vi "myRIO_BRig_RT_v0,83__PortC.vi"() -> ()   [LabVIEW 2014]
uses:
  myRIO_BRig_RT__Case_Exp_stateList.ctl
  myRIO_BRig_RT__Case_NonExp_stateList.ctl
  <vilib>/Platform/TimedLoop/XDataNode/timing_clust.ctl
  <vilib>/Platform/TimedLoop/XDataNode/nitl_modes.ctl
  <vilib>/Platform/TimedLoop/XDataNode/wakeup.ctl
  <vilib>/WebDAVClient/Advanced/SessionHandle.ctl
  <vilib>/myRIO/Common/Instrument Driver Framework/myRIO v1.0/UART/vis/myRIO v1.0 Close UART.vi
  <vilib>/FPGAPlugInAG/myRIO-1900/niLvFpga_Open_myRIO-1900.vi
  <vilib>/rvi/interface/common/dynamic/niFpgaDynamicAddResources.vi
  <vilib>/Utility/error.llb/Error Cluster From Error Code.vi
  <vilib>/rvi/errors/niLvFpgaAdjustHostInterfaceError.vi
  <vilib>/FPGAPlugInAG/Dynamic/niLvFpga_Close_Dynamic.vi
  <vilib>/myRIO/Common/Instrument Driver Framework/Utilities/vis/FPGA Ref Manager.vi
  <vilib>/myRIO/Common/Instrument Driver Framework/myRIO v1.0/myRIO v1.0 Reset FPGA.vi
  <vilib>/myRIO/Common/Instrument Driver Framework/myRIO v1.0/IRQ/vis/myRIO v1.0 IRQ Info FGV.vi
  <vilib>/myRIO/Common/Instrument Driver Framework/myRIO v1.0/IRQ/vis/myRIO v1.0 Timer IRQ Info FGV.vi
  <vilib>/myRIO/Common/Instrument Driver Framework/myRIO v1.0/IRQ/vis/myRIO v1.0 ISR Agent.vi
  <vilib>/rvi/interface/nirviOpenFPGA/nirviOpenFPGA.xnode
  myRIO_BRig_FPGA_v3,80__PortC__build.lvbitx
  myRIO_BRig_FPGA_v3,80__PortC.vi
  <vilib>/rvi/interface/nirviReadWriteControl/nirviReadWriteControl.xnode
  <vilib>/Platform/TimedLoop/XDataNode/XDataNode.xnode
  <vilib>/rvi/interface/nirviCloseFPGA/nirviCloseFPGA.xnode
  <vilib>/Platform/TimedLoop/XDataNode/XDNodeRunTimeDep.lvlib
  <vilib>/rvi/interface/Simulation/niFpgaSimulationCallBeginRW.vi
  <vilib>/myRIO/Instrument Drivers/Utilities/Utilities.lvlib
  <vilib>/WebDAVClient/NI_WebDAV.lvlib
  NiFpgaLv.dll
panel:
  out "allReward_R":bool
  out "allReward_L":bool
  in  "I_allReward":bool caption="NonSpecific Lick Direction"
  in  "Tcycle_Reward_max_R":u16=1000 caption="Max" min=5 max=5000 step=5
  in  "Tcycle_Reward_min_R":u16=1000 caption="Min" min=5 max=5000 step=5
  in  "Tcycle_Reward_step_R":u16=1000 caption="Penalty" min=1 max=10000 step=1
  in  "Tcycle_Reward_max_L":u16=1000 caption="Max" min=5 max=5000 step=5
  in  "Tcycle_Reward_min_L":u16=1000 caption="Min" min=5 max=5000 step=5
  in  "Tcycle_Reward_step_L":u16=1000 caption="Penalty" min=1 max=10000 step=1
  in  "MTrig_CueLed":bool
  out "Threshold":bool
  out "tLoop":dbl
  in  "Tcycle_Cue_LED_max":u16=1000 caption="Max" min=5 max=5000 step=5
  in  "Tcycle_Cue_LED_min":u16=1000 caption="Min" min=5 max=5000 step=5
  in  "Tcycle_CuePenalty_LED":u16=1000 caption="Penalty" min=1 max=10000 step=1
  out "power_l2":dbl
  in  "MTrig_Laser_Switch":bool
  in  "Cue1Param_AudioLed_Count_NS":u16
  in  "Cue1Param_AudioLed_Count_Switch":u16
  in  "Cue1Param_AudioLed_Probability_NS":u16
  in  "Cue1Param_CueType_NS":u16(slide) max=2 step=1 scale=0.0..2.0
  in  "Cue1Param_AudioLed_Probability_Switch":u16
  in  "Cue1Param_CueType_Switch":u16(slide) max=2 step=1 scale=0.0..2.0
  in  "CueLed_Freq":dbl=10.0
  in  "CueLed_Tpeak":dbl=2.0
  in  "Laser_power_step_l2":dbl
  in  "Laser_power_max_l2":dbl
  in  "Laser_power_min_l2":dbl
  in  "Laser_Tshutter_l2":dbl=2.0
  in  "Laser_Freq_l2":dbl=10.0
  in  "Laser_Tpeak_l2":dbl=2.0
  in  "Laser_duration_l2":u16
  in  "LC_Sel_Count_NS_l2":u16
  in  "LC_Sel_Count_Switch_l2":u16
  in  "LC_Sel_Probability_NS_l2":u16
  in  "LC_Sel_Block_NS_l2":u16(slide) max=2 step=1 scale=0.0..2.0
  in  "LC_Sel_OnOff_NS_l2":bool
  in  "LC_Sel_Probability_Switch_l2":u16
  in  "LC_Sel_Block_Switch_l2":u16(slide) max=2 step=1 scale=0.0..2.0
  in  "LC_Sel_OnOff_Switch_l2":bool
  in  "LC_Sel_Tdelay_NS_l2":u16
  in  "LC_Sel_Tdelay_Switch_l2":u16
  in  "LC_Cue1_Count_NS_l2":u16
  in  "LC_Cue1_Count_Switch_l2":u16
  in  "LC_Cue1_delayOpt_NS_l2":bool
  in  "LC_ENL1_delayOpt_NS_l2":bool
  in  "LC_ENL1_Count_NS_l2":u16
  in  "LC_ENL1_Count_Switch_l2":u16
  in  "LC_Cue1_delayOpt_Switch_l2":bool
  in  "LC_ENL1_delayOpt_Switch_l2":bool
  in  "LC_Cue1_Probability_NS_l2":u16
  in  "LC_Cue1_Block_NS_l2":u16(slide) max=2 step=1 scale=0.0..2.0
  in  "LC_Cue1_OnOff_NS_l2":bool
  in  "LC_Cue1_Probability_Switch_l2":u16
  in  "LC_Cue1_Block_Switch_l2":u16(slide) max=2 step=1 scale=0.0..2.0
  in  "LC_Cue1_OnOff_Switch_l2":bool
  in  "LC_ENL1_Probability_NS_l2":u16 max=100 step=1
  in  "LC_ENL1_Block_NS_l2":u16(slide) max=2 step=1 scale=0.0..2.0
  in  "LC_ENL1_OnOff_NS_l2":bool
  in  "LC_ENL1_Probability_Switch_l2":u16 max=100 step=1
  in  "LC_ENL1_Block_Switch_l2":u16(slide) max=2 step=1 scale=0.0..2.0
  in  "LC_Cue1_Tdelay_NS_l2":u16
  in  "LC_ENL1_Tdelay_NS_l2":u16
  in  "LC_Cue1_Tdelay_Switch_l2":u16
  in  "LC_ENL1_Tdelay_Switch_l2":u16
  in  "LC_ENL1_OnOff_Switch_l2":bool
  in  "LC_Wrong_Probability_l2":u16
  in  "LC_Wrong_Trial_l2":u16(slide) max=2 step=1 scale=0.0..2.0
  in  "LC_Wrong_Block_l2":u16(slide) max=2 step=1 scale=0.0..2.0
  in  "LC_Wrong_OnOff_l2":bool
  in  "LC_Reward_Probability_l2":u16
  in  "LC_Reward_Trial_l2":u16(slide) max=2 step=1 scale=0.0..2.0
  in  "LC_Reward_Block_l2":u16(slide) max=2 step=1 scale=0.0..2.0
  in  "LC_Reward_OnOff_l2":bool
  in  "LC_Wrong_Tdelay_l2":u16
  in  "LC_Reward_Tdelay_l2":u16
  in  "LC_Sel_Count_NS_l1":u16
  in  "LC_Sel_Count_Switch_l1":u16
  in  "LC_Sel_Probability_NS_l1":u16
  in  "LC_Sel_Block_NS_l1":u16(slide) max=2 step=1 scale=0.0..2.0
  in  "LC_Sel_OnOff_NS_l1":bool
  in  "LC_Sel_Probability_Switch_l1":u16
  in  "LC_Sel_Block_Switch_l1":u16(slide) max=2 step=1 scale=0.0..2.0
  in  "LC_Sel_OnOff_Switch_l1":bool
  in  "LC_Sel_Tdelay_NS_l1":u16
  in  "LC_Sel_Tdelay_Switch_l1":u16
  out "I_connect_TCP":bool
  in  "get_countPerMS":bool
  in  "count_warmup_R_reset":bool
  in  "count_warmup_L_reset":bool
  out "count_warmup_R":u16
  out "count_warmup_L":u16
  out "SolenoidReward":bool
  in  "SolenoidProbability_L":u16=100 caption="Reward Time [ms]" min=1 max=1000 step=1
  in  "SolenoidProbability_R":u16=100 caption="Reward Time [ms]" min=1 max=1000 step=1
  out "power_l1":dbl caption="LaserPower"
  in  "Laser_power_step_l1":dbl
  in  "Laser_power_max_l1":dbl
  in  "Recording":bool
  in  "Laser_power_min_l1":dbl
  in  "FPGA_count2ms":dbl=159.0
  in  "Laser_Tshutter_l1":dbl=2.0
  in  "Laser_Freq_l1":dbl=10.0
  in  "Laser_Tpeak_l1":dbl=2.0
  in  "Laser_duration_l1":u16
  out "error out":errorcluster
  in  "LC_Cue1_Count_NS_l1":u16
  in  "LC_Cue1_Count_Switch_l1":u16
  in  "LC_Cue1_delayOpt_NS_l1":bool
  in  "LC_ENL1_delayOpt_NS_l1":bool
  in  "LC_ENL1_Count_NS_l1":u16
  in  "LC_ENL1_Count_Switch_l1":u16
  in  "LC_Cue1_delayOpt_Switch_l1":bool
  in  "LC_ENL1_delayOpt_Switch_l1":bool
  in  "Tcycle_Cue_Audio_max":u16=1000 caption="Max" min=5 max=5000 step=5
  in  "Tcycle_Cue_Audio_min":u16=1000 caption="Min" min=5 max=5000 step=5
  in  "SendData":bool
  out "cSpout":enum16{"Left", "Right"}(ring) caption="Left or Right Spout"
  out "A4":u32 caption="LickCounter_Right"
  out "A2":u32 caption="LickCounter_Left"
  in  "LR_wrong_Event":bool
  out "SelectWrong":bool
  out "SelectReward":bool
  in  "Left(F)_or_Right(T)":bool
  in  "ignoreWrong":bool
  in  "SelectionState":bool
  in  "LR_wrong_Laser":bool
  in  "LR_reward_Laser":bool
  in  "LR_reward_Event":bool
  out "nRewards_Right":u16 caption="# Rewards Total (Right)"
  out "nRewards_Left":u16 caption="# Rewards Total (Left)"
  out "nRewards_cur":u16 caption="# Rewards in Current Block"
  out "TpB_target":u16 caption="Target Trials Per Block"
  out "cState_NonExp":T1 caption="WarmUp State"
  out "iBlock":u16 caption="Current Block"
  out "cState":T2 caption="Experimental State"
  out "iTrial":u16 caption="Current Trial"
  in  "warmupType":u8(slide) max=2 step=1 scale=0.0..2.0
  in  "TestConnection":bool
  in  "warmup":bool caption="WarmUp"
  in  "Data Set Prefix":string="Exp1_TM2"
  out "Connected To Host?":bool
  in  "Host Password":string="sabalab"
  in  "Host UserName":string="Test2"
  in  "sp_RightSpout":u16(slide)=2 max=2 step=1 scale=0.0..2.0
  in  "sp_LeftSpout":u16(slide)=2 max=2 step=1 scale=0.0..2.0
  in  "BUR_max":u16 caption="Count Reward Structure  (0 = off)"
  in  "LC_Wrong_Probability_l1":u16
  in  "LC_Wrong_Trial_l1":u16(slide) max=2 step=1 scale=0.0..2.0
  in  "LC_Wrong_Block_l1":u16(slide) max=2 step=1 scale=0.0..2.0
  in  "LC_Wrong_OnOff_l1":bool
  in  "LC_Reward_Probability_l1":u16
  in  "LC_Reward_Trial_l1":u16(slide) max=2 step=1 scale=0.0..2.0
  in  "LC_Reward_Block_l1":u16(slide) max=2 step=1 scale=0.0..2.0
  in  "LC_Reward_OnOff_l1":bool
  in  "LC_Cue1_Probability_NS_l1":u16
  in  "LC_Cue1_Block_NS_l1":u16(slide) max=2 step=1 scale=0.0..2.0
  in  "LC_Cue1_OnOff_NS_l1":bool
  in  "LC_Cue1_Probability_Switch_l1":u16
  in  "LC_Cue1_Block_Switch_l1":u16(slide) max=2 step=1 scale=0.0..2.0
  in  "LC_Cue1_OnOff_Switch_l1":bool
  in  "LC_ENL1_Probability_NS_l1":u16 max=100 step=1
  in  "LC_ENL1_Block_NS_l1":u16(slide) max=2 step=1 scale=0.0..2.0
  in  "LC_ENL1_OnOff_NS_l1":bool
  in  "LC_ENL1_Probability_Switch_l1":u16 max=100 step=1
  in  "LC_ENL1_Block_Switch_l1":u16(slide) max=2 step=1 scale=0.0..2.0
  in  "Tcycle_Timeout":u16=1000 caption="Timeout Time [ms]" min=10 max=10000 step=1
  in  "Tcycle_Wrong":u16=1000 caption="Wrong Time [ms]" min=10 max=10000 step=1
  in  "Tcycle_Selection":u16=1000 caption="Answer Time [ms]" min=1 max=10000 step=1
  in  "Tcycle_RewardPost":u16=1000 caption="Consumption Time [ms]" min=250 max=10000 step=250
  in  "TpB_Max_R":u16=4 caption="Max TrialsPerBlock" min=1 max=12 step=1
  in  "TpB_Min_R":u16=4 caption="Min TrialsPerBlock" min=1 max=12 step=1
  in  "TpB_Max_L":u16=4 caption="Max TrialsPerBlock" min=1 max=12 step=1
  in  "TpB_Min_L":u16=4 caption="Min TrialsPerBlock" min=1 max=12 step=1
  in  "BUR_min":u16 caption="Count Reward Structure\n(0 = off)"
  in  "TrialUntilReward":bool caption="Ignore Wrong Selection"
  in  "CueCycles":u16=1 caption="Cue Structure" min=1 max=1 step=1
  in  "MTrig_Laser_Tcycle":u16=10 caption="Time [ms]"
  in  "MTrig_Laser_trig":bool
  in  "MTrig_Audio_trig__R":bool caption="Trigger Audio"
  in  "MTrig_Audio_trig__L":bool caption="Trigger Audio"
  in  "RewCalib_Trig_R":bool caption="Calibrate_R"
  in  "RewCalib_Trig_L":bool caption="Calibrate_L"
  in  "MTrig_Solenoid_Tcycle__R":u16=300 caption="Time [ms]"
  in  "MTrig_Solenoid_Tcycle__L":u16=300 caption="Time [ms]"
  in  "MTrig_Solenoid_trig__R":bool caption="Solenoid"
  in  "MTrig_Solenoid_trig__L":bool caption="Solenoid"
  in  "STOP_abort":bool caption="Stop LabView\n(Stops myRio and FPGA)"
  in  "STOP_endBlock":bool caption="Stop Experiment\n@ End of Block"
  in  "STOP_endTrial":bool caption="Stop Experiment\n@ End of Trial"
  in  "START":bool caption="Start Experiment"
  in  "Tcycle_CuePenalty_Audio":u16=1000 caption="Penalty" min=1 max=10000 step=1
  in  "Audio_Amp__R":u16=100 caption="Amp"
  in  "Audio_Freq__R":u8=5 caption="Freq [kHz]" max=14 step=1
  in  "Audio_Amp__L":u16=100 caption="Amp"
  in  "Audio_Freq__L":u8=5 caption="Freq [kHz]" max=14 step=1
  in  "LC_Wrong_Tdelay_l1":u16
  in  "LC_Cue1_Tdelay_NS_l1":u16
  in  "LC_ENL1_Tdelay_NS_l1":u16
  in  "LC_Reward_Tdelay_l1":u16
  in  "LC_Cue1_Tdelay_Switch_l1":u16
  in  "LC_ENL1_Tdelay_Switch_l1":u16
  in  "LC_ENL1_OnOff_Switch_l1":bool
  in  "Tcycle_ENLPenalty":u16=100 caption="Penalty" min=10 max=10000 step=10
  in  "Tcycle_ENL_max":u16=1000 caption="Max" min=250 max=10000 step=250
  in  "Tcycle_ENL_min":u16=1000 caption="Min" min=250 max=10000 step=250
  # "Communication (Host PC)"
  # "Recording Rig"
  # "Experimental Run"
  # "Experiment Task Structure"
  # "STOP experiment at"
  # "Min            Max            Penalty"
  # "(1) = Switching\n(2) = Two Choice"
  # "Enforced\nNonLick"
  # "FPGA Count per [ms]"
  # "Cue Audio"
  # "Current State"
  # "Cue LED"
  # "Global Parameters                                                         Trial Parameters"
  # "Selection"
  # "WarmUp"
  # "Reward - Dispense Water"
  # "Left/Right        Give Reward?        Laser Power [V]"
  # "Laser1      Laser2"
  # "Left"
  # "Cue then reward (no lick)\n \nLeft                    Right"
  # "Right"
  # "Min"
  # "Max"
  # "Dispense Water Probability"
  # "Block                   Trial            Target Trials       # Rewards \n                                                            Per Block             Current"
  # "Left"
  # "WarmUp State"
  # "Trial Per Block Structure \n               Left                        Right"
  # "Lick Counter"
  # "Right"
  # "Left           Right"
  # "Reward - Consumption"
  # "Manual Control"
  # "Min"
  # "# Rewards Total\n                                                                  Left                    Right"
  # "Experimental State"
  # "Penalty - Wrong Choice"
  # "Solenoid\n \nLeft              Right"
  # "Speaker\n \nLeft                    Right"
  # "Laser 1  |  Laser 2"
  # "Max"
  # "Penalty - Choice Timeout"
  # "Time\n[ms]"
  # "Time\n[ms]"
  # "Time = Cue Min"
  # "Cue LED"
  # "Power = Min"
  # "Cue1 Control\n                                  Cue Type           LED Probability [%]      Count"
  # "Laser1 Control\n                               On/Off      Block        Probability [%]   Delay [ms]                              Count"
  # "Laser2 Control\n                               On/Off      Block        Probability [%]   Delay [ms]                              Count"
  # "Audio or LED"
  # "Cue 1"
  # "Enforced\nNonLick\n      1"
  # "Enforced\nNonLick\n      1"
  # "from end"
  # "from end"
  # "Switch\nTrial"
  # "Switch\nTrial"
  # "Switch\nTrial"
  # "from start"
  # "from start"
  # "from end"
  # "from end"
  # "NonSwitch\nTrials"
  # "NonSwitch\nTrials"
  # "NonSwitch\nTrials"
  # "from start"
  # "from start"
  # "Cue 1"
  # "Cue 1"
  # "from end"
  # "from end"
  # "Switch\nTrial"
  # "Switch\nTrial"
  # "Cue Audio Parameters"
  # "Cue LED Parameters"
  # "from start"
  # "from start"
  # "Left                  Right"
  # "Frequency\n[Hz]"
  # "Frequency\n[kHz]"
  # "from end"
  # "from end"
  # "NonSwitch\nTrials"
  # "NonSwitch\nTrials"
  # "Timing [ms]\n                    Peak Width"
  # "from start"
  # "from start"
  # "Amp\n(0 - 32,000)"
  # "Selection"
  # "Selection"
  # "from start"
  # "from start"
  # "Switch\nTrial"
  # "Switch\nTrial"
  # "Speaker\nPattern\nDuring Cue"
  # "from start"
  # "from start"
  # "NonSwitch\nTrials"
  # "NonSwitch\nTrials"
  # "Laser1 Parameters"
  # "Laser2 Parameters"
  # "Laser1 Response\n                               On/Off      Block       Trial       Probability [%]   Delay [ms]"
  # "Laser2 Response\n                               On/Off      Block       Trial       Probability [%]   Delay [ms]"
  # "Frequency\n[Hz]"
  # "Frequency\n[Hz]"
  # "Timing [ms]\n Duration     Peak Width   Shutter"
  # "Timing [ms]\n Duration     Peak Width   Shutter"
  # "Selection Reward"
  # "Selection Reward"
  # "Laser Power [V]\nMin          Max              Step"
  # "Laser Power [V]\nMin          Max              Step"
  # "Selection Wrong"
  # "Selection Wrong"
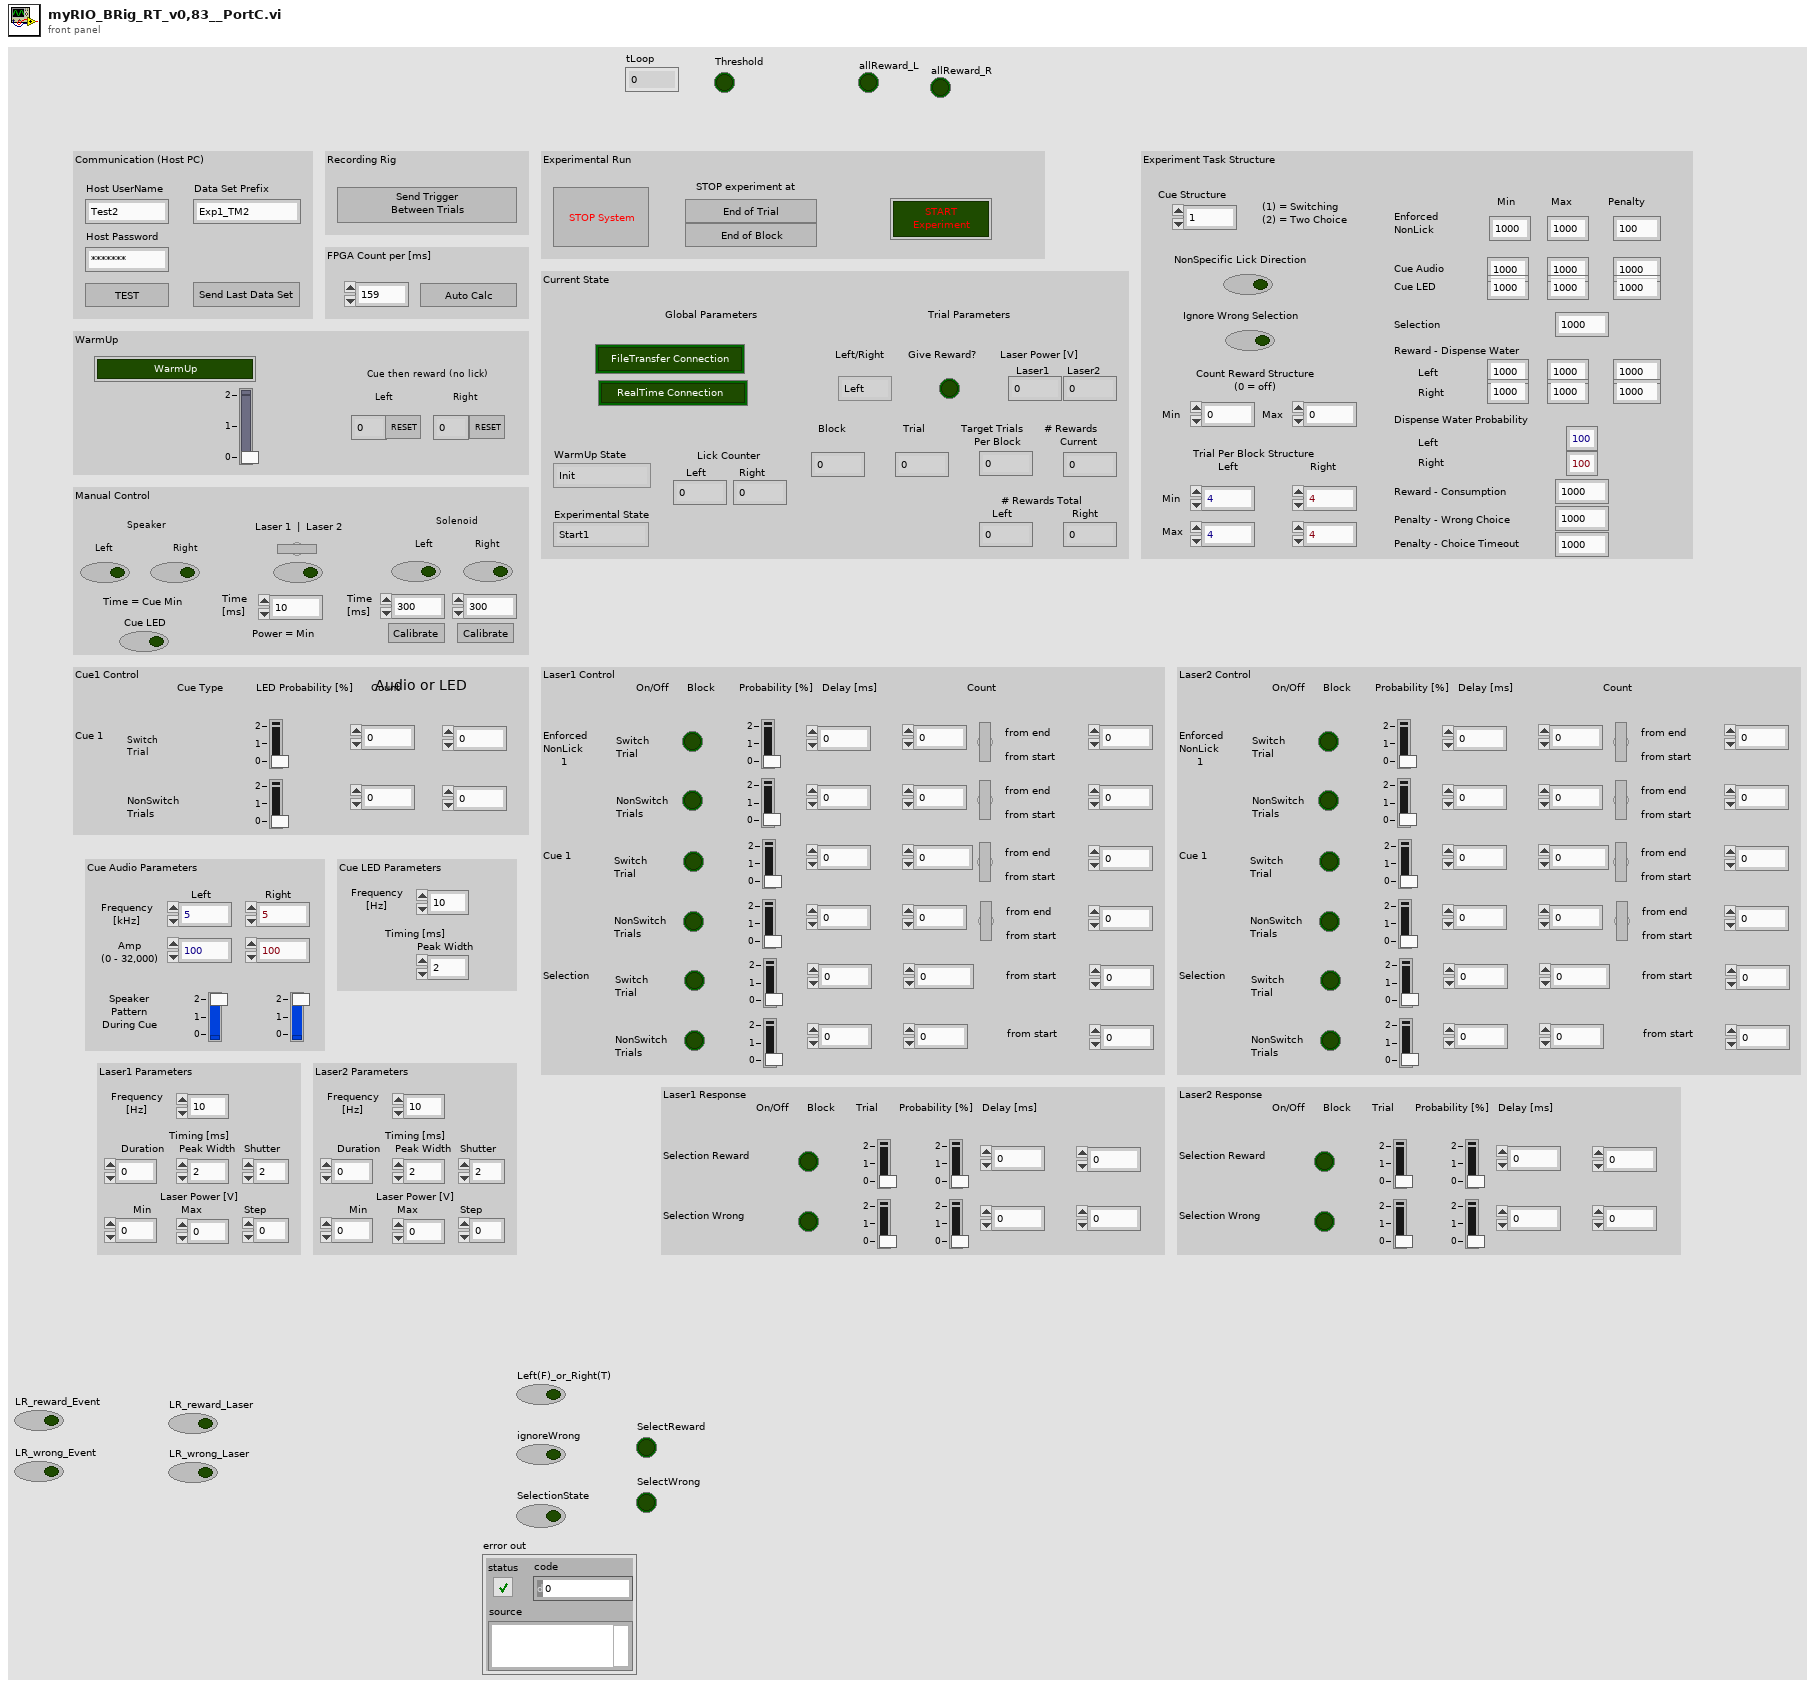
[diagram p1: front panel]
types:
  T1 = typedef "myRIO_BRig_RT__Case_NonExp_stateList.ctl" = enum16{"Init", "UploadSettings_pre", "UploadSettings_Read_dataExp", "UploadSettings_dataExp_1", "UploadSettings_dataExp_2", "UploadSettings_Read_dataLC", "UploadSettings_dataLC_1", "UploadSettings_dataLC_2", "UploadSettings_dataLC_3", "UploadSettings_dataLC_4", "UploadSettings_Read_dataMTrig", "UploadSettings_dataMTrig_1", "UploadSettings_post", "Idle_pre", "IdleEmpty", "IdleEmpty2", "IdleEmpty3", "IdleEmpty4", "Idle", "Idle_2", "Idle_3", "Idle_4", "Idle_5", "Idle_6", "Idle_post", "Cue_pre__pre", "Cue_pre", "Cue", "Cue_LED", "Cue_post", "RewardCalibration_pre", "DispenseWater_pre__pre", "DispenseWater_pre", "DispenseWater", "DispenseWater_post", "TestConnection", "SendData", "Get_FPGA_count_per_ms", "End"}
  T2 = typedef "myRIO_BRig_RT__Case_Exp_stateList.ctl" = enum16{"Start1", "Start2", "Start3", "saveSettings1", "saveSettings2", "saveSettings3", "saveSettings4", "saveSettings_LC_ENL_l1", "saveSettings_LC_ENL_l2", "saveSettings_LC_Cue_l1", "saveSettings_LC_Cue_l2", "saveSettings6_LC_l1_Other", "SaveSettings6_LC_l2_Other", "setSettings_Audio", "setSettings_Laser", "initBlock_pre", "initBlock", "initBlock2", "initBlock_post", "initTrial_pre", "initTrial", "initTrial2", "initTrial3", "initTrial4", "initTrial_LC_ENL1", "initTrial_LC_Cue1", "initTrial_LC_Cue1_2", "initTrial_LC_Sel", "initTrial_post", "ENL1_pre", "ENL1", "ENL1_post", "ENL1Penalty_pre", "ENL1Penalty", "ENL2_pre", "ENL2", "ENL2Penalty_pre", "ENL2Penalty", "Cue1_pre", "Cue1", "Cue1_post", "Cue1Penalty_pre", "Cue1Penalty", "Cue2_pre", "Cue2", "Cue2Penalty_pre", "Cue2Penalty", "Selection_pre", "Selection", "Select_post", "SelectReward_pre", "SelectReward", "SelectRewardPost_pre", "SelectRewardPost", "SelectWrong_pre", "SelectWrong", "SelectWrong_post", "SelectTimeout_pre", "SelectTimeout", "SelectTimeout_post", "endTrial_pre", "endTrial1", "endTrial2", "endTrial3", "endTrial_post", "endBlock_pre", "endBlock", "endBlock_post", "endExp", "commConnect", "commUpload_pre", "commUpload_dataBlock", "commUpload_dataCurrent", "commUpload_dataExp", "commUpload_dataLC", "commUpload_dataTrial", "commUpload_post", "saveData_pre", "saveData_dataBlock", "saveData_dataCurrent", "saveData_dataExp", "saveData_dataLC", "saveData_dataTrial", "saveData_post", "empty_endBlock1", "empty_endBlock2", "empty_endTrial1", "empty_endTrial2", "empty_endTrial3", "empty_endTrial4", "empty_endTrial5", "dummyState", "dummyState_endBlock"}
  T3 = typedef "XDNodeRunTimeDep.lvlib/timing_clust.ctl" = cluster{"Expected End [f-1]":u64, "Actual End [f-1]":u64, "Finished Late? [f-1]":bool, "Expected End [i-1]":u64, "Actual End [i-1]":u64, "Finished Late? [i-1]":bool, "Expected Start [i]":u64, "Actual Start [i]":u64, "Expected Start [f]":u64, "Actual Start [f]":u64, "Source Name":string, "Structure Name":string, "Period":i64, "Deadline":i64, "Offset":i64, "Start":i64, "Priority":i32, "Timeout":i32, "Mode":T4, "Wakeup Reason":T5, "Error":errorcluster, "Source Type":string, "Secondary Source Type":string, "Global End Time":u64, "Global Start Time":u64, "Frame Duration":u64, "Iteration Duration":u64, "Assigned CPU":i32, "I/O Scan Engine Mode":u32}
  T4 = typedef "XDNodeRunTimeDep.lvlib/nitl_modes.ctl" = enum32{"No Change", "Process missed periods, maintain original phase", "Discard missed periods, maintain original phase", "Process missed periods, ignore original phase", "Discard missed periods, ignore original phase"}
  T5 = typedef "XDNodeRunTimeDep.lvlib/wakeup.ctl" = enum32{"Normal", "Aborted", "Asynchronous wakeup", "Timing source error", "Timed loop error", "Timeout"}
  T6 = typedef "NI_WebDAV.lvlib/SessionHandle.ctl" = refnum<k1>
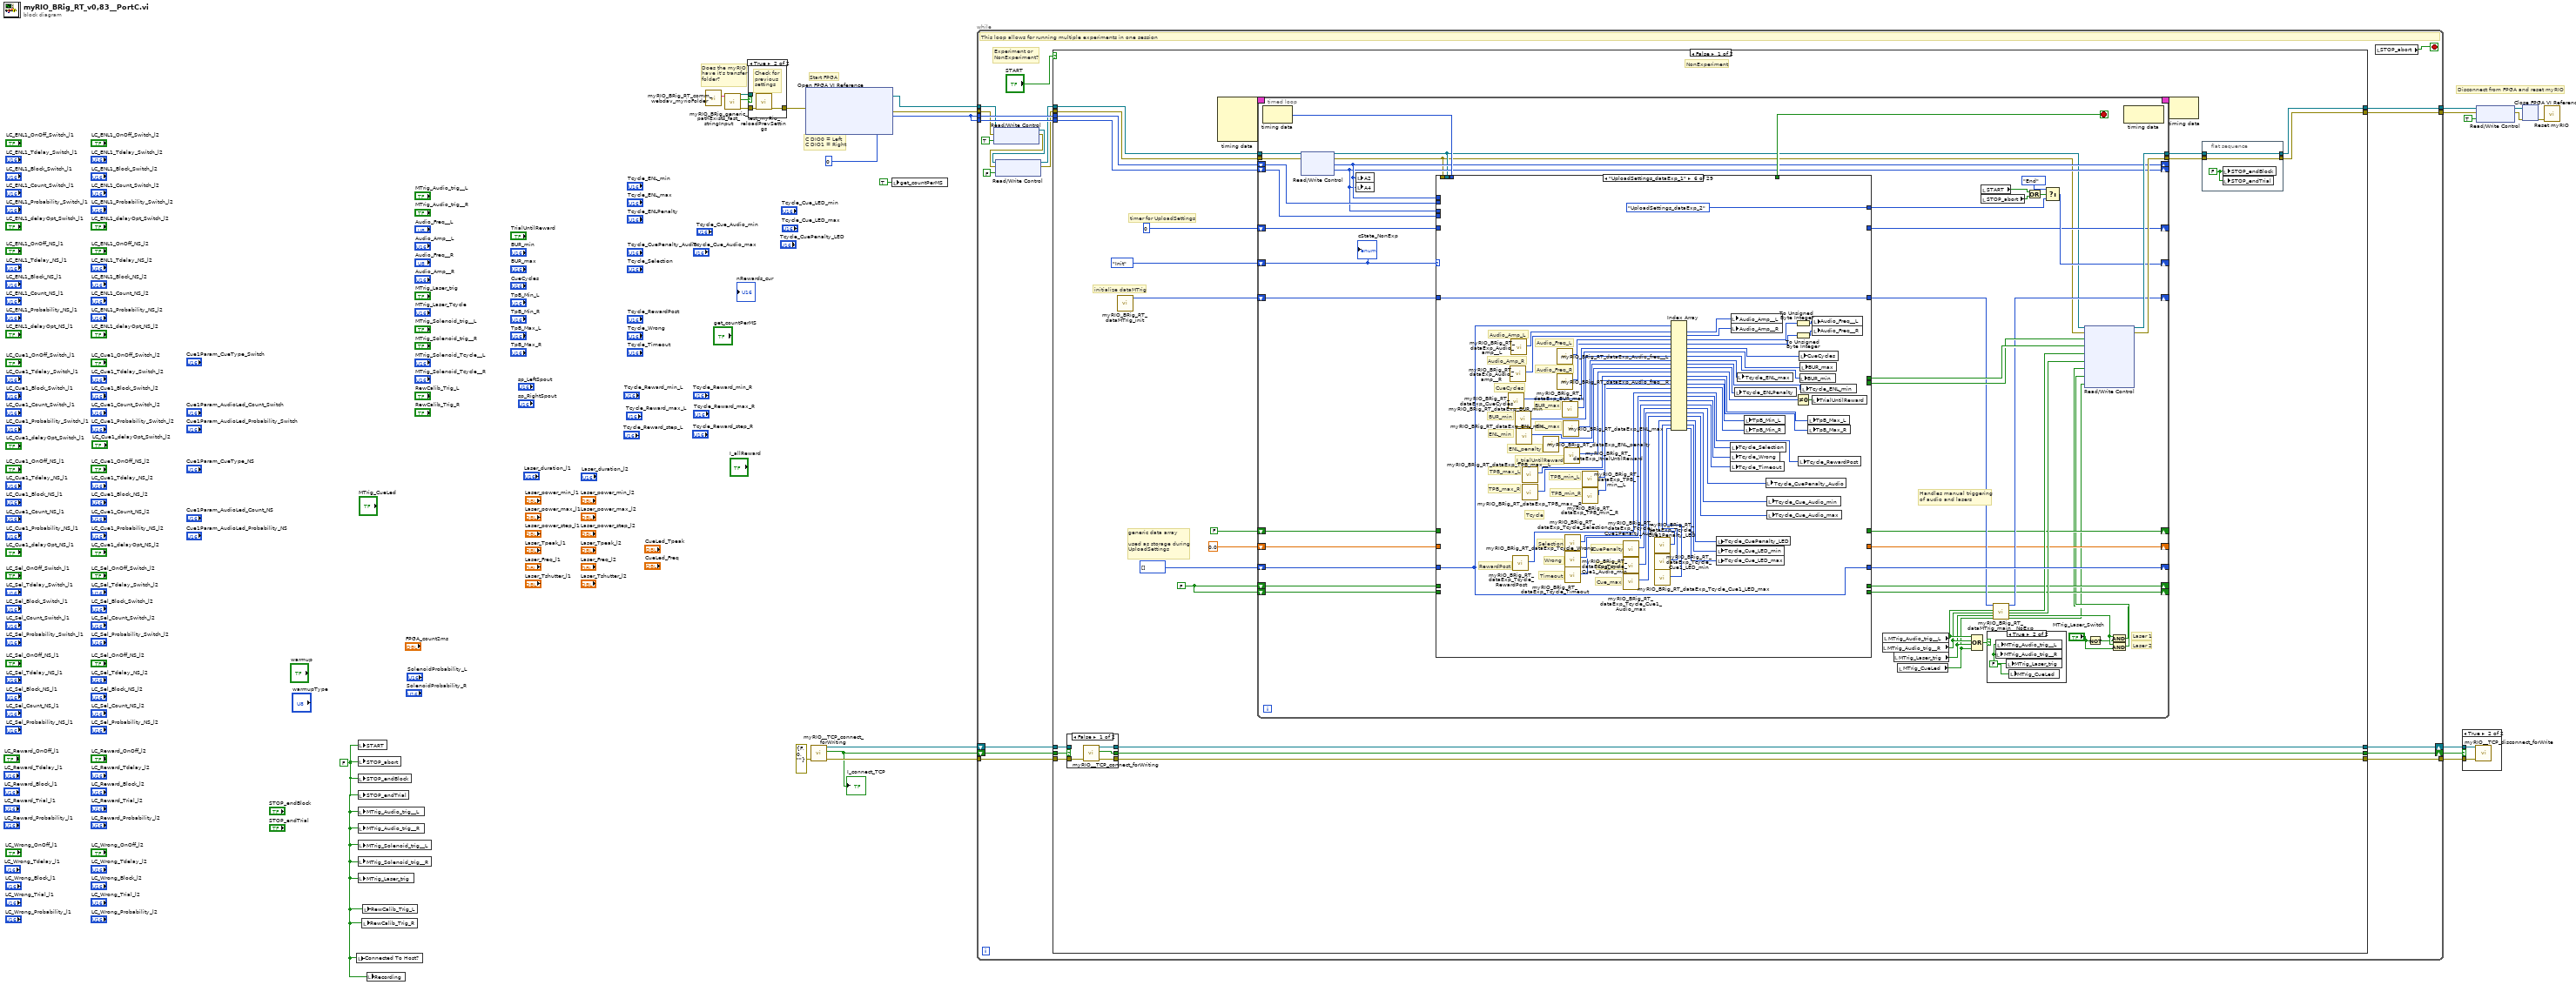
[diagram p0: block diagram]
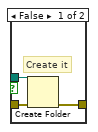
[diagram p3: hidden frame]
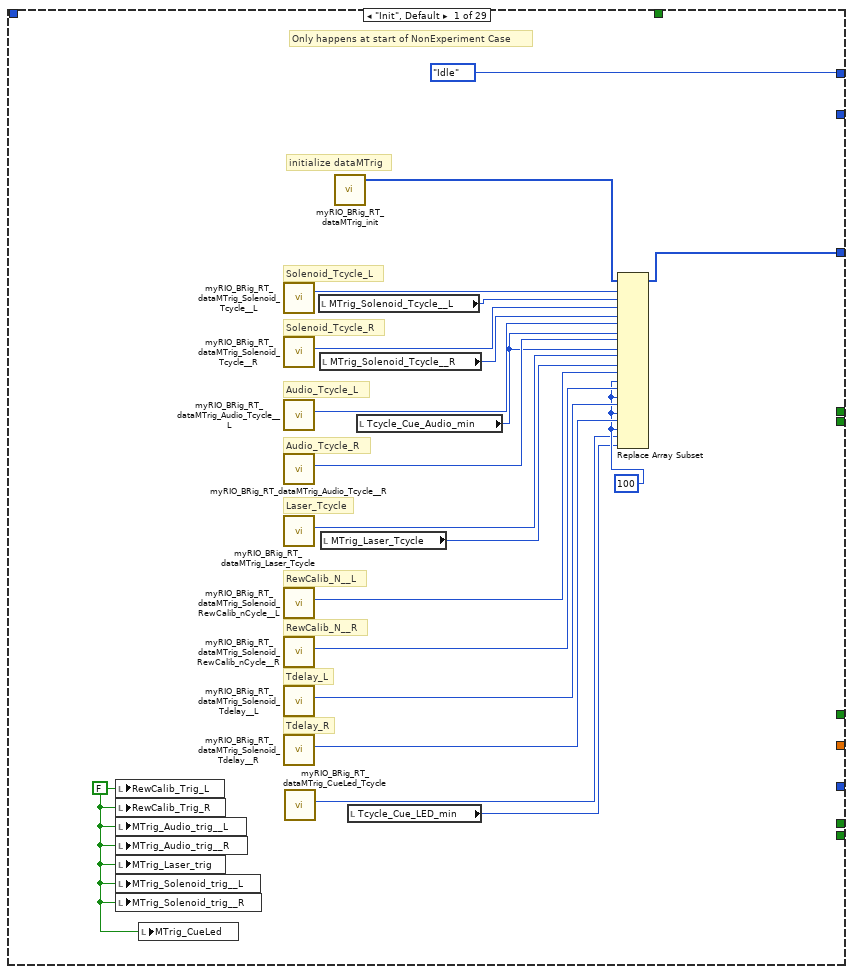
[diagram p6: hidden frame]
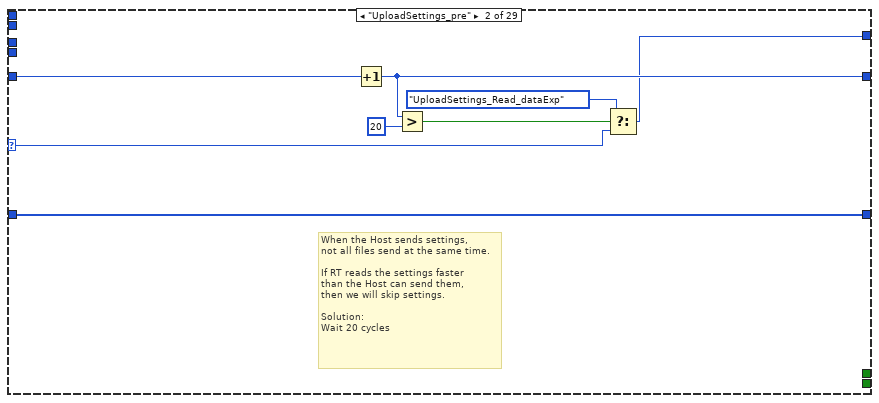
[diagram p7: hidden frame]
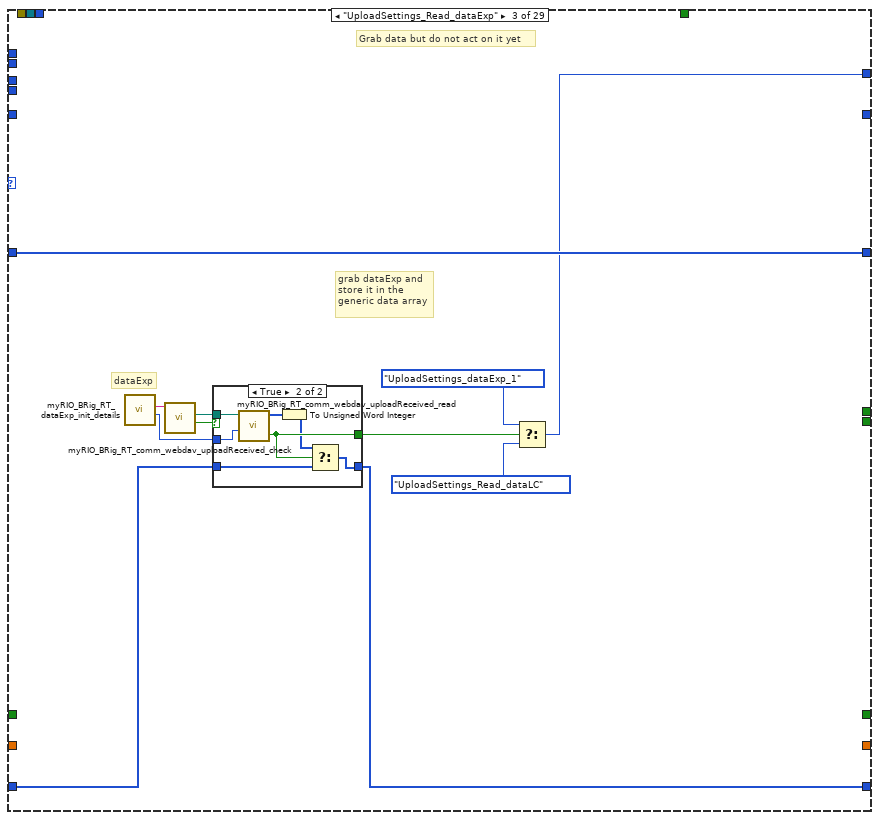
[diagram p8: hidden frame]
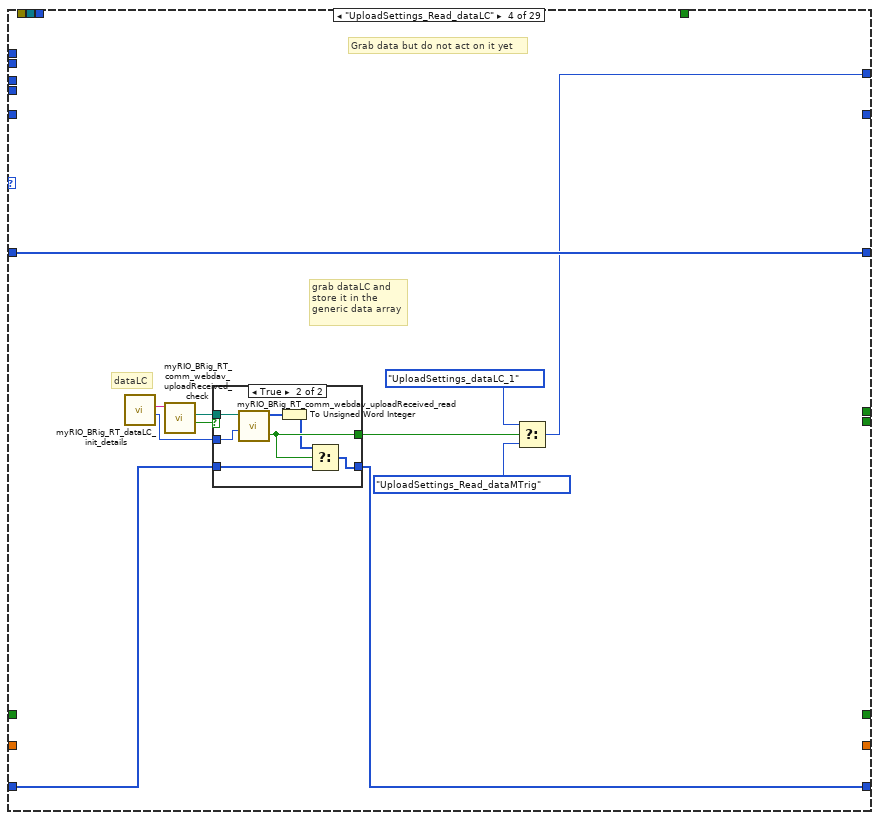
[diagram p10: hidden frame]
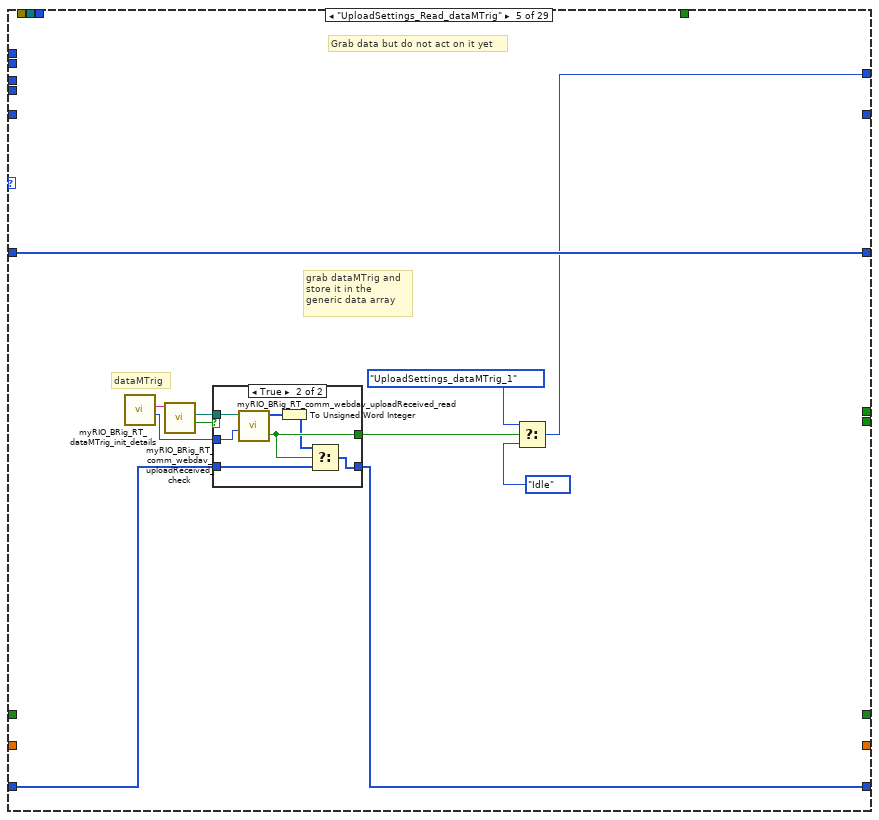
[diagram p12: hidden frame]
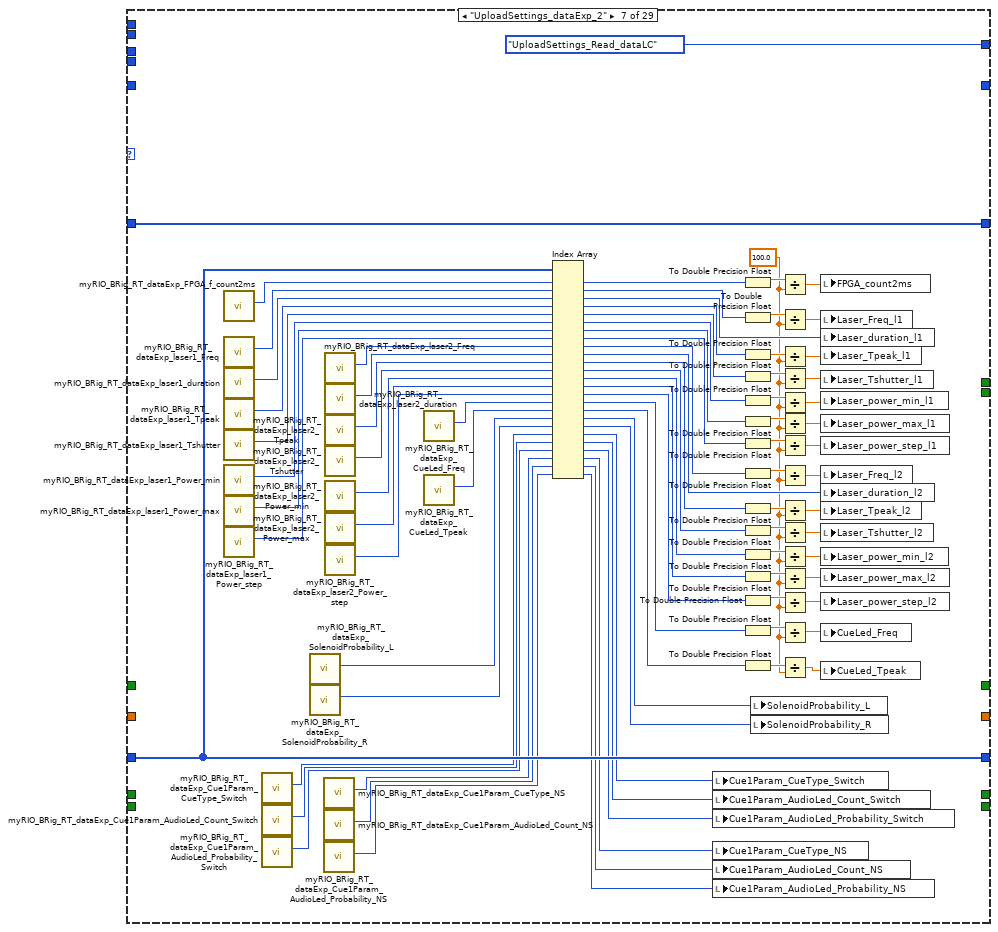
[diagram p14: hidden frame]
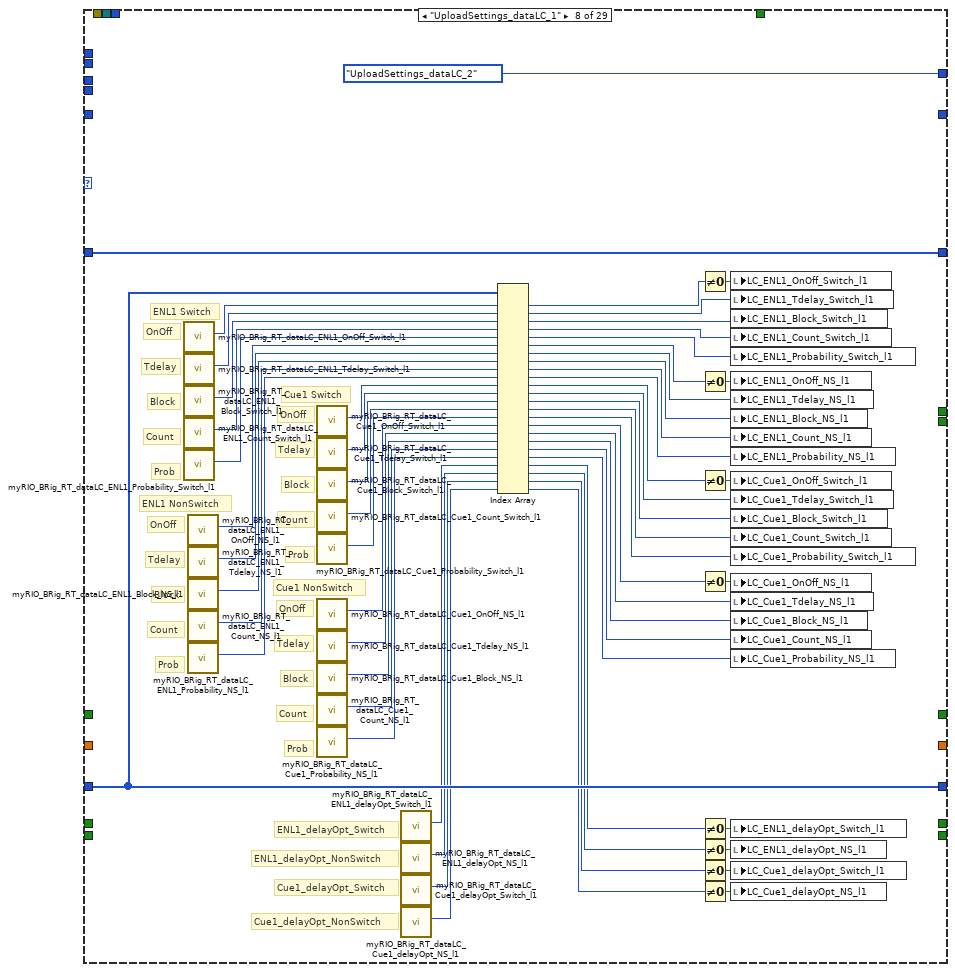
[diagram p15: hidden frame]
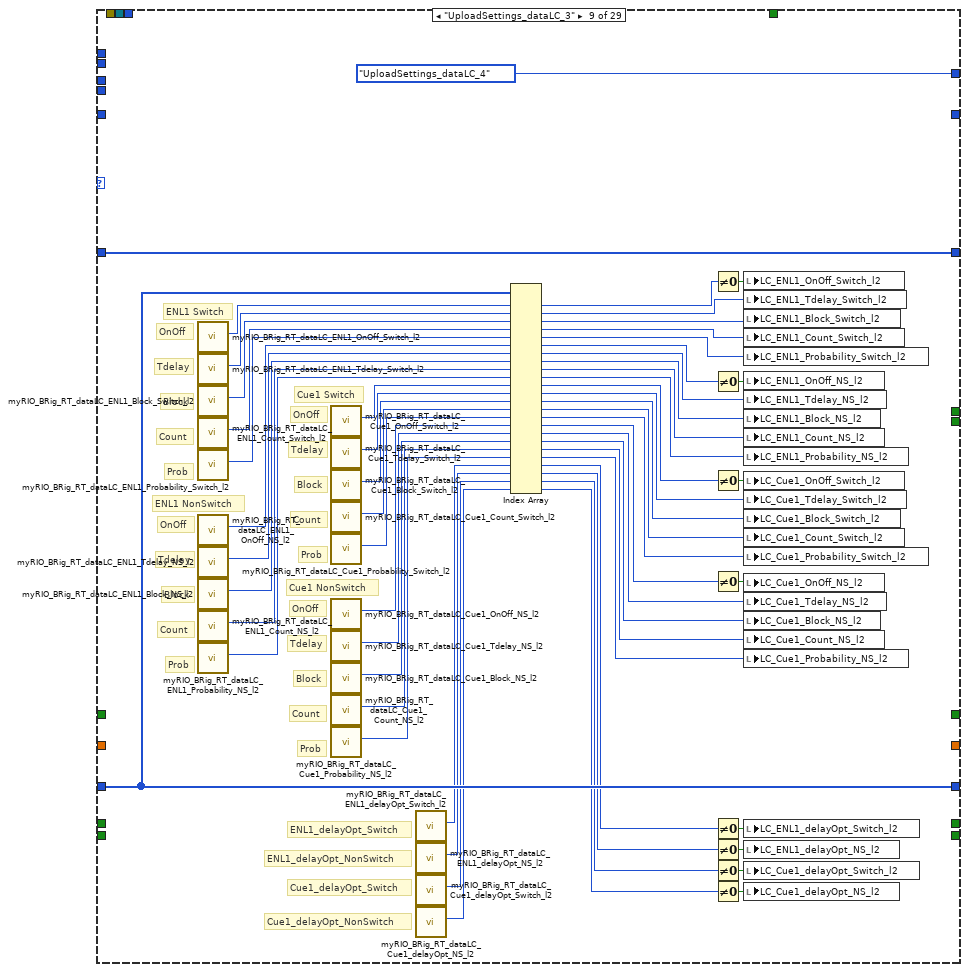
[diagram p16: hidden frame]
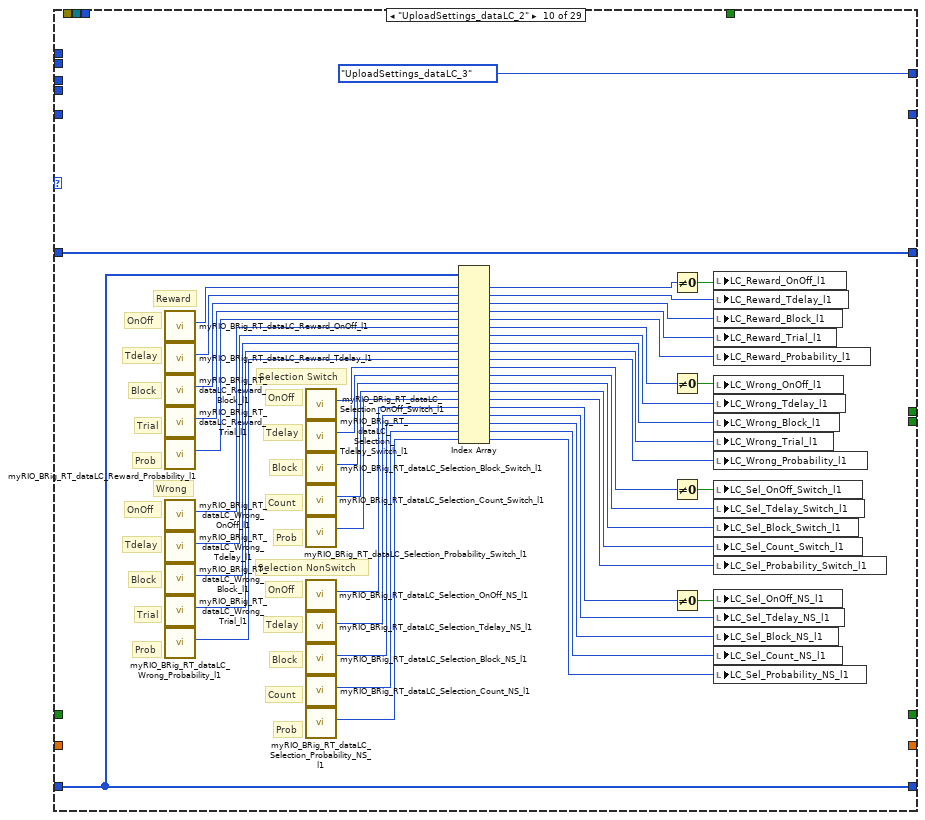
[diagram p17: hidden frame]
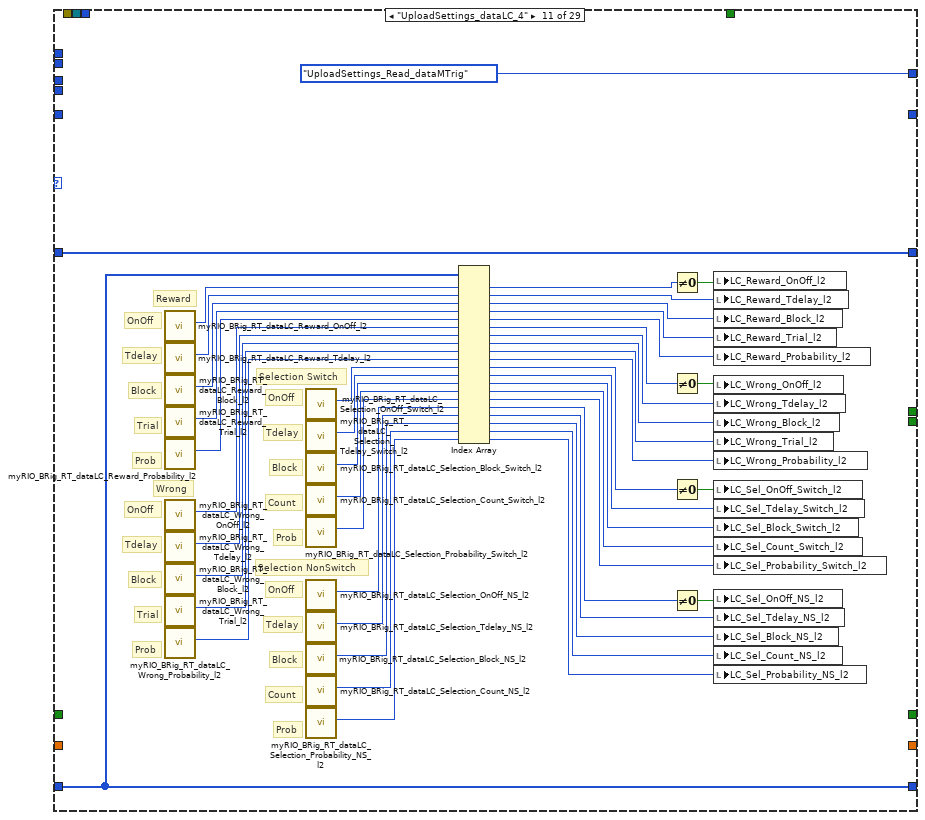
[diagram p18: hidden frame]
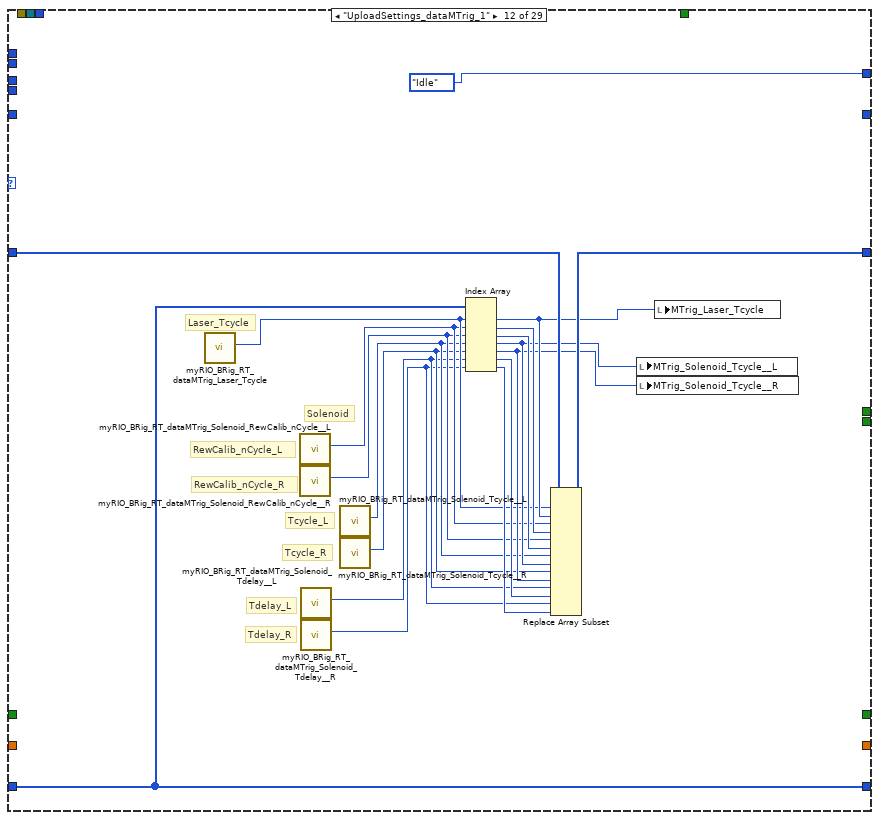
[diagram p19: hidden frame]
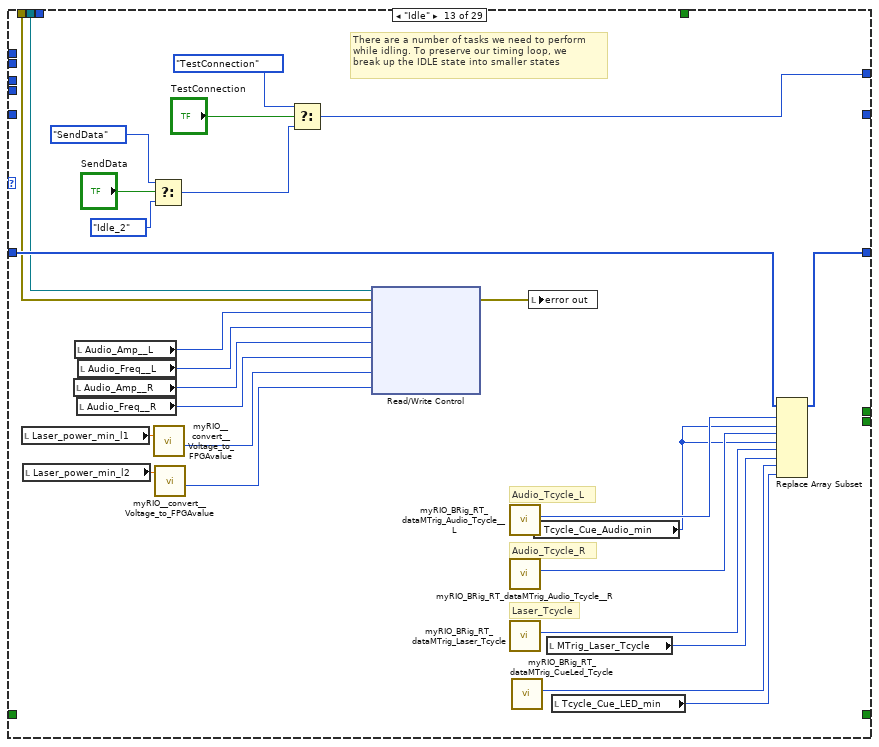
[diagram p20: hidden frame]
diagram:
  w17 = u32 0
  w1 = FALSE
  # "Does the myRIO\nhave it's transfer\nfolder?"
  # "C DIO0 = Left\nC DIO1 = Right"
  # "Start FPGA"
  # "Disconnect from FPGA and reset myRIO"
  n1 = local write "Connected To Host?"(w1) -> ()
  n2 = local write "START"(w1) -> ()
  n3 = local write "STOP_abort"(w1) -> ()
  n4 = local write "STOP_endBlock"(w1) -> ()
  n5 = local write "STOP_endTrial"(w1) -> ()
  n6 = local write "MTrig_Audio_trig__L"(w1) -> ()
  n7 = local write "MTrig_Audio_trig__R"(w1) -> ()
  n8 = local write "MTrig_Solenoid_trig__L"(w1) -> ()
  n9 = local write "MTrig_Solenoid_trig__R"(w1) -> ()
  n10 = local write "MTrig_Laser_trig"(w1) -> ()
  n11 = local write "RewCalib_Trig_R"(w1) -> ()
  n12 = local write "RewCalib_Trig_L"(w1) -> ()
  n13 = local write "Recording"(w1) -> ()
  n14 = call "myRIO_BRig_RT_comm_webdav_myrioFolder.vi"() -> ("output_myrioFolder"=w14:string)  [unwired: 11 in]
  n15 = call "myRIO_BRig_generic_pathExists_fast_stringInput.vi"("input_filePath"=w14) -> ("output_error"=w13:errorcluster, "output_Iexist"=w12:bool, "output_filePath"=w11:path)  [unwired: 8 in]
  n16 = case shown="True" w12 {
    tunnel: w11 -> [w26 _]
    tunnel: w13 -> [w25 w28]
    tunnel: [w24 w27] -> w9
    frame False {
      # "Create it"
      n17 = Create Folder(path (use dialog)=w26, error in=w25) -> (error out=w24:errorcluster)  [unwired: 1 in, 2 out]
    }
    frame True {
      # "Check for\nprevious\nsettings"
      n18 = call "test_myRio_reloadPrevSettings.vi"("input_error"=w28) -> ("output_error"=w27:errorcluster)  [unwired: 10 in]
    }
  }
  n19 = xnode "Open FPGA VI Reference"("error in"=w9) -> ("FPGA VI Reference Out"=w19:refnum<k20>, "error out"=w18:errorcluster)  [unwired: 1 in]
  n20 = call "myRIO__TCP_connect_forWriting.vi"("input_error"=errorcluster {"status"=FALSE, "code"=0, "source"=""}) -> ("output_error"=w7:errorcluster, "output_connected"=w6:bool, "output_hTCP"=w10:refnum<k5>)  [unwired: 8 in]
  "I_connect_TCP" <- w6
  n21 = local write "get_countPerMS"(TRUE ("get_countPerMS")) -> ()
  n22 = while {
    tunnel: w19 -> [w38]
    tunnel: w18 -> [w43]
    tunnel: w17 -> [w46]
    tunnel: w17 -> [w45]
    tunnel: [w36] -> w16
    tunnel: [w35] -> w15
    shift-right: [w32] -> w5
    shift-left: w6 -> [w33]
    tunnel: w7 -> [w31]
    shift-right: [w30] -> w4
    shift-left: w10 -> [w34]
    tunnel: [w29] -> w3
    stop <- w44 stop-if-true
    # "Experiment or\nNonExperiment?"
    # "This loop allows for running multiple experiments in one session"
    n23 = xnode "Read/Write Control"("FPGA VI Reference In"=w38, "error in"=w43, "Counts_Reset"=TRUE) -> ("FPGA VI Reference Out"=w40:refnum<k20>, "error out"=w41:errorcluster)
    n24 = xnode "Read/Write Control"("FPGA VI Reference In"=w40, "error in"=w41, "Counts_Reset"=FALSE) -> ("FPGA VI Reference Out"=w37:refnum<k20>, "error out"=w39:errorcluster)
    n25 = case shown="False" "START" {
      tunnel: w46 -> [w67 w1510]
      tunnel: w45 -> [w66 w1509]
      tunnel: w39 -> [w64 w1444]
      tunnel: w37 -> [w65 w1445]
      tunnel: [w62 w1506] -> w36
      tunnel: [w60 w1501] -> w35
      tunnel: w34 -> [w53 w1455]
      tunnel: [w51 w1459] -> w30
      tunnel: w33 -> [w52 w1457]
      tunnel: [w50 w1458] -> w32
      tunnel: w31 -> [w54 w1456]
      tunnel: [w49 w1454] -> w29
      frame False {
        w57 = FALSE
        # "generic data array\n\nused as storage during\nUploadSettings"
        # "timer for UploadSettings"
        # "initialize dataMTrig"
        # "NonExperiment"
        n26 = case shown="False" w52 {
          selector: w52 -> [_ w76]
          tunnel: w54 -> [w73 w78]
          tunnel: [w74 w78] -> w49
          tunnel: w53 -> [_ w77]
          tunnel: [w75 w77] -> w51
          tunnel: [w72 w76] -> w50
          frame False {
            n27 = call "myRIO__TCP_connect_forWriting.vi"("input_error"=w73) -> ("output_error"=w74:errorcluster, "output_connected"=w72:bool, "output_hTCP"=w75:refnum<k5>)  [unwired: 8 in]
          }
          frame True {
          }
        }
        n28 = call "myRIO_BRig_RT_dataMTrig_init.vi"() -> ("output_dataMTrig"=w68:u16[])  [unwired: 5 in]
        n29 = node-c288() -> (w71:T3)  [unwired: 4 in]
        n30 = timed-loop {
          timing: w71 -> [_]
          timing-out: [_] -> w70
          shift-right: [w117] -> _
          shift-left: w68 -> [w129]
          shift-right: [w111] -> _
          shift-left: myRIO_BRig_RT__Case_NonExp_stateList."Init" ("Enum") -> [w123]
          shift-right: [w105] -> _
          shift-left: w67 -> [w106]
          shift-right: [w103] -> _
          shift-left: w66 -> [w104]
          tunnel: [w125] -> w63
          tunnel: [w124] -> w61
          tunnel: w64 -> [w127]
          tunnel: w65 -> [w126]
          shift-right: [w122] -> _
          shift-left: u16[] [] ("output_data") -> [w121]
          shift-right: [w107] -> _
          shift-left: u16 0 ("Audio_Amp__L") -> [w108]
          shift-right: [w100] -> _
          shift-left: w57 -> [w102]
          shift-right: [w99] -> _
          shift-left: w57 -> [w101]
          shift-right: [w95] -> _
          shift-left: FALSE -> [w96]
          shift-right: [w93] -> _
          shift-left: 0.0 -> [w94]
          stop <- w130 stop-if-true
          # "Laser 2"
          # "Laser 1"
          # "Handles manual triggering\nof audio and lasers"
          n31 = node-c288() -> (w128:i64)  [unwired: 1 in]
          n32 = xnode "Read/Write Control"("FPGA VI Reference In"=w126, "error in"=w127) -> ("FPGA VI Reference Out"=w98:refnum<k20>, "error out"=w97:errorcluster, "A2_LickL"=w105:u32, "A4_LickR"=w103:u32)
          n33 = local write "A2"(w105) -> ()
          n34 = local write "A4"(w103) -> ()
          n35 = case shown="\"UploadSettings_dataExp_1\"" w123 {
            selector: w123 -> [_ w155 _ _ _ _ _ _ _ _ _ _ _ _ _ _ _ _ _ w1059 w1118 _ _ w1323 _ _ _ w1396 w1437]
            tunnel: [myRIO_BRig_RT__Case_NonExp_stateList."Idle" ("Enum") w153 w160 w179 w198 myRIO_BRig_RT__Case_NonExp_stateList."UploadSettings_dataExp_2" ("Enum") myRIO_BRig_RT__Case_NonExp_stateList."UploadSettings_Read_dataLC" ("Enum") myRIO_BRig_RT__Case_NonExp_stateList."UploadSettings_dataLC_2" ("Enum") myRIO_BRig_RT__Case_NonExp_stateList."UploadSettings_dataLC_4" ("Enum") myRIO_BRig_RT__Case_NonExp_stateList."UploadSettings_dataLC_3" ("f") myRIO_BRig_RT__Case_NonExp_stateList."UploadSettings_Read_dataMTrig" ("f") myRIO_BRig_RT__Case_NonExp_stateList."Idle" ("Enum") w606 w642 myRIO_BRig_RT__Case_NonExp_stateList."Idle_5" ("Enum") w715 w833 w995 w1026 w1054 w1113 myRIO_BRig_RT__Case_NonExp_stateList."DispenseWater_pre" ("Enum") w1269 w1321 w1343 myRIO_BRig_RT__Case_NonExp_stateList."Idle" ("Enum") myRIO_BRig_RT__Case_NonExp_stateList."Idle" ("Enum") w1395 w1437] -> w112
            tunnel: [w143 w152 w170 w189 w208 w272 w356 w409 w468 w521 w568 w584 w610 w657 w701 w720 w838 w993 w1033 w1060 w1119 w1180 w1306 w1328 w1354 w1388 w1393 w1405 w1435] -> w118
            tunnel: [_ _ _ _ _ _ _ _ _ _ _ _ _ _ _ _ _ _ _ _ _ _ _ _ _ _ _ _ TRUE] -> w130
            tunnel: w129 -> [_ w152 w170 w189 w208 w272 w356 w409 w468 w521 w568 w585 w609 w657 w701 w721 w839 w993 w1034 w1061 w1120 w1166 w1302 w1329 w1355 w1388 w1393 w1405 w1435]
            tunnel: w128 -> [_ _ _ _ _ _ _ _ _ _ _ _ _ _ _ _ _ _ _ _ _ _ _ w1333 _ _ _ _ _]
            tunnel: [_ _ w161 w180 w199 w237 w354 w410 w469 w517 w564 w569 _ _ _ _ _ _ w1022 _ w1107 _ _ _ _ _ _ _ _] -> w122
            tunnel: w121 -> [_ _ w162 w181 w200 w237 w354 w410 w469 w517 w564 w569 _ _ _ _ _ _ _ _ w1108 _ _ _ _ _ _ _ _]
            tunnel: [_ _ _ _ _ _ _ _ _ _ _ _ _ _ _ _ _ _ _ _ _ _ _ w1330 _ _ _ _ _] -> w120
            tunnel: [_ _ _ _ _ _ _ _ _ _ _ _ _ _ _ _ _ _ _ _ _ _ _ w1312 _ _ _ _ _] -> w119
            tunnel: w108 -> [_ w159 _ _ _ _ _ _ _ _ _ _ _ _ _ _ _ _ _ _ _ _ _ _ _ _ _ _ _]
            tunnel: [_ w158 _ _ _ _ _ _ _ _ _ _ _ _ _ _ _ _ _ _ _ _ _ _ _ _ _ _ _] -> w107
            tunnel: w106 -> [_ _ _ _ _ _ _ _ _ _ _ _ _ _ _ _ _ _ _ w1065 w1124 _ _ _ _ _ _ _ _]
            tunnel: w105 -> [_ _ _ _ _ _ _ _ _ _ _ _ _ _ _ _ _ _ _ w1066 w1125 _ _ _ _ _ _ _ _]
            tunnel: w104 -> [_ _ _ _ _ _ _ _ _ _ _ _ _ _ _ _ _ _ _ w1063 w1122 _ _ _ _ _ _ _ _]
            tunnel: w103 -> [_ _ _ _ _ _ _ _ _ _ _ _ _ _ _ _ _ _ _ w1064 w1123 _ _ _ _ _ _ _ _]
            tunnel: w102 -> [_ _ _ _ _ _ _ _ _ _ _ _ _ _ _ _ _ _ _ w1051 w1110 _ _ _ _ _ _ _ _]
            tunnel: w101 -> [_ _ _ _ _ _ _ _ _ _ _ _ _ _ _ _ _ _ _ w1050 w1109 _ _ _ _ _ _ _ _]
            tunnel: [_ _ _ _ _ _ _ _ _ _ _ _ _ _ _ _ _ _ w1024 w1051 w1110 _ _ _ _ _ _ _ _] -> w100
            tunnel: [_ _ _ _ _ _ _ _ _ _ _ _ _ _ _ _ _ _ w1023 w1050 w1109 _ _ _ _ _ _ _ _] -> w99
            tunnel: w98 -> [_ _ _ _ _ _ _ _ _ _ _ _ w599 w615 w703 _ _ _ _ _ w1106 _ _ _ _ _ _ w1400 _]
            tunnel: w97 -> [_ _ _ _ _ _ _ _ _ _ _ _ w598 w616 w702 _ _ _ _ _ w1105 _ _ _ _ _ _ w1399 _]
            tunnel: w96 -> [_ _ _ _ _ _ _ _ _ _ _ _ _ _ _ _ _ _ _ _ _ _ _ _ _ _ _ w1404 _]
            tunnel: [_ _ _ _ _ _ _ _ _ _ _ _ _ _ _ _ _ _ _ _ _ _ _ _ _ _ _ TRUE _] -> w95
            tunnel: w94 -> [_ _ _ _ _ _ _ _ _ _ _ _ _ _ _ _ _ _ _ _ _ _ _ _ _ _ _ w1402 _]
            tunnel: [_ _ _ _ _ _ _ _ _ _ _ _ _ _ _ _ _ _ _ _ _ _ _ _ _ _ _ w1401 _] -> w93
            frame "Init", Default {
              w134 = FALSE ("RewCalib_Trig_L")
              w135 = u16 100 ("new element/subarray")
              # "Only happens at start of NonExperiment Case"
              # "Tdelay_R"
              # "Tdelay_L"
              # "RewCalib_N__R"
              # "RewCalib_N__L"
              # "Solenoid_Tcycle_R"
              # "Solenoid_Tcycle_L"
              # "Laser_Tcycle"
              # "Audio_Tcycle_R"
              # "Audio_Tcycle_L"
              # "initialize dataMTrig"
              n36 = local write "RewCalib_Trig_L"(w134) -> ()
              n37 = local write "RewCalib_Trig_R"(w134) -> ()
              n38 = local write "MTrig_Audio_trig__L"(w134) -> ()
              n39 = local write "MTrig_Audio_trig__R"(w134) -> ()
              n40 = local write "MTrig_Laser_trig"(w134) -> ()
              n41 = local write "MTrig_Solenoid_trig__L"(w134) -> ()
              n42 = local write "MTrig_Solenoid_trig__R"(w134) -> ()
              n43 = local write "MTrig_CueLed"(w134) -> ()
              n44 = call "myRIO_BRig_RT_dataMTrig_Solenoid_Tcycle__L.vi"() -> ("output_Solenoid_Tcycle__L"=w145:i32)  [unwired: 11 in]
              n45 = call "myRIO_BRig_RT_dataMTrig_Solenoid_Tcycle__R.vi"() -> ("output_Solenoid_Tcycle__R"=w146:i32)  [unwired: 11 in]
              n46 = call "myRIO_BRig_RT_dataMTrig_Audio_Tcycle__L.vi"() -> ("output_Audio_Tcycle__L"=w147:i32)  [unwired: 11 in]
              n47 = call "myRIO_BRig_RT_dataMTrig_Audio_Tcycle__R.vi"() -> ("output_Audio_Tcycle__R"=w148:i32)  [unwired: 11 in]
              n48 = call "myRIO_BRig_RT_dataMTrig_Laser_Tcycle.vi"() -> ("output_Laser_Tcycle"=w149:i32)  [unwired: 11 in]
              n49 = call "myRIO_BRig_RT_dataMTrig_Solenoid_RewCalib_nCycle__L.vi"() -> ("output_Solenoid_RewCalib_nCycle__L"=w141:i32)  [unwired: 11 in]
              n50 = call "myRIO_BRig_RT_dataMTrig_Solenoid_RewCalib_nCycle__R.vi"() -> ("output_Solenoid_RewCalib_nCycle__R"=w140:i32)  [unwired: 11 in]
              n51 = call "myRIO_BRig_RT_dataMTrig_Solenoid_Tdelay__L.vi"() -> ("output_Solenoid_Tdelay__L"=w139:i32)  [unwired: 11 in]
              n52 = call "myRIO_BRig_RT_dataMTrig_Solenoid_Tdelay__R.vi"() -> ("output_Solenoid_Tdelay__R"=w138:i32)  [unwired: 11 in]
              n53 = call "myRIO_BRig_RT_dataMTrig_CueLed_Tcycle.vi"() -> ("output_CueLed_Tcycle"=w133:i32)  [unwired: 11 in]
              n54 = local read "MTrig_Solenoid_Tcycle__L"() -> (w150:u16)
              n55 = local read "MTrig_Solenoid_Tcycle__R"() -> (w151:u16)
              n56 = local read "MTrig_Laser_Tcycle"() -> (w136:u16)
              n57 = call "myRIO_BRig_RT_dataMTrig_init.vi"() -> ("output_dataMTrig"=w144:u16[])  [unwired: 5 in]
              n58 = local read "Tcycle_Cue_LED_min"() -> (w132:u16)
              n59 = local read "Tcycle_Cue_Audio_min"() -> (w137:u16)
              n60 = Replace Array Subset(array=w144, new element #1=w150, index #1=w145, new element #2=w151, index #2=w146, new element #3=w137, index #3=w147, new element #4=w137, index #4=w148, new element #5=w136, index #5=w149, new element #6=w135, index #6=w141, new element #7=w135, index #7=w140, new element #8=w135, index #8=w139, new element #9=w135, index #9=w138, new element #10=w132, index #10=w133) -> (w143:u16[])
            }
            frame "UploadSettings_pre" {
              # "When the Host sends settings,\nnot all files send at the same time.\n\nIf RT reads the settings faster\nthan the Host can send them,\nthen we will skip settings.\n\nSolution:\nWait 20 cycles"
              n61 = Increment(x=w159) -> (x+1=w158:u16)
              n62 = Greater?(x=w158, y=u16 20) -> (0:w156:bool)
              n63 = Select(t=myRIO_BRig_RT__Case_NonExp_stateList."UploadSettings_Read_dataExp", s=w156, f=w155) -> (s? t:f=w153:T1)
            }
            frame "UploadSettings_Read_dataExp" {
              # "Grab data but do not act on it yet"
              # "grab dataExp and\nstore it in the\ngeneric data array"
              # "dataExp"
              n64 = call "myRIO_BRig_RT_dataExp_init_details.vi"() -> ("output_dataSize"=w166:i32, "output_dataName"=w169:string)  [unwired: 10 in]
              n65 = call "myRIO_BRig_RT_comm_webdav_uploadReceived_check.vi"("input_dataName"=w169) -> ("output_Iexist"=w168:bool, "output_dataPath"=w167:path)  [unwired: 9 in]
              n66 = case shown="True" w168 {
                tunnel: w167 -> [_ w178]
                tunnel: w166 -> [_ w177]
                tunnel: [_ w176] -> w165
                tunnel: w162 -> [w171 w175]
                tunnel: [w171 w172] -> w161
                frame False {
                }
                frame True {
                  n67 = call "myRIO_BRig_RT_comm_webdav_uploadReceived_read.vi"("input_dataSize"=w177, "input_filePath"=w178) -> ("output_Ivalid"=w176:bool, "output_data"=w174:i64[])  [unwired: 8 in]
                  n68 = To Unsigned Word Integer(number=w174) -> (unsigned 16bit integer=w173:u16[])
                  n69 = Select(t=w173, s=w176, f=w175) -> (s? t:f=w172:u16[])
                }
              }
              n70 = Select(t=myRIO_BRig_RT__Case_NonExp_stateList."UploadSettings_dataExp_1", s=w165, f=myRIO_BRig_RT__Case_NonExp_stateList."UploadSettings_Read_dataLC" ("t")) -> (s? t:f=w160:T1)
            }
            frame "UploadSettings_Read_dataLC" {
              # "Grab data but do not act on it yet"
              # "grab dataLC and\nstore it in the\ngeneric data array"
              # "dataLC"
              n71 = call "myRIO_BRig_RT_dataLC_init_details.vi"() -> ("output_dataSize"=w185:i32, "output_dataName"=w188:string)  [unwired: 10 in]
              n72 = call "myRIO_BRig_RT_comm_webdav_uploadReceived_check.vi"("input_dataName"=w188) -> ("output_Iexist"=w187:bool, "output_dataPath"=w186:path)  [unwired: 9 in]
              n73 = case shown="True" w187 {
                tunnel: w186 -> [_ w197]
                tunnel: w185 -> [_ w196]
                tunnel: [_ w195] -> w184
                tunnel: w181 -> [w190 w194]
                tunnel: [w190 w191] -> w180
                frame False {
                }
                frame True {
                  n74 = call "myRIO_BRig_RT_comm_webdav_uploadReceived_read.vi"("input_dataSize"=w196, "input_filePath"=w197) -> ("output_Ivalid"=w195:bool, "output_data"=w193:i64[])  [unwired: 8 in]
                  n75 = To Unsigned Word Integer(number=w193) -> (unsigned 16bit integer=w192:u16[])
                  n76 = Select(t=w192, s=w195, f=w194) -> (s? t:f=w191:u16[])
                }
              }
              n77 = Select(t=myRIO_BRig_RT__Case_NonExp_stateList."UploadSettings_dataLC_1", s=w184, f=myRIO_BRig_RT__Case_NonExp_stateList."UploadSettings_Read_dataMTrig" ("t")) -> (s? t:f=w179:T1)
            }
            frame "UploadSettings_Read_dataMTrig" {
              # "Grab data but do not act on it yet"
              # "grab dataMTrig and\nstore it in the\ngeneric data array"
              # "dataMTrig"
              n78 = call "myRIO_BRig_RT_dataMTrig_init_details.vi"() -> ("output_dataSize"=w204:i32, "output_dataName"=w207:string)  [unwired: 10 in]
              n79 = call "myRIO_BRig_RT_comm_webdav_uploadReceived_check.vi"("input_dataName"=w207) -> ("output_Iexist"=w206:bool, "output_dataPath"=w205:path)  [unwired: 9 in]
              n80 = case shown="True" w206 {
                tunnel: w205 -> [_ w216]
                tunnel: w204 -> [_ w215]
                tunnel: [_ w214] -> w203
                tunnel: w200 -> [w209 w213]
                tunnel: [w209 w210] -> w199
                frame False {
                }
                frame True {
                  n81 = call "myRIO_BRig_RT_comm_webdav_uploadReceived_read.vi"("input_dataSize"=w215, "input_filePath"=w216) -> ("output_Ivalid"=w214:bool, "output_data"=w212:i64[])  [unwired: 8 in]
                  n82 = To Unsigned Word Integer(number=w212) -> (unsigned 16bit integer=w211:u16[])
                  n83 = Select(t=w211, s=w214, f=w213) -> (s? t:f=w210:u16[])
                }
              }
              n84 = Select(t=myRIO_BRig_RT__Case_NonExp_stateList."UploadSettings_dataMTrig_1", s=w203, f=myRIO_BRig_RT__Case_NonExp_stateList."Idle" ("t")) -> (s? t:f=w198:T1)
            }
            frame "UploadSettings_dataExp_1" {
              # "Cue_max"
              # "Cue_min"
              # "CuePenalty"
              # "Timeout"
              # "Wrong"
              # "Selection"
              # "RewardPost"
              # "Tcycle"
              # "TPB_min_R"
              # "TPB_min_L"
              # "TPB_max_R"
              # "TPB_max_L"
              # "I_trialUntilReward"
              # "ENL_penalty"
              # "ENL_min"
              # "ENL_max"
              # "BUR_max"
              # "BUR_min"
              # "CueCycles"
              # "Audio_Freq_R"
              # "Audio_Freq_L"
              # "Audio_Amp_R"
              # "Audio_Amp_L"
              n85 = call "myRIO_BRig_RT_dataExp_CueCycles.vi"() -> ("output_CueCycles"=w264:i32)  [unwired: 11 in]
              n86 = call "myRIO_BRig_RT_dataExp_Audio_amp__R.vi"() -> ("output_Audio_amp__R"=w268:i32)  [unwired: 11 in]
              n87 = call "myRIO_BRig_RT_dataExp_Audio_amp__L.vi"() -> ("output_Audio_amp__L"=w270:i32)  [unwired: 11 in]
              n88 = call "myRIO_BRig_RT_dataExp_Tcycle_RewardPost.vi"() -> ("output_Tcycle_RewardPost"=w236:i32)  [unwired: 11 in]
              n89 = call "myRIO_BRig_RT_dataExp_BUR_min.vi"() -> ("output_BUR_min"=w261:i32)  [unwired: 11 in]
              n90 = call "myRIO_BRig_RT_dataExp_ENL_min.vi"() -> ("output_ENL_min"=w257:i32)  [unwired: 11 in]
              n91 = call "myRIO_BRig_RT_dataExp_TPB_max__L.vi"() -> ("output_TPB_max__L"=w249:i32)  [unwired: 11 in]
              n92 = call "myRIO_BRig_RT_dataExp_TPB_max__R.vi"() -> ("output_TPB_max__R"=w248:i32)  [unwired: 11 in]
              n93 = call "myRIO_BRig_RT_dataExp_ENL_penalty.vi"() -> ("output_ENL_penalty"=w256:i32)  [unwired: 11 in]
              n94 = call "myRIO_BRig_RT_dataExp_Audio_freq__L.vi"() -> ("output_Audio_freq__L"=w266:i32)  [unwired: 11 in]
              n95 = call "myRIO_BRig_RT_dataExp_Audio_freq__R.vi"() -> ("output_Audio_freq__R"=w265:i32)  [unwired: 11 in]
              n96 = call "myRIO_BRig_RT_dataExp_BUR_max.vi"() -> ("output_BUR_max"=w262:i32)  [unwired: 11 in]
              n97 = call "myRIO_BRig_RT_dataExp_ENL_max.vi"() -> ("output_ENL_max"=w258:i32)  [unwired: 11 in]
              n98 = call "myRIO_BRig_RT_dataExp_ItrialUntilReward.vi"() -> ("output_I_trialUntilReward"=w252:i32)  [unwired: 11 in]
              n99 = call "myRIO_BRig_RT_dataExp_Tcycle_Selection.vi"() -> ("output_Tcycle_Selection"=w235:i32)  [unwired: 11 in]
              n100 = call "myRIO_BRig_RT_dataExp_Tcycle_Wrong.vi"() -> ("output_Tcycle_Wrong"=w234:i32)  [unwired: 11 in]
              n101 = call "myRIO_BRig_RT_dataExp_Tcycle_Timeout.vi"() -> ("output_Tcycle_Timeout"=w230:i32)  [unwired: 11 in]
              n102 = call "myRIO_BRig_RT_dataExp_TPB_min__L.vi"() -> ("output_TPB_min__L"=w247:i32)  [unwired: 11 in]
              n103 = call "myRIO_BRig_RT_dataExp_TPB_min__R.vi"() -> ("output_TPB_min__R"=w246:i32)  [unwired: 11 in]
              n104 = call "myRIO_BRig_RT_dataExp_Tcycle_Cue1Penalty_Audio.vi"() -> ("output_Tcycle_Cue1Penalty_Audio"=w228:i32)  [unwired: 11 in]
              n105 = call "myRIO_BRig_RT_dataExp_Tcycle_Cue1_Audio_min.vi"() -> ("output_Tcycle_Cue1_Audio_min"=w226:i32)  [unwired: 11 in]
              n106 = call "myRIO_BRig_RT_dataExp_Tcycle_Cue1_Audio_max.vi"() -> ("output_Tcycle_Cue1_Audio_max"=w224:i32)  [unwired: 11 in]
              n107 = call "myRIO_BRig_RT_dataExp_Tcycle_Cue1Penalty_LED.vi"() -> ("output_Tcycle_Cue1Penalty_LED"=w222:i32)  [unwired: 11 in]
              n108 = call "myRIO_BRig_RT_dataExp_Tcycle_Cue1_LED_min.vi"() -> ("output_Tcycle_Cue1_LED_min"=w221:i32)  [unwired: 11 in]
              n109 = call "myRIO_BRig_RT_dataExp_Tcycle_Cue1_LED_max.vi"() -> ("output_Tcycle_Cue1_LED_max"=w220:i32)  [unwired: 11 in]
              n110 = Index Array(array=w237, index #1=w270, index #2=w268, index #3=w266, index #4=w265, index #5=w264, index #6=w262, index #7=w261, index #8=w258, index #9=w257, index #10=w256, index #11=w252, index #12=w249, index #13=w248, index #14=w247, index #15=w246, index #16=w236, index #17=w235, index #18=w234, index #19=w230, index #20=w228, index #21=w226, index #22=w224, index #23=w222, index #24=w221, index #25=w220) -> (element #1=w269:u16, element #2=w267:u16, element #3=w240:u16, element #4=w239:u16, element #5=w263:u16, element #6=w260:u16, element #7=w259:u16, element #8=w255:u16, element #9=w254:u16, element #10=w253:u16, element #11=w250:u16, element #12=w245:u16, element #13=w244:u16, element #14=w243:u16, element #15=w242:u16, element #16=w233:u16, element #17=w232:u16, element #18=w231:u16, element #19=w229:u16, element #20=w227:u16, element #21=w225:u16, element #22=w223:u16, element #23=w219:u16, element #24=w218:u16, element #25=w217:u16)
              n111 = local write "Tcycle_CuePenalty_LED"(w219) -> ()
              n112 = local write "Tcycle_Cue_LED_min"(w218) -> ()
              n113 = local write "Tcycle_Cue_LED_max"(w217) -> ()
              n114 = local write "Tcycle_Selection"(w232) -> ()
              n115 = local write "Tcycle_Wrong"(w231) -> ()
              n116 = local write "Tcycle_Timeout"(w229) -> ()
              n117 = local write "Audio_Amp__L"(w269) -> ()
              n118 = local write "Audio_Amp__R"(w267) -> ()
              n119 = local write "Tcycle_ENLPenalty"(w253) -> ()
              n120 = local write "Tcycle_ENL_max"(w255) -> ()
              n121 = local write "TpB_Min_L"(w243) -> ()
              n122 = local write "TpB_Min_R"(w242) -> ()
              n123 = local write "Tcycle_CuePenalty_Audio"(w227) -> ()
              n124 = local write "Tcycle_Cue_Audio_min"(w225) -> ()
              n125 = local write "Tcycle_Cue_Audio_max"(w223) -> ()
              n126 = To Unsigned Byte Integer(number=w240) -> (unsigned 8bit integer=w241:u8)
              n127 = To Unsigned Byte Integer(number=w239) -> (unsigned 8bit integer=w238:u8)
              n128 = Not Equal To 0?(x=w250) -> (x != 0?=w251:bool)
              n129 = local write "Tcycle_RewardPost"(w233) -> ()
              n130 = local write "CueCycles"(w263) -> ()
              n131 = local write "BUR_min"(w259) -> ()
              n132 = local write "BUR_max"(w260) -> ()
              n133 = local write "Tcycle_ENL_min"(w254) -> ()
              n134 = local write "TpB_Max_L"(w245) -> ()
              n135 = local write "TpB_Max_R"(w244) -> ()
              n136 = local write "TrialUntilReward"(w251) -> ()
              n137 = local write "Audio_Freq__L"(w241) -> ()
              n138 = local write "Audio_Freq__R"(w238) -> ()
            }
            frame "UploadSettings_dataExp_2" {
              w292 = 100.0 ("y")
              n139 = call "myRIO_BRig_RT_dataExp_FPGA_f_count2ms.vi"() -> ("output_FPGA_f_count2ms"=w353:i32)  [unwired: 11 in]
              n140 = call "myRIO_BRig_RT_dataExp_laser1_Freq.vi"() -> ("output_laser1_Freq"=w341:i32)  [unwired: 11 in]
              n141 = call "myRIO_BRig_RT_dataExp_laser1_duration.vi"() -> ("output_laser1_duration"=w340:i32)  [unwired: 11 in]
              n142 = call "myRIO_BRig_RT_dataExp_laser1_Tpeak.vi"() -> ("output_laser1_Tpeak"=w339:i32)  [unwired: 11 in]
              n143 = call "myRIO_BRig_RT_dataExp_laser1_Tshutter.vi"() -> ("output_laser1_Tshutter"=w338:i32)  [unwired: 11 in]
              n144 = call "myRIO_BRig_RT_dataExp_laser1_Power_min.vi"() -> ("output_laser1_Power_min"=w337:i32)  [unwired: 11 in]
              n145 = call "myRIO_BRig_RT_dataExp_laser1_Power_max.vi"() -> ("output_laser1_Power_max"=w336:i32)  [unwired: 11 in]
              n146 = call "myRIO_BRig_RT_dataExp_laser1_Power_step.vi"() -> ("output_laser1_Power_step"=w335:i32)  [unwired: 11 in]
              n147 = call "myRIO_BRig_RT_dataExp_Cue1Param_CueType_Switch.vi"() -> ("output_Cue1Param_CueType_Switch"=w286:i32)  [unwired: 11 in]
              n148 = call "myRIO_BRig_RT_dataExp_Cue1Param_AudioLed_Count_Switch.vi"() -> ("output_Cue1Param_AudioLed_Count_Switch"=w285:i32)  [unwired: 11 in]
              n149 = call "myRIO_BRig_RT_dataExp_Cue1Param_AudioLed_Probability_Switch.vi"() -> ("output_Cue1Param_AudioLed_Probability_Switch"=w284:i32)  [unwired: 11 in]
              n150 = call "myRIO_BRig_RT_dataExp_SolenoidProbability_L.vi"() -> ("output_SolenoidProbability_L"=w288:i32)  [unwired: 11 in]
              n151 = call "myRIO_BRig_RT_dataExp_SolenoidProbability_R.vi"() -> ("output_SolenoidProbability_R"=w287:i32)  [unwired: 11 in]
              n152 = call "myRIO_BRig_RT_dataExp_Cue1Param_CueType_NS.vi"() -> ("output_Cue1Param_CueType_NS"=w283:i32)  [unwired: 11 in]
              n153 = call "myRIO_BRig_RT_dataExp_Cue1Param_AudioLed_Count_NS.vi"() -> ("output_Cue1Param_AudioLed_Count_NS"=w282:i32)  [unwired: 11 in]
              n154 = call "myRIO_BRig_RT_dataExp_Cue1Param_AudioLed_Probability_NS.vi"() -> ("output_Cue1Param_AudioLed_Probability_NS"=w281:i32)  [unwired: 11 in]
              n155 = call "myRIO_BRig_RT_dataExp_laser2_Freq.vi"() -> ("output_laser2_Freq"=w334:i32)  [unwired: 11 in]
              n156 = call "myRIO_BRig_RT_dataExp_laser2_duration.vi"() -> ("output_laser2_duration"=w333:i32)  [unwired: 11 in]
              n157 = call "myRIO_BRig_RT_dataExp_laser2_Tpeak.vi"() -> ("output_laser2_Tpeak"=w332:i32)  [unwired: 11 in]
              n158 = call "myRIO_BRig_RT_dataExp_laser2_Tshutter.vi"() -> ("output_laser2_Tshutter"=w331:i32)  [unwired: 11 in]
              n159 = call "myRIO_BRig_RT_dataExp_laser2_Power_min.vi"() -> ("output_laser2_Power_min"=w330:i32)  [unwired: 11 in]
              n160 = call "myRIO_BRig_RT_dataExp_laser2_Power_max.vi"() -> ("output_laser2_Power_max"=w329:i32)  [unwired: 11 in]
              n161 = call "myRIO_BRig_RT_dataExp_laser2_Power_step.vi"() -> ("output_laser2_Power_step"=w328:i32)  [unwired: 11 in]
              n162 = call "myRIO_BRig_RT_dataExp_CueLed_Freq.vi"() -> ("output_CueLed_Freq"=w297:i32)  [unwired: 11 in]
              n163 = call "myRIO_BRig_RT_dataExp_CueLed_Tpeak.vi"() -> ("output_CueLed_Tpeak"=w290:i32)  [unwired: 11 in]
              n164 = Index Array(array=w354, index #1=w353, index #2=w341, index #3=w340, index #4=w339, index #5=w338, index #6=w337, index #7=w336, index #8=w335, index #9=w334, index #10=w333, index #11=w332, index #12=w331, index #13=w330, index #14=w329, index #15=w328, index #16=w297, index #17=w290, index #18=w288, index #19=w287, index #20=w286, index #21=w285, index #22=w284, index #23=w283, index #24=w282, index #25=w281) -> (element #1=w352:u16, element #2=w327:u16, element #3=w326:u16, element #4=w325:u16, element #5=w324:u16, element #6=w323:u16, element #7=w313:u16, element #8=w312:u16, element #9=w308:u16, element #10=w307:u16, element #11=w306:u16, element #12=w305:u16, element #13=w304:u16, element #14=w299:u16, element #15=w298:u16, element #16=w291:u16, element #17=w289:u16, element #18=w280:u16, element #19=w279:u16, element #20=w278:u16, element #21=w277:u16, element #22=w276:u16, element #23=w275:u16, element #24=w274:u16, element #25=w273:u16)
              n165 = local write "Cue1Param_CueType_Switch"(w278) -> ()
              n166 = local write "Cue1Param_AudioLed_Count_Switch"(w277) -> ()
              n167 = local write "Cue1Param_AudioLed_Probability_Switch"(w276) -> ()
              n168 = local write "Cue1Param_CueType_NS"(w275) -> ()
              n169 = local write "Cue1Param_AudioLed_Count_NS"(w274) -> ()
              n170 = local write "Cue1Param_AudioLed_Probability_NS"(w273) -> ()
              n171 = To Double Precision Float(number=w352) -> (double precision float=w351:dbl)
              n172 = To Double Precision Float(number=w327) -> (double precision float=w349:dbl)
              n173 = To Double Precision Float(number=w325) -> (double precision float=w346:dbl)
              n174 = To Double Precision Float(number=w324) -> (double precision float=w345:dbl)
              n175 = To Double Precision Float(number=w323) -> (double precision float=w347:dbl)
              n176 = To Double Precision Float(number=w313) -> (double precision float=w318:dbl)
              n177 = To Double Precision Float(number=w312) -> (double precision float=w314:dbl)
              n178 = To Double Precision Float(number=w308) -> (double precision float=w319:dbl)
              n179 = To Double Precision Float(number=w306) -> (double precision float=w321:dbl)
              n180 = To Double Precision Float(number=w305) -> (double precision float=w322:dbl)
              n181 = To Double Precision Float(number=w304) -> (double precision float=w320:dbl)
              n182 = To Double Precision Float(number=w299) -> (double precision float=w302:dbl)
              n183 = To Double Precision Float(number=w298) -> (double precision float=w303:dbl)
              n184 = To Double Precision Float(number=w291) -> (double precision float=w296:dbl)
              n185 = To Double Precision Float(number=w289) -> (double precision float=w295:dbl)
              n186 = local write "SolenoidProbability_L"(w280) -> ()
              n187 = local write "SolenoidProbability_R"(w279) -> ()
              n188 = Divide(x=w351, y=w292) -> (x/y=w350:dbl)
              n189 = Divide(x=w349, y=w292) -> (x/y=w348:dbl)
              n190 = Divide(x=w346, y=w292) -> (x/y=w343:dbl)
              n191 = Divide(x=w345, y=w292) -> (x/y=w342:dbl)
              n192 = Divide(x=w347, y=w292) -> (x/y=w344:dbl)
              n193 = Divide(x=w318, y=w292) -> (x/y=w316:dbl)
              n194 = Divide(x=w314, y=w292) -> (x/y=w315:dbl)
              n195 = Divide(x=w319, y=w292) -> (x/y=w317:dbl)
              n196 = Divide(x=w321, y=w292) -> (x/y=w311:dbl)
              n197 = Divide(x=w322, y=w292) -> (x/y=w310:dbl)
              n198 = Divide(x=w320, y=w292) -> (x/y=w309:dbl)
              n199 = Divide(x=w302, y=w292) -> (x/y=w301:dbl)
              n200 = Divide(x=w303, y=w292) -> (x/y=w300:dbl)
              n201 = Divide(x=w296, y=w292) -> (x/y=w294:dbl)
              n202 = Divide(x=w295, y=w292) -> (x/y=w293:dbl)
              n203 = local write "FPGA_count2ms"(w350) -> ()
              n204 = local write "Laser_Freq_l1"(w348) -> ()
              n205 = local write "Laser_duration_l1"(w326) -> ()
              n206 = local write "Laser_Tpeak_l1"(w343) -> ()
              n207 = local write "Laser_Tshutter_l1"(w342) -> ()
              n208 = local write "Laser_power_min_l1"(w344) -> ()
              n209 = local write "Laser_power_max_l1"(w316) -> ()
              n210 = local write "Laser_power_step_l1"(w315) -> ()
              n211 = local write "Laser_Freq_l2"(w317) -> ()
              n212 = local write "Laser_duration_l2"(w307) -> ()
              n213 = local write "Laser_Tpeak_l2"(w311) -> ()
              n214 = local write "Laser_Tshutter_l2"(w310) -> ()
              n215 = local write "Laser_power_min_l2"(w309) -> ()
              n216 = local write "Laser_power_max_l2"(w301) -> ()
              n217 = local write "Laser_power_step_l2"(w300) -> ()
              n218 = local write "CueLed_Freq"(w294) -> ()
              n219 = local write "CueLed_Tpeak"(w293) -> ()
            }
            frame "UploadSettings_dataLC_1" {
              # "Cue1_delayOpt_NonSwitch"
              # "ENL1_delayOpt_NonSwitch"
              # "Cue1_delayOpt_Switch"
              # "ENL1_delayOpt_Switch"
              # "Count"
              # "Tdelay"
              # "Prob"
              # "OnOff"
              # "Block"
              # "Count"
              # "Tdelay"
              # "Prob"
              # "OnOff"
              # "Block"
              # "Count"
              # "Tdelay"
              # "Prob"
              # "OnOff"
              # "Block"
              # "ENL1 Switch"
              # "Cue1 NonSwitch"
              # "Cue1 Switch"
              # "ENL1 NonSwitch"
              # "Count"
              # "Tdelay"
              # "Prob"
              # "OnOff"
              # "Block"
              n220 = call "myRIO_BRig_RT_dataLC_ENL1_OnOff_Switch_l1.vi"() -> ("output_ENL1_OnOff_Switch_l1"=w408:i32)  [unwired: 11 in]
              n221 = call "myRIO_BRig_RT_dataLC_ENL1_Tdelay_Switch_l1.vi"() -> ("output_ENL1_Tdelay_Switch_l1"=w407:i32)  [unwired: 11 in]
              n222 = call "myRIO_BRig_RT_dataLC_ENL1_Block_Switch_l1.vi"() -> ("output_ENL1_Block_Switch_l1"=w406:i32)  [unwired: 11 in]
              n223 = call "myRIO_BRig_RT_dataLC_ENL1_Count_Switch_l1.vi"() -> ("output_ENL1_Count_Switch_l1"=w405:i32)  [unwired: 11 in]
              n224 = call "myRIO_BRig_RT_dataLC_ENL1_Probability_Switch_l1.vi"() -> ("output_ENL1_Probability_Switch_l1"=w404:i32)  [unwired: 11 in]
              n225 = call "myRIO_BRig_RT_dataLC_ENL1_OnOff_NS_l1.vi"() -> ("output_ENL1_OnOff_NS_l1"=w403:i32)  [unwired: 11 in]
              n226 = call "myRIO_BRig_RT_dataLC_ENL1_Tdelay_NS_l1.vi"() -> ("output_ENL1_Tdelay_NS_l1"=w402:i32)  [unwired: 11 in]
              n227 = call "myRIO_BRig_RT_dataLC_ENL1_Block_NS_l1.vi"() -> ("output_ENL1_All_Block"=w401:i32)  [unwired: 11 in]
              n228 = call "myRIO_BRig_RT_dataLC_ENL1_Count_NS_l1.vi"() -> ("output_ENL1_Count_NS_l1"=w400:i32)  [unwired: 11 in]
              n229 = call "myRIO_BRig_RT_dataLC_ENL1_Probability_NS_l1.vi"() -> ("output_ENL1_Probability_NS_l1"=w399:i32)  [unwired: 11 in]
              n230 = call "myRIO_BRig_RT_dataLC_Cue1_OnOff_Switch_l1.vi"() -> ("output_Cue1_OnOff_Switch_l1"=w398:i32)  [unwired: 11 in]
              n231 = call "myRIO_BRig_RT_dataLC_Cue1_Tdelay_Switch_l1.vi"() -> ("output_Cue1_Tdelay_Switch_l1"=w397:i32)  [unwired: 11 in]
              n232 = call "myRIO_BRig_RT_dataLC_Cue1_Block_Switch_l1.vi"() -> ("output_Cue1_Block_Switch_l1"=w396:i32)  [unwired: 11 in]
              n233 = call "myRIO_BRig_RT_dataLC_Cue1_Count_Switch_l1.vi"() -> ("output_Cue1_Count_Switch_l1"=w395:i32)  [unwired: 11 in]
              n234 = call "myRIO_BRig_RT_dataLC_Cue1_Probability_Switch_l1.vi"() -> ("output_Cue1_Probability_Switch_l1"=w394:i32)  [unwired: 11 in]
              n235 = call "myRIO_BRig_RT_dataLC_Cue1_OnOff_NS_l1.vi"() -> ("output_Cue1_OnOff_NS_l1"=w393:i32)  [unwired: 11 in]
              n236 = call "myRIO_BRig_RT_dataLC_Cue1_Tdelay_NS_l1.vi"() -> ("output_Cue1_Tdelay_NS_l1"=w392:i32)  [unwired: 11 in]
              n237 = call "myRIO_BRig_RT_dataLC_Cue1_Block_NS_l1.vi"() -> ("output_Cue1_Block_NS_l1"=w391:i32)  [unwired: 11 in]
              n238 = call "myRIO_BRig_RT_dataLC_Cue1_Count_NS_l1.vi"() -> ("output_Cue1_Count_NS_l1"=w390:i32)  [unwired: 11 in]
              n239 = call "myRIO_BRig_RT_dataLC_Cue1_Probability_NS_l1.vi"() -> ("output_Cue1_l1_All_Probability"=w389:i32)  [unwired: 11 in]
              n240 = call "myRIO_BRig_RT_dataLC_ENL1_delayOpt_Switch_l1.vi"() -> ("output_ENL1_delayOpt_Switch_l1"=w368:i32)  [unwired: 11 in]
              n241 = call "myRIO_BRig_RT_dataLC_ENL1_delayOpt_NS_l1.vi"() -> ("output_ENL1_delayOpt_NS_l1"=w367:i32)  [unwired: 11 in]
              n242 = call "myRIO_BRig_RT_dataLC_Cue1_delayOpt_Switch_l1.vi"() -> ("output_Cue1_delayOpt_Switch_l1"=w366:i32)  [unwired: 11 in]
              n243 = call "myRIO_BRig_RT_dataLC_Cue1_delayOpt_NS_l1.vi"() -> ("output_Cue1_delayOpt_NS_l1"=w365:i32)  [unwired: 11 in]
              n244 = Index Array(array=w410, index #1=w408, index #2=w407, index #3=w406, index #4=w405, index #5=w404, index #6=w403, index #7=w402, index #8=w401, index #9=w400, index #10=w399, index #11=w398, index #12=w397, index #13=w396, index #14=w395, index #15=w394, index #16=w393, index #17=w392, index #18=w391, index #19=w390, index #20=w389, index #21=w368, index #22=w367, index #23=w366, index #24=w365) -> (element #1=w388:u16, element #2=w387:u16, element #3=w386:u16, element #4=w385:u16, element #5=w384:u16, element #6=w383:u16, element #7=w382:u16, element #8=w381:u16, element #9=w380:u16, element #10=w379:u16, element #11=w378:u16, element #12=w377:u16, element #13=w376:u16, element #14=w375:u16, element #15=w374:u16, element #16=w373:u16, element #17=w372:u16, element #18=w371:u16, element #19=w370:u16, element #20=w369:u16, element #21=w360:u16, element #22=w359:u16, element #23=w358:u16, element #24=w357:u16)
              n245 = Not Equal To 0?(x=w388) -> (x != 0?=w412:bool)
              n246 = Not Equal To 0?(x=w383) -> (x != 0?=w411:bool)
              n247 = Not Equal To 0?(x=w378) -> (x != 0?=w414:bool)
              n248 = Not Equal To 0?(x=w373) -> (x != 0?=w413:bool)
              n249 = Not Equal To 0?(x=w360) -> (x != 0?=w362:bool)
              n250 = Not Equal To 0?(x=w359) -> (x != 0?=w363:bool)
              n251 = Not Equal To 0?(x=w358) -> (x != 0?=w364:bool)
              n252 = Not Equal To 0?(x=w357) -> (x != 0?=w361:bool)
              n253 = local write "LC_ENL1_OnOff_Switch_l1"(w412) -> ()
              n254 = local write "LC_ENL1_Tdelay_Switch_l1"(w387) -> ()
              n255 = local write "LC_ENL1_Block_Switch_l1"(w386) -> ()
              n256 = local write "LC_ENL1_Count_Switch_l1"(w385) -> ()
              n257 = local write "LC_ENL1_Probability_Switch_l1"(w384) -> ()
              n258 = local write "LC_ENL1_OnOff_NS_l1"(w411) -> ()
              n259 = local write "LC_ENL1_Tdelay_NS_l1"(w382) -> ()
              n260 = local write "LC_ENL1_Block_NS_l1"(w381) -> ()
              n261 = local write "LC_ENL1_Count_NS_l1"(w380) -> ()
              n262 = local write "LC_ENL1_Probability_NS_l1"(w379) -> ()
              n263 = local write "LC_Cue1_OnOff_Switch_l1"(w414) -> ()
              n264 = local write "LC_Cue1_Tdelay_Switch_l1"(w377) -> ()
              n265 = local write "LC_Cue1_Block_Switch_l1"(w376) -> ()
              n266 = local write "LC_Cue1_Count_Switch_l1"(w375) -> ()
              n267 = local write "LC_Cue1_Probability_Switch_l1"(w374) -> ()
              n268 = local write "LC_Cue1_OnOff_NS_l1"(w413) -> ()
              n269 = local write "LC_Cue1_Tdelay_NS_l1"(w372) -> ()
              n270 = local write "LC_Cue1_Block_NS_l1"(w371) -> ()
              n271 = local write "LC_Cue1_Count_NS_l1"(w370) -> ()
              n272 = local write "LC_Cue1_Probability_NS_l1"(w369) -> ()
              n273 = local write "LC_ENL1_delayOpt_Switch_l1"(w362) -> ()
              n274 = local write "LC_ENL1_delayOpt_NS_l1"(w363) -> ()
              n275 = local write "LC_Cue1_delayOpt_Switch_l1"(w364) -> ()
              n276 = local write "LC_Cue1_delayOpt_NS_l1"(w361) -> ()
            }
            frame "UploadSettings_dataLC_3" {
              # "Cue1_delayOpt_NonSwitch"
              # "ENL1_delayOpt_NonSwitch"
              # "Cue1_delayOpt_Switch"
              # "ENL1_delayOpt_Switch"
              # "Count"
              # "Tdelay"
              # "Prob"
              # "OnOff"
              # "Block"
              # "Count"
              # "Tdelay"
              # "Prob"
              # "OnOff"
              # "Block"
              # "Count"
              # "Tdelay"
              # "Prob"
              # "OnOff"
              # "Block"
              # "ENL1 Switch"
              # "Cue1 NonSwitch"
              # "Cue1 Switch"
              # "ENL1 NonSwitch"
              # "Count"
              # "Tdelay"
              # "Prob"
              # "OnOff"
              # "Block"
              n277 = call "myRIO_BRig_RT_dataLC_ENL1_OnOff_Switch_l2.vi"() -> ("output_ENL1_OnOff_Switch_l2"=w435:i32)  [unwired: 11 in]
              n278 = call "myRIO_BRig_RT_dataLC_ENL1_Tdelay_Switch_l2.vi"() -> ("output_ENL1_Tdelay_Switch_l2"=w436:i32)  [unwired: 11 in]
              n279 = call "myRIO_BRig_RT_dataLC_ENL1_Block_Switch_l2.vi"() -> ("output_ENL1_Block_Switch_l2"=w437:i32)  [unwired: 11 in]
              n280 = call "myRIO_BRig_RT_dataLC_ENL1_Count_Switch_l2.vi"() -> ("output_ENL1_Count_Switch_l2"=w438:i32)  [unwired: 11 in]
              n281 = call "myRIO_BRig_RT_dataLC_ENL1_Probability_Switch_l2.vi"() -> ("output_ENL1_Probability_Switch_l2"=w439:i32)  [unwired: 11 in]
              n282 = call "myRIO_BRig_RT_dataLC_ENL1_OnOff_NS_l2.vi"() -> ("output_ENL1_OnOff_NS_l2"=w430:i32)  [unwired: 11 in]
              n283 = call "myRIO_BRig_RT_dataLC_ENL1_Tdelay_NS_l2.vi"() -> ("output_ENL1_Tdelay_NS_l2"=w431:i32)  [unwired: 11 in]
              n284 = call "myRIO_BRig_RT_dataLC_ENL1_Block_NS_l2.vi"() -> ("output_ENL1_Block_NS_l2"=w432:i32)  [unwired: 11 in]
              n285 = call "myRIO_BRig_RT_dataLC_ENL1_Count_NS_l2.vi"() -> ("output_ENL1_Count_NS_l2"=w433:i32)  [unwired: 11 in]
              n286 = call "myRIO_BRig_RT_dataLC_ENL1_Probability_NS_l2.vi"() -> ("output_ENL1_Probability_NS_l2"=w434:i32)  [unwired: 11 in]
              n287 = call "myRIO_BRig_RT_dataLC_Cue1_OnOff_Switch_l2.vi"() -> ("output_Cue1_OnOff_Switch_l2"=w425:i32)  [unwired: 11 in]
              n288 = call "myRIO_BRig_RT_dataLC_Cue1_Tdelay_Switch_l2.vi"() -> ("output_Cue1_Tdelay_Switch_l2"=w426:i32)  [unwired: 11 in]
              n289 = call "myRIO_BRig_RT_dataLC_Cue1_Block_Switch_l2.vi"() -> ("output_Cue1_Block_Switch_l2"=w427:i32)  [unwired: 11 in]
              n290 = call "myRIO_BRig_RT_dataLC_Cue1_Count_Switch_l2.vi"() -> ("output_Cue1_Count_Switch_l2"=w428:i32)  [unwired: 11 in]
              n291 = call "myRIO_BRig_RT_dataLC_Cue1_Probability_Switch_l2.vi"() -> ("output_Cue1_l2_First_Probability"=w429:i32)  [unwired: 11 in]
              n292 = call "myRIO_BRig_RT_dataLC_Cue1_OnOff_NS_l2.vi"() -> ("output_Cue1_OnOff_NS_l2"=w420:i32)  [unwired: 11 in]
              n293 = call "myRIO_BRig_RT_dataLC_Cue1_Tdelay_NS_l2.vi"() -> ("output_Cue1_Tdelay_NS_l2"=w421:i32)  [unwired: 11 in]
              n294 = call "myRIO_BRig_RT_dataLC_Cue1_Block_NS_l2.vi"() -> ("output_Cue1_Block_NS_l2"=w422:i32)  [unwired: 11 in]
              n295 = call "myRIO_BRig_RT_dataLC_Cue1_Count_NS_l2.vi"() -> ("output_Cue1_Count_NS_l2"=w423:i32)  [unwired: 11 in]
              n296 = call "myRIO_BRig_RT_dataLC_Cue1_Probability_NS_l2.vi"() -> ("output_Cue1_l2_All_Probability"=w424:i32)  [unwired: 11 in]
              n297 = call "myRIO_BRig_RT_dataLC_ENL1_delayOpt_Switch_l2.vi"() -> ("output_ENL1_delayOpt_Switch_l2"=w416:i32)  [unwired: 11 in]
              n298 = call "myRIO_BRig_RT_dataLC_ENL1_delayOpt_NS_l2.vi"() -> ("output_ENL1_delayOpt_NS_l2"=w417:i32)  [unwired: 11 in]
              n299 = call "myRIO_BRig_RT_dataLC_Cue1_delayOpt_Switch_l2.vi"() -> ("output_Cue1_delayOpt_Switch_l2"=w418:i32)  [unwired: 11 in]
              n300 = call "myRIO_BRig_RT_dataLC_Cue1_delayOpt_NS_l2.vi"() -> ("output_Cue1_delayOpt_NS_l2"=w419:i32)  [unwired: 11 in]
              n301 = Index Array(array=w469, index #1=w435, index #2=w436, index #3=w437, index #4=w438, index #5=w439, index #6=w430, index #7=w431, index #8=w432, index #9=w433, index #10=w434, index #11=w425, index #12=w426, index #13=w427, index #14=w428, index #15=w429, index #16=w420, index #17=w421, index #18=w422, index #19=w423, index #20=w424, index #21=w416, index #22=w417, index #23=w418, index #24=w419) -> (element #1=w467:u16, element #2=w466:u16, element #3=w465:u16, element #4=w464:u16, element #5=w463:u16, element #6=w462:u16, element #7=w461:u16, element #8=w460:u16, element #9=w459:u16, element #10=w458:u16, element #11=w457:u16, element #12=w456:u16, element #13=w455:u16, element #14=w454:u16, element #15=w453:u16, element #16=w452:u16, element #17=w451:u16, element #18=w450:u16, element #19=w449:u16, element #20=w448:u16, element #21=w443:u16, element #22=w442:u16, element #23=w441:u16, element #24=w440:u16)
              n302 = Not Equal To 0?(x=w467) -> (x != 0?=w471:bool)
              n303 = Not Equal To 0?(x=w462) -> (x != 0?=w470:bool)
              n304 = Not Equal To 0?(x=w457) -> (x != 0?=w473:bool)
              n305 = Not Equal To 0?(x=w452) -> (x != 0?=w472:bool)
              n306 = Not Equal To 0?(x=w443) -> (x != 0?=w445:bool)
              n307 = Not Equal To 0?(x=w442) -> (x != 0?=w446:bool)
              n308 = Not Equal To 0?(x=w441) -> (x != 0?=w447:bool)
              n309 = Not Equal To 0?(x=w440) -> (x != 0?=w444:bool)
              n310 = local write "LC_ENL1_OnOff_Switch_l2"(w471) -> ()
              n311 = local write "LC_ENL1_Tdelay_Switch_l2"(w466) -> ()
              n312 = local write "LC_ENL1_Block_Switch_l2"(w465) -> ()
              n313 = local write "LC_ENL1_Count_Switch_l2"(w464) -> ()
              n314 = local write "LC_ENL1_Probability_Switch_l2"(w463) -> ()
              n315 = local write "LC_ENL1_OnOff_NS_l2"(w470) -> ()
              n316 = local write "LC_ENL1_Tdelay_NS_l2"(w461) -> ()
              n317 = local write "LC_ENL1_Block_NS_l2"(w460) -> ()
              n318 = local write "LC_ENL1_Count_NS_l2"(w459) -> ()
              n319 = local write "LC_ENL1_Probability_NS_l2"(w458) -> ()
              n320 = local write "LC_Cue1_OnOff_Switch_l2"(w473) -> ()
              n321 = local write "LC_Cue1_Tdelay_Switch_l2"(w456) -> ()
              n322 = local write "LC_Cue1_Block_Switch_l2"(w455) -> ()
              n323 = local write "LC_Cue1_Count_Switch_l2"(w454) -> ()
              n324 = local write "LC_Cue1_Probability_Switch_l2"(w453) -> ()
              n325 = local write "LC_Cue1_OnOff_NS_l2"(w472) -> ()
              n326 = local write "LC_Cue1_Tdelay_NS_l2"(w451) -> ()
              n327 = local write "LC_Cue1_Block_NS_l2"(w450) -> ()
              n328 = local write "LC_Cue1_Count_NS_l2"(w449) -> ()
              n329 = local write "LC_Cue1_Probability_NS_l2"(w448) -> ()
              n330 = local write "LC_ENL1_delayOpt_Switch_l2"(w445) -> ()
              n331 = local write "LC_ENL1_delayOpt_NS_l2"(w446) -> ()
              n332 = local write "LC_Cue1_delayOpt_Switch_l2"(w447) -> ()
              n333 = local write "LC_Cue1_delayOpt_NS_l2"(w444) -> ()
            }
            frame "UploadSettings_dataLC_2" {
              # "Count"
              # "Tdelay"
              # "Prob"
              # "OnOff"
              # "Block"
              # "Selection NonSwitch"
              # "Count"
              # "Tdelay"
              # "Prob"
              # "OnOff"
              # "Block"
              # "Selection Switch"
              # "Trial"
              # "Tdelay"
              # "Prob"
              # "OnOff"
              # "Block"
              # "Wrong"
              # "Reward"
              # "Trial"
              # "Tdelay"
              # "Prob"
              # "OnOff"
              # "Block"
              n334 = call "myRIO_BRig_RT_dataLC_Reward_OnOff_l1.vi"() -> ("output_Reward_OnOff_l1"=w516:i32)  [unwired: 11 in]
              n335 = call "myRIO_BRig_RT_dataLC_Reward_Tdelay_l1.vi"() -> ("output_Reward_Tdelay_l1"=w515:i32)  [unwired: 11 in]
              n336 = call "myRIO_BRig_RT_dataLC_Reward_Block_l1.vi"() -> ("output_Reward_Block_l1"=w514:i32)  [unwired: 11 in]
              n337 = call "myRIO_BRig_RT_dataLC_Reward_Trial_l1.vi"() -> ("output_Reward_Trial_l1"=w513:i32)  [unwired: 11 in]
              n338 = call "myRIO_BRig_RT_dataLC_Reward_Probability_l1.vi"() -> ("output_Reward_Probability_l1"=w512:i32)  [unwired: 11 in]
              n339 = call "myRIO_BRig_RT_dataLC_Wrong_OnOff_l1.vi"() -> ("output_Wrong_OnOff_l1"=w505:i32)  [unwired: 11 in]
              n340 = call "myRIO_BRig_RT_dataLC_Wrong_Tdelay_l1.vi"() -> ("output_Wrong_Tdelay_l1"=w504:i32)  [unwired: 11 in]
              n341 = call "myRIO_BRig_RT_dataLC_Wrong_Block_l1.vi"() -> ("output_Wrong_Block_l1"=w503:i32)  [unwired: 11 in]
              n342 = call "myRIO_BRig_RT_dataLC_Wrong_Trial_l1.vi"() -> ("output_Wrong_Trial_l1"=w502:i32)  [unwired: 11 in]
              n343 = call "myRIO_BRig_RT_dataLC_Wrong_Probability_l1.vi"() -> ("output_Wrong_Probability_l1"=w501:i32)  [unwired: 11 in]
              n344 = call "myRIO_BRig_RT_dataLC_Selection_OnOff_Switch_l1.vi"() -> ("output_Selection_OnOff_Switch_l1"=w496:i32)  [unwired: 11 in]
              n345 = call "myRIO_BRig_RT_dataLC_Selection_Tdelay_Switch_l1.vi"() -> ("output_Selection_Tdelay_Switch_l1"=w495:i32)  [unwired: 11 in]
              n346 = call "myRIO_BRig_RT_dataLC_Selection_Block_Switch_l1.vi"() -> ("output_Selection_Block_Switch_l1"=w494:i32)  [unwired: 11 in]
              n347 = call "myRIO_BRig_RT_dataLC_Selection_Count_Switch_l1.vi"() -> ("output_Selection_Count_Switch_l1"=w493:i32)  [unwired: 11 in]
              n348 = call "myRIO_BRig_RT_dataLC_Selection_Probability_Switch_l1.vi"() -> ("output_Selection_Probability_Switch_l1"=w492:i32)  [unwired: 11 in]
              n349 = call "myRIO_BRig_RT_dataLC_Selection_OnOff_NS_l1.vi"() -> ("output_Selection_OnOff_NS_l1"=w491:i32)  [unwired: 11 in]
              n350 = call "myRIO_BRig_RT_dataLC_Selection_Tdelay_NS_l1.vi"() -> ("output_Selection_Tdelay_NS_l1"=w490:i32)  [unwired: 11 in]
              n351 = call "myRIO_BRig_RT_dataLC_Selection_Block_NS_l1.vi"() -> ("output_Selection_Block_NS_l1"=w489:i32)  [unwired: 11 in]
              n352 = call "myRIO_BRig_RT_dataLC_Selection_Count_NS_l1.vi"() -> ("output_Selection_Count_NS_l1"=w488:i32)  [unwired: 11 in]
              n353 = call "myRIO_BRig_RT_dataLC_Selection_Probability_NS_l1.vi"() -> ("output_Selection_Probability_NS_l1"=w487:i32)  [unwired: 11 in]
              n354 = Index Array(array=w517, index #1=w516, index #2=w515, index #3=w514, index #4=w513, index #5=w512, index #6=w505, index #7=w504, index #8=w503, index #9=w502, index #10=w501, index #11=w496, index #12=w495, index #13=w494, index #14=w493, index #15=w492, index #16=w491, index #17=w490, index #18=w489, index #19=w488, index #20=w487) -> (element #1=w511:u16, element #2=w510:u16, element #3=w509:u16, element #4=w508:u16, element #5=w507:u16, element #6=w506:u16, element #7=w500:u16, element #8=w499:u16, element #9=w498:u16, element #10=w497:u16, element #11=w484:u16, element #12=w483:u16, element #13=w482:u16, element #14=w481:u16, element #15=w480:u16, element #16=w479:u16, element #17=w478:u16, element #18=w477:u16, element #19=w476:u16, element #20=w475:u16)
              n355 = Not Equal To 0?(x=w511) -> (x != 0?=w519:bool)
              n356 = Not Equal To 0?(x=w506) -> (x != 0?=w518:bool)
              n357 = Not Equal To 0?(x=w484) -> (x != 0?=w486:bool)
              n358 = Not Equal To 0?(x=w479) -> (x != 0?=w485:bool)
              n359 = local write "LC_Reward_OnOff_l1"(w519) -> ()
              n360 = local write "LC_Reward_Tdelay_l1"(w510) -> ()
              n361 = local write "LC_Reward_Block_l1"(w509) -> ()
              n362 = local write "LC_Reward_Trial_l1"(w508) -> ()
              n363 = local write "LC_Reward_Probability_l1"(w507) -> ()
              n364 = local write "LC_Wrong_OnOff_l1"(w518) -> ()
              n365 = local write "LC_Wrong_Tdelay_l1"(w500) -> ()
              n366 = local write "LC_Wrong_Block_l1"(w499) -> ()
              n367 = local write "LC_Wrong_Trial_l1"(w498) -> ()
              n368 = local write "LC_Wrong_Probability_l1"(w497) -> ()
              n369 = local write "LC_Sel_OnOff_Switch_l1"(w486) -> ()
              n370 = local write "LC_Sel_Tdelay_Switch_l1"(w483) -> ()
              n371 = local write "LC_Sel_Block_Switch_l1"(w482) -> ()
              n372 = local write "LC_Sel_Count_Switch_l1"(w481) -> ()
              n373 = local write "LC_Sel_Probability_Switch_l1"(w480) -> ()
              n374 = local write "LC_Sel_OnOff_NS_l1"(w485) -> ()
              n375 = local write "LC_Sel_Tdelay_NS_l1"(w478) -> ()
              n376 = local write "LC_Sel_Block_NS_l1"(w477) -> ()
              n377 = local write "LC_Sel_Count_NS_l1"(w476) -> ()
              n378 = local write "LC_Sel_Probability_NS_l1"(w475) -> ()
            }
            frame "UploadSettings_dataLC_4" {
              # "Count"
              # "Tdelay"
              # "Prob"
              # "OnOff"
              # "Block"
              # "Selection NonSwitch"
              # "Count"
              # "Tdelay"
              # "Prob"
              # "OnOff"
              # "Block"
              # "Selection Switch"
              # "Trial"
              # "Tdelay"
              # "Prob"
              # "OnOff"
              # "Block"
              # "Wrong"
              # "Reward"
              # "Trial"
              # "Tdelay"
              # "Prob"
              # "OnOff"
              # "Block"
              n379 = call "myRIO_BRig_RT_dataLC_Reward_OnOff_l2.vi"() -> ("output_Reward_OnOff_l2"=w527:i32)  [unwired: 11 in]
              n380 = call "myRIO_BRig_RT_dataLC_Reward_Tdelay_l2.vi"() -> ("output_Reward_Tdelay_l2"=w528:i32)  [unwired: 11 in]
              n381 = call "myRIO_BRig_RT_dataLC_Reward_Block_l2.vi"() -> ("output_Reward_Block_l2"=w529:i32)  [unwired: 11 in]
              n382 = call "myRIO_BRig_RT_dataLC_Reward_Trial_l2.vi"() -> ("output_Reward_Trial_l2"=w530:i32)  [unwired: 11 in]
              n383 = call "myRIO_BRig_RT_dataLC_Reward_Probability_l2.vi"() -> ("output_Reward_Probability_l2"=w531:i32)  [unwired: 11 in]
              n384 = call "myRIO_BRig_RT_dataLC_Wrong_OnOff_l2.vi"() -> ("output_Wrong_OnOff_l2"=w522:i32)  [unwired: 11 in]
              n385 = call "myRIO_BRig_RT_dataLC_Wrong_Tdelay_l2.vi"() -> ("output_Wrong_Tdelay_l2"=w523:i32)  [unwired: 11 in]
              n386 = call "myRIO_BRig_RT_dataLC_Wrong_Block_l2.vi"() -> ("output_Wrong_Block_l2"=w524:i32)  [unwired: 11 in]
              n387 = call "myRIO_BRig_RT_dataLC_Wrong_Trial_l2.vi"() -> ("output_Wrong_Trial_l2"=w525:i32)  [unwired: 11 in]
              n388 = call "myRIO_BRig_RT_dataLC_Wrong_Probability_l2.vi"() -> ("output_Wrong_Probability_l2"=w526:i32)  [unwired: 11 in]
              n389 = call "myRIO_BRig_RT_dataLC_Selection_OnOff_Switch_l2.vi"() -> ("output_Selection_OnOff_Switch_l2"=w537:i32)  [unwired: 11 in]
              n390 = call "myRIO_BRig_RT_dataLC_Selection_Tdelay_Switch_l2.vi"() -> ("output_Selection_Tdelay_Switch_l2"=w538:i32)  [unwired: 11 in]
              n391 = call "myRIO_BRig_RT_dataLC_Selection_Block_Switch_l2.vi"() -> ("output_Selection_Block_Switch_l2"=w539:i32)  [unwired: 11 in]
              n392 = call "myRIO_BRig_RT_dataLC_Selection_Count_Switch_l2.vi"() -> ("output_Selection_Count_Switch_l2"=w540:i32)  [unwired: 11 in]
              n393 = call "myRIO_BRig_RT_dataLC_Selection_Probability_Switch_l2.vi"() -> ("output_Selection_Probability_Switch_l1"=w541:i32)  [unwired: 11 in]
              n394 = call "myRIO_BRig_RT_dataLC_Selection_OnOff_NS_l2.vi"() -> ("output_Selection_OnOff_NS_l2"=w532:i32)  [unwired: 11 in]
              n395 = call "myRIO_BRig_RT_dataLC_Selection_Tdelay_NS_l2.vi"() -> ("output_Selection_Tdelay_NS_l2"=w533:i32)  [unwired: 11 in]
              n396 = call "myRIO_BRig_RT_dataLC_Selection_Block_NS_l2.vi"() -> ("output_Selection_Block_NS_l2"=w534:i32)  [unwired: 11 in]
              n397 = call "myRIO_BRig_RT_dataLC_Selection_Count_NS_l2.vi"() -> ("output_Selection_Count_NS_l2"=w535:i32)  [unwired: 11 in]
              n398 = call "myRIO_BRig_RT_dataLC_Selection_Probability_NS_l2.vi"() -> ("output_Selection_Probability_NS_l2"=w536:i32)  [unwired: 11 in]
              n399 = Index Array(array=w564, index #1=w527, index #2=w528, index #3=w529, index #4=w530, index #5=w531, index #6=w522, index #7=w523, index #8=w524, index #9=w525, index #10=w526, index #11=w537, index #12=w538, index #13=w539, index #14=w540, index #15=w541, index #16=w532, index #17=w533, index #18=w534, index #19=w535, index #20=w536) -> (element #1=w563:u16, element #2=w562:u16, element #3=w561:u16, element #4=w560:u16, element #5=w559:u16, element #6=w558:u16, element #7=w557:u16, element #8=w556:u16, element #9=w555:u16, element #10=w554:u16, element #11=w551:u16, element #12=w550:u16, element #13=w549:u16, element #14=w548:u16, element #15=w547:u16, element #16=w546:u16, element #17=w545:u16, element #18=w544:u16, element #19=w543:u16, element #20=w542:u16)
              n400 = Not Equal To 0?(x=w563) -> (x != 0?=w566:bool)
              n401 = Not Equal To 0?(x=w558) -> (x != 0?=w565:bool)
              n402 = Not Equal To 0?(x=w551) -> (x != 0?=w553:bool)
              n403 = Not Equal To 0?(x=w546) -> (x != 0?=w552:bool)
              n404 = local write "LC_Reward_OnOff_l2"(w566) -> ()
              n405 = local write "LC_Reward_Tdelay_l2"(w562) -> ()
              n406 = local write "LC_Reward_Block_l2"(w561) -> ()
              n407 = local write "LC_Reward_Trial_l2"(w560) -> ()
              n408 = local write "LC_Reward_Probability_l2"(w559) -> ()
              n409 = local write "LC_Wrong_OnOff_l2"(w565) -> ()
              n410 = local write "LC_Wrong_Tdelay_l2"(w557) -> ()
              n411 = local write "LC_Wrong_Block_l2"(w556) -> ()
              n412 = local write "LC_Wrong_Trial_l2"(w555) -> ()
              n413 = local write "LC_Wrong_Probability_l2"(w554) -> ()
              n414 = local write "LC_Sel_OnOff_Switch_l2"(w553) -> ()
              n415 = local write "LC_Sel_Tdelay_Switch_l2"(w550) -> ()
              n416 = local write "LC_Sel_Block_Switch_l2"(w549) -> ()
              n417 = local write "LC_Sel_Count_Switch_l2"(w548) -> ()
              n418 = local write "LC_Sel_Probability_Switch_l2"(w547) -> ()
              n419 = local write "LC_Sel_OnOff_NS_l2"(w552) -> ()
              n420 = local write "LC_Sel_Tdelay_NS_l2"(w545) -> ()
              n421 = local write "LC_Sel_Block_NS_l2"(w544) -> ()
              n422 = local write "LC_Sel_Count_NS_l2"(w543) -> ()
              n423 = local write "LC_Sel_Probability_NS_l2"(w542) -> ()
            }
            frame "UploadSettings_dataMTrig_1" {
              # "Tdelay_R"
              # "Tdelay_L"
              # "Tcycle_R"
              # "Tcycle_L"
              # "RewCalib_nCycle_R"
              # "RewCalib_nCycle_L"
              # "Solenoid"
              # "Laser_Tcycle"
              n424 = call "myRIO_BRig_RT_dataMTrig_Laser_Tcycle.vi"() -> ("output_Laser_Tcycle"=w576:i32)  [unwired: 11 in]
              n425 = call "myRIO_BRig_RT_dataMTrig_Solenoid_RewCalib_nCycle__L.vi"() -> ("output_Solenoid_RewCalib_nCycle__L"=w575:i32)  [unwired: 11 in]
              n426 = call "myRIO_BRig_RT_dataMTrig_Solenoid_RewCalib_nCycle__R.vi"() -> ("output_Solenoid_RewCalib_nCycle__R"=w574:i32)  [unwired: 11 in]
              n427 = call "myRIO_BRig_RT_dataMTrig_Solenoid_Tdelay__L.vi"() -> ("output_Solenoid_Tdelay__L"=w571:i32)  [unwired: 11 in]
              n428 = call "myRIO_BRig_RT_dataMTrig_Solenoid_Tdelay__R.vi"() -> ("output_Solenoid_Tdelay__R"=w570:i32)  [unwired: 11 in]
              n429 = call "myRIO_BRig_RT_dataMTrig_Solenoid_Tcycle__L.vi"() -> ("output_Solenoid_Tcycle__L"=w573:i32)  [unwired: 11 in]
              n430 = call "myRIO_BRig_RT_dataMTrig_Solenoid_Tcycle__R.vi"() -> ("output_Solenoid_Tcycle__R"=w572:i32)  [unwired: 11 in]
              n431 = Index Array(array=w569, index #1=w576, index #2=w575, index #3=w574, index #4=w573, index #5=w572, index #6=w571, index #7=w570) -> (element #1=w583:u16, element #2=w582:u16, element #3=w581:u16, element #4=w580:u16, element #5=w579:u16, element #6=w578:u16, element #7=w577:u16)
              n432 = Replace Array Subset(array=w585, new element #1=w583, index #1=w576, new element #2=w582, index #2=w575, new element #3=w581, index #3=w574, new element #4=w580, index #4=w573, new element #5=w579, index #5=w572, new element #6=w578, index #6=w571, new element #7=w577, index #7=w570) -> (w584:u16[])
              n433 = local write "MTrig_Solenoid_Tcycle__L"(w580) -> ()
              n434 = local write "MTrig_Solenoid_Tcycle__R"(w579) -> ()
              n435 = local write "MTrig_Laser_Tcycle"(w583) -> ()
            }
            frame "Idle" {
              # "There are a number of tasks we need to perform\nwhile idling. To preserve our timing loop, we\nbreak up the IDLE state into smaller states"
              # "Laser_Tcycle"
              # "Audio_Tcycle_R"
              # "Audio_Tcycle_L"
              n436 = local read "Laser_power_min_l1"() -> (w593:dbl)
              n437 = local read "Laser_power_min_l2"() -> (w591:dbl)
              n438 = local read "Audio_Amp__R"() -> (w595:u16)
              n439 = local read "Audio_Amp__L"() -> (w597:u16)
              n440 = local read "Audio_Freq__R"() -> (w594:u8)
              n441 = local read "Audio_Freq__L"() -> (w596:u8)
              n442 = Select(t=myRIO_BRig_RT__Case_NonExp_stateList."SendData" ("Enum"), s="SendData", f=myRIO_BRig_RT__Case_NonExp_stateList."Idle_2" ("Enum")) -> (s? t:f=w602:T1)
              n443 = call "myRIO__convert__Voltage_to_FPGAvalue.vi"("input_voltage"=w593) -> ("output_PortC"=w592:i16)  [unwired: 9 in, 1 out]
              n444 = call "myRIO__convert__Voltage_to_FPGAvalue.vi"("input_voltage"=w591) -> ("output_PortC"=w590:i16)  [unwired: 9 in, 1 out]
              n445 = Select(t=myRIO_BRig_RT__Case_NonExp_stateList."TestConnection" ("Enum"), s="TestConnection", f=w602) -> (s? t:f=w606:T1)
              n446 = xnode "Read/Write Control"("FPGA VI Reference In"=w599, "error in"=w598, "audioAmp_L"=w597, "audioFreq_L_kHz"=w596, "audioAmp_R"=w595, "audioFreq_R_kHz"=w594, "AnaOut_0"=w592, "AnaOut_1"=w590) -> ("error out"=w589:errorcluster)  [unwired: 1 out]
              n447 = call "myRIO_BRig_RT_dataMTrig_Audio_Tcycle__L.vi"() -> ("output_Audio_Tcycle__L"=w613:i32)  [unwired: 11 in]
              n448 = call "myRIO_BRig_RT_dataMTrig_Audio_Tcycle__R.vi"() -> ("output_Audio_Tcycle__R"=w612:i32)  [unwired: 11 in]
              n449 = call "myRIO_BRig_RT_dataMTrig_Laser_Tcycle.vi"() -> ("output_Laser_Tcycle"=w611:i32)  [unwired: 11 in]
              n450 = call "myRIO_BRig_RT_dataMTrig_CueLed_Tcycle.vi"() -> ("output_CueLed_Tcycle"=w588:i32)  [unwired: 11 in]
              n451 = local write "error out"(w589) -> ()
              n452 = local read "Tcycle_Cue_Audio_min"() -> (w601:u16)
              n453 = local read "MTrig_Laser_Tcycle"() -> (w600:u16)
              n454 = local read "Tcycle_Cue_LED_min"() -> (w587:u16)
              n455 = Replace Array Subset(array=w609, new element #1=w601, index #1=w613, new element #2=w601, index #2=w612, new element #3=w600, index #3=w611, new element #4=w587, index #4=w588) -> (w610:u16[])
            }
            frame "Idle_2" {
              w636 = u16 0 ("t")
              # "There are a number of tasks we need to perform\nwhile idling. To preserve our timing loop, we\nbreak up the IDLE state into smaller states"
              # "Ncycles"
              # "Ncycles"
              # "RewCalib"
              # "RewCalib"
              # "Solenoid R"
              # "Solenoid L"
              n456 = local read "MTrig_Laser_Switch"() -> (w629:bool)
              n457 = local read "count_warmup_R"() -> (w635:u16)
              n458 = local read "count_warmup_L"() -> (w640:u16)
              n459 = call "myRIO_BRig_RT_dataMTrig_Solenoid_RewCalib_OnOff__R.vi"() -> ("output_Solenoid_RewCalib_OnOff__R"=w651:i32)  [unwired: 11 in]
              n460 = call "myRIO_BRig_RT_dataMTrig_Solenoid_N__R.vi"() -> ("output_Solenoid_N__R"=w650:i32)  [unwired: 11 in]
              n461 = call "myRIO_BRig_RT_dataMTrig_Solenoid_RewCalib_OnOff__L.vi"() -> ("output_Solenoid_RewCalib_OnOff__L"=w666:i32)  [unwired: 11 in]
              n462 = call "myRIO_BRig_RT_dataMTrig_Solenoid_N__L.vi"() -> ("output_Solenoid_N__L"=w654:i32)  [unwired: 11 in]
              n463 = case shown="False" w629 {
                tunnel: "LR_reward_Event" -> [w672 w676]
                tunnel: "LR_wrong_Event" -> [w671 w675]
                tunnel: "LR_reward_Laser" -> [w670 w674]
                tunnel: "LR_wrong_Laser" -> [w669 w673]
                tunnel: [w672 _] -> w624
                tunnel: [w671 _] -> w623
                tunnel: [w670 _] -> w622
                tunnel: [w669 _] -> w621
                tunnel: [_ w676] -> w620
                tunnel: [_ w675] -> w619
                tunnel: [_ w674] -> w618
                tunnel: [_ w673] -> w617
                frame False {
                }
                frame True {
                }
              }
              n464 = Index Array(array=w657, index #1=w666, index #2=w654, index #3=w651, index #4=w650) -> (element #1=w653:u16, element #2=w648:u16, element #3=w649:u16, element #4=w647:u16)
              n465 = Select(t=w636, s="count_warmup_L_reset", f=w640) -> (s? t:f=→"count_warmup_L":u16)
              n466 = Select(t=w636, s="count_warmup_R_reset", f=w635) -> (s? t:f=→"count_warmup_R":u16)
              n467 = local read "RewCalib_Trig_L"() -> (w646:bool)
              n468 = local read "RewCalib_Trig_R"() -> (w645:bool)
              n469 = Equal To 0?(x=w648) -> (x = 0?=w656:bool)
              n470 = Equal To 0?(x=w647) -> (x = 0?=w655:bool)
              n471 = Not Equal To 0?(x=w649) -> (x != 0?=w667:bool)
              n472 = Not Equal To 0?(x=w653) -> (x != 0?=w668:bool)
              n473 = And(x=w656, y=w655) -> (x .and. y?=w660:bool)
              n474 = Or(x=w646, y=w645) -> (x .or. y?=w661:bool)
              n475 = Not Exclusive Or(1:w668, 2:w646) -> (0:w663:bool)
              n476 = xnode "Read/Write Control"("FPGA VI Reference In"=w615, "error in"=w616, "Left(F)_or_Right(T)"="Left(F)_or_Right(T)", "SelectionState"="SelectionState", "ignoreWrong"="ignoreWrong", "LR_reward_Event_l1"=w624, "LR_wrong_Event_l1"=w623, "LR_reward_Laser_l1"=w622, "LR_wrong_Laser_l1"=w621, "LR_reward_Event_l2"=w620, "LR_wrong_Event_l2"=w619, "LR_reward_Laser_l2"=w618, "LR_wrong_laser_l2"=w617) -> ("error out"=w614:errorcluster, "SelectReward"=→"SelectReward":bool, "SelectWrong"=→"SelectWrong":bool)  [unwired: 1 out]
              n477 = Not Exclusive Or(1:w667, 2:w645) -> (0:w665:bool)
              n478 = And(x=w661, y=w660) -> (x .and. y?=w643:bool)
              n479 = Not(x=w663) -> (.not. x?=w662:bool)
              n480 = Not(x=w665) -> (.not. x?=w664:bool)
              n481 = Or(x=w662, y=w664) -> (x .or. y?=w644:bool)
              n482 = Or(x=w643, y=w644) -> (x .or. y?=w659:bool)
              n483 = local write "error out"(w614) -> ()
              n484 = Select(t=myRIO_BRig_RT__Case_NonExp_stateList."RewardCalibration_pre" ("Enum"), s=w659, f=myRIO_BRig_RT__Case_NonExp_stateList."Idle_3" ("Enum")) -> (s? t:f=w642:T1)
            }
            frame "Idle_3" {
              # "There are a number of tasks we need to perform\nwhile idling. To preserve our timing loop, we\nbreak up the IDLE state into smaller states"
              n485 = local read "Laser_Tshutter_l1"() -> (w695:dbl)
              n486 = local read "Laser_duration_l1"() -> (w694:u16)
              n487 = local read "Laser_Tshutter_l2"() -> (w691:dbl)
              n488 = local read "Laser_duration_l2"() -> (w690:u16)
              n489 = local read "Laser_Tpeak_l1"() -> (w697:dbl)
              n490 = local read "Laser_Tpeak_l2"() -> (w693:dbl)
              n491 = local read "CueLed_Tpeak"() -> (w688:dbl)
              n492 = local read "Laser_Freq_l1"() -> (w696:dbl)
              n493 = local read "Laser_Freq_l2"() -> (w692:dbl)
              n494 = local read "CueLed_Freq"() -> (w687:dbl)
              n495 = local read "FPGA_count2ms"() -> (w689:dbl)
              n496 = To Unsigned Word Integer(number=w689) -> (unsigned 16bit integer=w698:u16)
              n497 = call "myRIO_BRig_RT__calc_laser_FPGA_N.vi"("input_FPGA_ms2count"=w689, "input_Tpeak"=w697, "input_Freq"=w696, "input_Tshutter"=w695, "input_duration"=w694) -> ("output_laser_Npeak"=w686:u32, "output_laser_Nvalley"=w684:u32, "output_laser_Nshutter"=w682:u32, "output_laser_Nduration"=w680:u32)  [unwired: 6 in, 1 out]
              n498 = call "myRIO_BRig_RT__calc_laser_FPGA_N.vi"("input_FPGA_ms2count"=w689, "input_Tpeak"=w693, "input_Freq"=w692, "input_Tshutter"=w691, "input_duration"=w690) -> ("output_laser_Npeak"=w685:u32, "output_laser_Nvalley"=w683:u32, "output_laser_Nshutter"=w681:u32, "output_laser_Nduration"=w679:u32)  [unwired: 6 in, 1 out]
              n499 = call "myRIO_BRig_RT__calc_laser_FPGA_N__CueLed.vi"("input_FPGA_ms2count"=w689, "input_Tpeak"=w688, "input_Freq"=w687) -> ("output_laser_Npeak"=w678:u32, "output_laser_Nvalley"=w677:u32)  [unwired: 11 in]
              n500 = xnode "Read/Write Control"("FPGA VI Reference In"=w703, "error in"=w702, "k1__counter_per_ms"=w698, "LC_nPeak_l1"=w686, "LC_nPeak_l2"=w685, "LC_nValley_l1"=w684, "LC_nValley_l2"=w683, "LC_nShutter_l1"=w682, "LC_nShutter_l2"=w681, "LR_reward_nTotal_l1"=w680, "LR_wrong_nTotal_l1"=w680, "LR_reward_nTotal_l2"=w679, "LR_wrong_nTotal_l2"=w679, "CueLed_nPeak"=w678, "CueLed_nValley"=w677) -> ("error out"=w699:errorcluster)  [unwired: 1 out]
              n501 = local write "error out"(w699) -> ()
            }
            frame "Idle_4" {
              w725 = u8 0 ("f")
              # "There are a number of tasks we need to perform\nwhile idling. To preserve our timing loop, we\nbreak up the IDLE state into smaller states"
              n502 = local read "MTrig_Solenoid_trig__L"() -> (w716:bool)
              n503 = local read "MTrig_Solenoid_trig__R"() -> (w726:bool)
              n504 = local read "warmupType"() -> (w709:u8)
              n505 = local read "warmup"() -> (w718:bool)
              n506 = Not Equal To 0?(x=w709) -> (x != 0?=w708:bool)
              n507 = Not(x=w708) -> (.not. x?=w719:bool)
              n508 = Select(t=u8 1, s=w716, f=w725) -> (s? t:f=w724:u8)
              n509 = Select(t=u8 2, s=w726, f=w725) -> (s? t:f=w723:u8)
              n510 = And(x=w718, y=w719) -> (x .and. y?=w717:bool)
              n511 = And(x=w718, y=w708) -> (x .and. y?=w712:bool)
              n512 = Add(x=w724, y=w723) -> (x+y=w722:u8)
              n513 = case shown="3" w722 {
                tunnel: w721 -> [w729 w733 w766 w797]
                tunnel: [w729 w732 w765 w796] -> w720
                tunnel: w717 -> [_ w731 w764 w795]
                tunnel: [_ TRUE TRUE TRUE] -> w714
                frame 0, Default {
                }
                frame 1 {
                  n514 = case shown="False" w731 {
                    tunnel: w733 -> [w746 w761]
                    tunnel: [w745 w760] -> w732
                    frame True {
                      # "Audio_L"
                      # "Solenoid_L"
                      n515 = call "myRIO_BRig_RT_dataMTrig_Solenoid_N__L.vi"() -> ("output_Solenoid_N__L"=w743:i32)  [unwired: 11 in]
                      n516 = call "myRIO_BRig_RT_dataMTrig_Audio_N__L.vi"() -> ("output_Audio_N__L"=w741:i32)  [unwired: 11 in]
                      n517 = call "myRIO_BRig_RT_dataMTrig_Audio_N__R.vi"() -> ("output_Audio_N__R"=w736:i32)  [unwired: 11 in]
                      n518 = local read "sp_LeftSpout"() -> (w740:u16)
                      n519 = Index Array(array=w746, index #1=w743, index #2=w741, index #3=w736) -> (element #1=w744:u16, element #2=w739:u16, element #3=w738:u16)
                      n520 = Increment(x=w744) -> (x+1=w742:u16)
                      n521 = case shown="2" w740 {
                        tunnel: w739 -> [w749 w752 w754]
                        tunnel: w738 -> [w747 w751 w756]
                        tunnel: [w748 w752 w753] -> w737
                        tunnel: [w747 w750 w755] -> w735
                        frame 0, Default {
                          n522 = Increment(x=w749) -> (x+1=w748:u16)
                        }
                        frame 1 {
                          n523 = Increment(x=w751) -> (x+1=w750:u16)
                        }
                        frame 2 {
                          n524 = Increment(x=w756) -> (x+1=w755:u16)
                          n525 = Increment(x=w754) -> (x+1=w753:u16)
                        }
                      }
                      n526 = Replace Array Subset(array=w746, new element #1=w742, index #1=w743, new element #2=w737, index #2=w741, new element #3=w735, index #3=w736) -> (w745:u16[])
                    }
                    frame False {
                      # "Solenoid_L"
                      n527 = call "myRIO_BRig_RT_dataMTrig_Solenoid_N__L.vi"() -> ("output_Solenoid_N__L"=w758:i32)  [unwired: 11 in]
                      n528 = Index Array(array=w761, index=w758) -> (element=w759:u16)
                      n529 = Increment(x=w759) -> (x+1=w757:u16)
                      n530 = Replace Array Subset(array=w761, new element=w757, index=w758) -> (w760:u16[])
                    }
                  }
                  n531 = local write "MTrig_Solenoid_trig__L"(FALSE) -> ()
                }
                frame 2 {
                  n532 = case shown="True" w764 {
                    tunnel: w766 -> [w778 w793]
                    tunnel: [w777 w792] -> w765
                    frame True {
                      # "Solenoid_R"
                      n533 = call "myRIO_BRig_RT_dataMTrig_Solenoid_N__R.vi"() -> ("output_Solenoid_N__R"=w767:i32)  [unwired: 11 in]
                      n534 = call "myRIO_BRig_RT_dataMTrig_Audio_N__L.vi"() -> ("output_Audio_N__L"=w774:i32)  [unwired: 11 in]
                      n535 = call "myRIO_BRig_RT_dataMTrig_Audio_N__R.vi"() -> ("output_Audio_N__R"=w769:i32)  [unwired: 11 in]
                      n536 = local read "sp_RightSpout"() -> (w773:u16)
                      n537 = Index Array(array=w778, index #1=w767, index #2=w774, index #3=w769) -> (element #1=w776:u16, element #2=w772:u16, element #3=w771:u16)
                      n538 = Increment(x=w776) -> (x+1=w775:u16)
                      n539 = case shown="2" w773 {
                        tunnel: w772 -> [w781 w784 w786]
                        tunnel: w771 -> [w779 w783 w788]
                        tunnel: [w780 w784 w785] -> w770
                        tunnel: [w779 w782 w787] -> w768
                        frame 0, Default {
                          n540 = Increment(x=w781) -> (x+1=w780:u16)
                        }
                        frame 1 {
                          n541 = Increment(x=w783) -> (x+1=w782:u16)
                        }
                        frame 2 {
                          n542 = Increment(x=w788) -> (x+1=w787:u16)
                          n543 = Increment(x=w786) -> (x+1=w785:u16)
                        }
                      }
                      n544 = Replace Array Subset(array=w778, new element #1=w775, index #1=w767, new element #2=w770, index #2=w774, new element #3=w768, index #3=w769) -> (w777:u16[])
                    }
                    frame False {
                      # "Solenoid_R"
                      n545 = call "myRIO_BRig_RT_dataMTrig_Solenoid_N__R.vi"() -> ("output_Solenoid_N__R"=w789:i32)  [unwired: 11 in]
                      n546 = Index Array(array=w793, index=w789) -> (element=w791:u16)
                      n547 = Increment(x=w791) -> (x+1=w790:u16)
                      n548 = Replace Array Subset(array=w793, new element=w790, index=w789) -> (w792:u16[])
                    }
                  }
                  n549 = local write "MTrig_Solenoid_trig__R"(FALSE) -> ()
                }
                frame 3 {
                  w798 = FALSE
                  n550 = case shown="True" w795 {
                    tunnel: w797 -> [w812 w820]
                    tunnel: [w811 w819] -> w796
                    frame True {
                      # "Audio_R"
                      # "Solenoid_R"
                      # "Audio_L"
                      # "Solenoid_L"
                      n551 = call "myRIO_BRig_RT_dataMTrig_Solenoid_N__L.vi"() -> ("output_Solenoid_N__L"=w806:i32)  [unwired: 11 in]
                      n552 = call "myRIO_BRig_RT_dataMTrig_Audio_N__L.vi"() -> ("output_Audio_N__L"=w804:i32)  [unwired: 11 in]
                      n553 = call "myRIO_BRig_RT_dataMTrig_Solenoid_N__R.vi"() -> ("output_Solenoid_N__R"=w802:i32)  [unwired: 11 in]
                      n554 = call "myRIO_BRig_RT_dataMTrig_Audio_N__R.vi"() -> ("output_Audio_N__R"=w801:i32)  [unwired: 11 in]
                      n555 = Index Array(array=w812, index #1=w806, index #2=w804, index #3=w802, index #4=w801) -> (element #1=w810:u16, element #2=w809:u16, element #3=w808:u16, element #4=w807:u16)
                      n556 = Increment(x=w807) -> (x+1=w799:u16)
                      n557 = Increment(x=w810) -> (x+1=w805:u16)
                      n558 = Increment(x=w809) -> (x+1=w803:u16)
                      n559 = Increment(x=w808) -> (x+1=w800:u16)
                      n560 = Replace Array Subset(array=w812, new element #1=w805, index #1=w806, new element #2=w803, index #2=w804, new element #3=w800, index #3=w802, new element #4=w799, index #4=w801) -> (w811:u16[])
                    }
                    frame False {
                      # "Solenoid_R"
                      # "Solenoid_L"
                      n561 = call "myRIO_BRig_RT_dataMTrig_Solenoid_N__L.vi"() -> ("output_Solenoid_N__L"=w816:i32)  [unwired: 11 in]
                      n562 = call "myRIO_BRig_RT_dataMTrig_Solenoid_N__R.vi"() -> ("output_Solenoid_N__R"=w813:i32)  [unwired: 11 in]
                      n563 = Index Array(array=w820, index #1=w816, index #2=w813) -> (element #1=w818:u16, element #2=w817:u16)
                      n564 = Increment(x=w818) -> (x+1=w815:u16)
                      n565 = Increment(x=w817) -> (x+1=w814:u16)
                      n566 = Replace Array Subset(array=w820, new element #1=w815, index #1=w816, new element #2=w814, index #2=w813) -> (w819:u16[])
                    }
                  }
                  n567 = local write "MTrig_Solenoid_trig__L"(w798) -> ()
                  n568 = local write "MTrig_Solenoid_trig__R"(w798) -> ()
                }
              }
              n569 = local read "get_countPerMS"() -> (w707:bool)
              n570 = Select(t=myRIO_BRig_RT__Case_NonExp_stateList."Get_FPGA_count_per_ms" ("Enum"), s=w707, f=myRIO_BRig_RT__Case_NonExp_stateList."Idle_6" ("Enum")) -> (s? t:f=w705:T1)
              n571 = Select(t=myRIO_BRig_RT__Case_NonExp_stateList."Cue_pre", s=w712, f=myRIO_BRig_RT__Case_NonExp_stateList."DispenseWater_pre" ("Enum")) -> (s? t:f=w710:T1)
              n572 = Select(t=w710, s=w714, f=w705) -> (s? t:f=w715:T1)
            }
            frame "Idle_5" {
              w843 = u8 0 ("f")
              # "There are a number of tasks we need to perform\nwhile idling. To preserve our timing loop, we\nbreak up the IDLE state into smaller states"
              n573 = local read "MTrig_Solenoid_trig__L"() -> (w834:bool)
              n574 = local read "MTrig_Solenoid_trig__R"() -> (w844:bool)
              n575 = local read "warmupType"() -> (w822:u8)
              n576 = local read "Cue1Param_CueType_Switch"() -> (w821:u16)
              n577 = local read "warmup"() -> (w836:bool)
              n578 = Not Equal To 0?(x=w822) -> (x != 0?=w827:bool)
              n579 = Not(x=w827) -> (.not. x?=w837:bool)
              n580 = Select(t=u8 1, s=w834, f=w843) -> (s? t:f=w842:u8)
              n581 = Select(t=u8 2, s=w844, f=w843) -> (s? t:f=w841:u8)
              n582 = And(x=w836, y=w837) -> (x .and. y?=w835:bool)
              n583 = And(x=w836, y=w827) -> (x .and. y?=w830:bool)
              n584 = Add(x=w842, y=w841) -> (x+y=w840:u8)
              n585 = case shown="2" w840 {
                tunnel: w839 -> [w847 w852 w901 w951]
                tunnel: [w847 w851 w900 w950] -> w838
                tunnel: w835 -> [_ w850 w899 w949]
                tunnel: [_ TRUE TRUE TRUE] -> w832
                tunnel: w821 -> [_ w848 w897 w947]
                frame 0, Default {
                }
                frame 1 {
                  n586 = case shown="True" w850 {
                    tunnel: w852 -> [w857 w896]
                    tunnel: [w856 w895] -> w851
                    tunnel: w848 -> [w855 _]
                    frame True {
                      n587 = case shown="0, Default" w855 {
                        tunnel: [TRUE _ w889] -> w854
                        frame 0, Default {
                          # "Audio"
                        }
                        frame 1 {
                          # "LED"
                        }
                        frame 2 {
                          # "Audio or LED"
                          n588 = local read "Cue1Param_AudioLed_Probability_Switch"() -> (w891:u16)
                          n589 = call "myRIO__convert__Probability_to_TrueFalse.vi"("input_probability_u16"=w891) -> ("output_TF"=w890:bool)  [unwired: 10 in]
                          n590 = Not(x=w890) -> (.not. x?=w889:bool)
                        }
                      }
                      n591 = case shown="True" w854 {
                        tunnel: w857 -> [w869 w887]
                        tunnel: [w868 w886] -> w856
                        frame True {
                          n592 = call "myRIO_BRig_RT_dataMTrig_Solenoid_N__L.vi"() -> ("output_Solenoid_N__L"=w866:i32)  [unwired: 11 in]
                          n593 = call "myRIO_BRig_RT_dataMTrig_Audio_N__L.vi"() -> ("output_Audio_N__L"=w864:i32)  [unwired: 11 in]
                          n594 = call "myRIO_BRig_RT_dataMTrig_Audio_N__R.vi"() -> ("output_Audio_N__R"=w859:i32)  [unwired: 11 in]
                          n595 = local read "sp_LeftSpout"() -> (w863:u16)
                          n596 = Index Array(array=w869, index #1=w866, index #2=w864, index #3=w859) -> (element #1=w867:u16, element #2=w862:u16, element #3=w861:u16)
                          n597 = case shown="2" w863 {
                            tunnel: w862 -> [w872 w875 w877]
                            tunnel: w861 -> [w870 w874 w879]
                            tunnel: [w871 w875 w876] -> w860
                            tunnel: [w870 w873 w878] -> w858
                            frame 0, Default {
                              n598 = Increment(x=w872) -> (x+1=w871:u16)
                            }
                            frame 1 {
                              n599 = Increment(x=w874) -> (x+1=w873:u16)
                            }
                            frame 2 {
                              n600 = Increment(x=w879) -> (x+1=w878:u16)
                              n601 = Increment(x=w877) -> (x+1=w876:u16)
                            }
                          }
                          n602 = Increment(x=w867) -> (x+1=w865:u16)
                          n603 = Replace Array Subset(array=w869, new element #1=w865, index #1=w866, new element #2=w860, index #2=w864, new element #3=w858, index #3=w859) -> (w868:u16[])
                        }
                        frame False {
                          n604 = call "myRIO_BRig_RT_dataMTrig_Solenoid_N__L.vi"() -> ("output_Solenoid_N__L"=w884:i32)  [unwired: 11 in]
                          n605 = call "myRIO_BRig_RT_dataMTrig_CueLed_N.vi"() -> ("output_CueLed_N"=w882:i32)  [unwired: 11 in]
                          n606 = Index Array(array=w887, index #1=w884, index #2=w882) -> (element #1=w885:u16, element #2=w881:u16)
                          n607 = Increment(x=w885) -> (x+1=w883:u16)
                          n608 = Increment(x=w881) -> (x+1=w880:u16)
                          n609 = Replace Array Subset(array=w887, new element #1=w883, index #1=w884, new element #2=w880, index #2=w882) -> (w886:u16[])
                        }
                      }
                    }
                    frame False {
                      # "Solenoid_L"
                      n610 = call "myRIO_BRig_RT_dataMTrig_Solenoid_N__L.vi"() -> ("output_Solenoid_N__L"=w893:i32)  [unwired: 11 in]
                      n611 = Index Array(array=w896, index=w893) -> (element=w894:u16)
                      n612 = Increment(x=w894) -> (x+1=w892:u16)
                      n613 = Replace Array Subset(array=w896, new element=w892, index=w893) -> (w895:u16[])
                    }
                  }
                  n614 = local write "MTrig_Solenoid_trig__L"(FALSE) -> ()
                }
                frame 2 {
                  n615 = case shown="True" w899 {
                    tunnel: w901 -> [w906 w945]
                    tunnel: [w905 w944] -> w900
                    tunnel: w897 -> [w904 _]
                    frame True {
                      n616 = case shown="0, Default" w904 {
                        tunnel: [TRUE _ w938] -> w903
                        frame 0, Default {
                          # "Audio"
                        }
                        frame 1 {
                          # "LED"
                        }
                        frame 2 {
                          # "Audio or LED"
                          n617 = local read "Cue1Param_AudioLed_Probability_Switch"() -> (w940:u16)
                          n618 = call "myRIO__convert__Probability_to_TrueFalse.vi"("input_probability_u16"=w940) -> ("output_TF"=w939:bool)  [unwired: 10 in]
                          n619 = Not(x=w939) -> (.not. x?=w938:bool)
                        }
                      }
                      n620 = case shown="True" w903 {
                        tunnel: w906 -> [w918 w936]
                        tunnel: [w917 w935] -> w905
                        frame True {
                          n621 = call "myRIO_BRig_RT_dataMTrig_Solenoid_N__R.vi"() -> ("output_Solenoid_N__R"=w915:i32)  [unwired: 11 in]
                          n622 = call "myRIO_BRig_RT_dataMTrig_Audio_N__L.vi"() -> ("output_Audio_N__L"=w913:i32)  [unwired: 11 in]
                          n623 = call "myRIO_BRig_RT_dataMTrig_Audio_N__R.vi"() -> ("output_Audio_N__R"=w908:i32)  [unwired: 11 in]
                          n624 = local read "sp_RightSpout"() -> (w912:u16)
                          n625 = Index Array(array=w918, index #1=w915, index #2=w913, index #3=w908) -> (element #1=w916:u16, element #2=w911:u16, element #3=w910:u16)
                          n626 = case shown="2" w912 {
                            tunnel: w911 -> [w921 w924 w926]
                            tunnel: w910 -> [w919 w923 w928]
                            tunnel: [w920 w924 w925] -> w909
                            tunnel: [w919 w922 w927] -> w907
                            frame 0, Default {
                              n627 = Increment(x=w921) -> (x+1=w920:u16)
                            }
                            frame 1 {
                              n628 = Increment(x=w923) -> (x+1=w922:u16)
                            }
                            frame 2 {
                              n629 = Increment(x=w928) -> (x+1=w927:u16)
                              n630 = Increment(x=w926) -> (x+1=w925:u16)
                            }
                          }
                          n631 = Increment(x=w916) -> (x+1=w914:u16)
                          n632 = Replace Array Subset(array=w918, new element #1=w914, index #1=w915, new element #2=w909, index #2=w913, new element #3=w907, index #3=w908) -> (w917:u16[])
                        }
                        frame False {
                          n633 = call "myRIO_BRig_RT_dataMTrig_Solenoid_N__R.vi"() -> ("output_Solenoid_N__R"=w933:i32)  [unwired: 11 in]
                          n634 = call "myRIO_BRig_RT_dataMTrig_CueLed_N.vi"() -> ("output_CueLed_N"=w931:i32)  [unwired: 11 in]
                          n635 = Index Array(array=w936, index #1=w933, index #2=w931) -> (element #1=w934:u16, element #2=w930:u16)
                          n636 = Increment(x=w934) -> (x+1=w932:u16)
                          n637 = Increment(x=w930) -> (x+1=w929:u16)
                          n638 = Replace Array Subset(array=w936, new element #1=w932, index #1=w933, new element #2=w929, index #2=w931) -> (w935:u16[])
                        }
                      }
                    }
                    frame False {
                      # "Solenoid_R"
                      n639 = call "myRIO_BRig_RT_dataMTrig_Solenoid_N__R.vi"() -> ("output_Solenoid_N__R"=w942:i32)  [unwired: 11 in]
                      n640 = Index Array(array=w945, index=w942) -> (element=w943:u16)
                      n641 = Increment(x=w943) -> (x+1=w941:u16)
                      n642 = Replace Array Subset(array=w945, new element=w941, index=w942) -> (w944:u16[])
                    }
                  }
                  n643 = local write "MTrig_Solenoid_trig__R"(FALSE) -> ()
                }
                frame 3 {
                  w946 = FALSE
                  n644 = case shown="True" w949 {
                    tunnel: w951 -> [w955 w992]
                    tunnel: [w954 w991] -> w950
                    tunnel: w947 -> [w953 _]
                    frame True {
                      n645 = case shown="2" w953 {
                        tunnel: [TRUE _ w982] -> w952
                        frame 0, Default {
                          # "Audio"
                        }
                        frame 1 {
                          # "LED"
                        }
                        frame 2 {
                          # "Audio or LED"
                          n646 = local read "Cue1Param_AudioLed_Probability_Switch"() -> (w984:u16)
                          n647 = call "myRIO__convert__Probability_to_TrueFalse.vi"("input_probability_u16"=w984) -> ("output_TF"=w983:bool)  [unwired: 10 in]
                          n648 = Not(x=w983) -> (.not. x?=w982:bool)
                        }
                      }
                      n649 = case shown="True" w952 {
                        tunnel: w955 -> [w969 w980]
                        tunnel: [w968 w979] -> w954
                        frame True {
                          n650 = call "myRIO_BRig_RT_dataMTrig_Solenoid_N__L.vi"() -> ("output_Solenoid_N__L"=w957:i32)  [unwired: 11 in]
                          n651 = call "myRIO_BRig_RT_dataMTrig_Solenoid_N__R.vi"() -> ("output_Solenoid_N__R"=w966:i32)  [unwired: 11 in]
                          n652 = call "myRIO_BRig_RT_dataMTrig_Audio_N__L.vi"() -> ("output_Audio_N__L"=w964:i32)  [unwired: 11 in]
                          n653 = call "myRIO_BRig_RT_dataMTrig_Audio_N__R.vi"() -> ("output_Audio_N__R"=w960:i32)  [unwired: 11 in]
                          n654 = Index Array(array=w969, index #1=w957, index #2=w966, index #3=w964, index #4=w960) -> (element #1=w958:u16, element #2=w967:u16, element #3=w963:u16, element #4=w962:u16)
                          n655 = Increment(x=w958) -> (x+1=w956:u16)
                          n656 = Increment(x=w967) -> (x+1=w965:u16)
                          n657 = Increment(x=w962) -> (x+1=w959:u16)
                          n658 = Increment(x=w963) -> (x+1=w961:u16)
                          n659 = Replace Array Subset(array=w969, new element #1=w956, index #1=w957, new element #2=w965, index #2=w966, new element #3=w961, index #3=w964, new element #4=w959, index #4=w960) -> (w968:u16[])
                        }
                        frame False {
                          n660 = call "myRIO_BRig_RT_dataMTrig_Solenoid_N__L.vi"() -> ("output_Solenoid_N__L"=w970:i32)  [unwired: 11 in]
                          n661 = call "myRIO_BRig_RT_dataMTrig_Solenoid_N__R.vi"() -> ("output_Solenoid_N__R"=w977:i32)  [unwired: 11 in]
                          n662 = call "myRIO_BRig_RT_dataMTrig_CueLed_N.vi"() -> ("output_CueLed_N"=w975:i32)  [unwired: 11 in]
                          n663 = Index Array(array=w980, index #1=w970, index #2=w977, index #3=w975) -> (element #1=w972:u16, element #2=w978:u16, element #3=w974:u16)
                          n664 = Increment(x=w972) -> (x+1=w971:u16)
                          n665 = Increment(x=w978) -> (x+1=w976:u16)
                          n666 = Increment(x=w974) -> (x+1=w973:u16)
                          n667 = Replace Array Subset(array=w980, new element #1=w971, index #1=w970, new element #2=w976, index #2=w977, new element #3=w973, index #3=w975) -> (w979:u16[])
                        }
                      }
                    }
                    frame False {
                      n668 = call "myRIO_BRig_RT_dataMTrig_Solenoid_N__L.vi"() -> ("output_Solenoid_N__L"=w988:i32)  [unwired: 11 in]
                      n669 = call "myRIO_BRig_RT_dataMTrig_Solenoid_N__R.vi"() -> ("output_Solenoid_N__R"=w987:i32)  [unwired: 11 in]
                      n670 = Index Array(array=w992, index #1=w988, index #2=w987) -> (element #1=w990:u16, element #2=w986:u16)
                      n671 = Increment(x=w986) -> (x+1=w985:u16)
                      n672 = Increment(x=w990) -> (x+1=w989:u16)
                      n673 = Replace Array Subset(array=w992, new element #1=w989, index #1=w988, new element #2=w985, index #2=w987) -> (w991:u16[])
                    }
                  }
                  n674 = local write "MTrig_Solenoid_trig__L"(w946) -> ()
                  n675 = local write "MTrig_Solenoid_trig__R"(w946) -> ()
                }
              }
              n676 = local read "get_countPerMS"() -> (w826:bool)
              n677 = Select(t=myRIO_BRig_RT__Case_NonExp_stateList."Get_FPGA_count_per_ms" ("Enum"), s=w826, f=myRIO_BRig_RT__Case_NonExp_stateList."Idle_6" ("Enum")) -> (s? t:f=w824:T1)
              n678 = Select(t=myRIO_BRig_RT__Case_NonExp_stateList."Cue_pre", s=w830, f=myRIO_BRig_RT__Case_NonExp_stateList."DispenseWater_pre" ("Enum")) -> (s? t:f=w828:T1)
              n679 = Select(t=w828, s=w832, f=w824) -> (s? t:f=w833:T1)
            }
            frame "Idle_6" {
              # "There are a number of tasks we need to perform\nwhile idling. To preserve our timing loop, we\nbreak up the IDLE state into smaller states"
              # "use dataMTrig as it is one of the last to transfer"
              n680 = call "myRIO_BRig_RT_comm_webdav_uploadReceived_check_v2,0.vi"("input_dataName"="dataMTrig") -> ("output_Iexist"=w997:bool)  [unwired: 9 in, 1 out]
              n681 = Select(t=myRIO_BRig_RT__Case_NonExp_stateList."UploadSettings_pre" ("Enum"), s=w997, f=myRIO_BRig_RT__Case_NonExp_stateList."Idle") -> (s? t:f=w995:T1)
            }
            frame "Cue_pre" {
              w1004 = u16 0 ("new element/subarray")
              # "Audio cue or LED cue?"
              # "Audio, LED, or \"Audio or LED\""
              # "Right Audio?"
              # "Left Audio?"
              # "Left or Right?"
              # "Cue Audio?\n(T=Audio, F=LED)"
              # "Ncycle"
              # "count"
              # "Audio_R"
              # "Ncycle"
              # "count"
              # "Audio_L"
              n682 = local read "Cue1Param_CueType_Switch"() -> (w1028:u16)
              n683 = case shown="2" w1028 {
                tunnel: [TRUE _ w1046] -> w1000
                frame 0, Default {
                  # "Audio"
                }
                frame 1 {
                  # "LED"
                }
                frame 2 {
                  # "Audio or LED"
                  n684 = local read "Cue1Param_AudioLed_Probability_Switch"() -> (w1048:u16)
                  n685 = call "myRIO__convert__Probability_to_TrueFalse.vi"("input_probability_u16"=w1048) -> ("output_TF"=w1047:bool)  [unwired: 10 in]
                  n686 = Not(x=w1047) -> (.not. x?=w1046:bool)
                }
              }
              n687 = call "myRIO_BRig_RT_dataMTrig_Solenoid_N__L.vi"() -> ("output_Solenoid_N__L"=w1038:i32)  [unwired: 11 in]
              n688 = call "myRIO_BRig_RT_dataMTrig_Solenoid_N__R.vi"() -> ("output_Solenoid_N__R"=w1037:i32)  [unwired: 11 in]
              n689 = Index Array(array=w1034, index #1=w1038, index #2=w1037) -> (element #1=w1036:u16, element #2=w1035:u16)
              n690 = Not Equal To 0?(x=w1036) -> (x != 0?=w1024:bool)
              n691 = Not Equal To 0?(x=w1035) -> (x != 0?=w1023:bool)
              n692 = Not(x=w1000) -> (.not. x?=w999:bool)
              n693 = And(x=w1000, y=w1024) -> (x .and. y?=w1018:bool)
              n694 = And(x=w1000, y=w1023) -> (x .and. y?=w1016:bool)
              n695 = Select(t=myRIO_BRig_RT__Case_NonExp_stateList."Cue", s=w1000, f=myRIO_BRig_RT__Case_NonExp_stateList."Cue") -> (s? t:f=w1026:T1)
              n696 = local read "sp_RightSpout"() -> (w1017:u16)
              n697 = local read "sp_LeftSpout"() -> (w1019:u16)
              n698 = Boolean To (0,1)(Boolean=w999) -> (0, 1=w1002:i16)
              n699 = To Unsigned Word Integer(number=w1002) -> (unsigned 16bit integer=w1001:u16)
              n700 = case shown="0, Default" w1019 {
                tunnel: [w1042 _ w1044] -> w1015
                tunnel: [_ w1043 w1044] -> w1013
                tunnel: w1018 -> [w1042 w1043 w1044]
                frame 0, Default {
                }
                frame 1 {
                }
                frame 2 {
                }
              }
              n701 = case shown="0, Default" w1017 {
                tunnel: [w1039 _ w1041] -> w1014
                tunnel: [_ w1040 w1041] -> w1012
                tunnel: w1016 -> [w1039 w1040 w1041]
                frame 0, Default {
                }
                frame 1 {
                }
                frame 2 {
                }
              }
              n702 = call "myRIO_BRig_RT_dataMTrig_Audio_c__L.vi"() -> ("output_Audio_c__L"=w1032:i32)  [unwired: 11 in]
              n703 = call "myRIO_BRig_RT_dataMTrig_Audio_N__L.vi"() -> ("output_Audio_N__L"=w1031:i32)  [unwired: 11 in]
              n704 = call "myRIO_BRig_RT_dataMTrig_Audio_c__R.vi"() -> ("output_Audio_c__R"=w1030:i32)  [unwired: 11 in]
              n705 = call "myRIO_BRig_RT_dataMTrig_Audio_N__R.vi"() -> ("output_Audio_N__R"=w1029:i32)  [unwired: 11 in]
              n706 = call "myRIO_BRig_RT_dataMTrig_CueLed_c.vi"() -> ("output_CueLed_c"=w1005:i32)  [unwired: 11 in]
              n707 = call "myRIO_BRig_RT_dataMTrig_CueLed_N.vi"() -> ("output_CueLed_N"=w1003:i32)  [unwired: 11 in]
              n708 = Or(x=w1015, y=w1014) -> (x .or. y?=w1011:bool)
              n709 = Boolean To (0,1)(Boolean=w1011) -> (0, 1=w1009:i16)
              n710 = To Unsigned Word Integer(number=w1009) -> (unsigned 16bit integer=w1008:u16)
              n711 = Or(x=w1013, y=w1012) -> (x .or. y?=w1010:bool)
              n712 = Boolean To (0,1)(Boolean=w1010) -> (0, 1=w1007:i16)
              n713 = To Unsigned Word Integer(number=w1007) -> (unsigned 16bit integer=w1006:u16)
              n714 = Replace Array Subset(array=w1034, new element #1=w1004, index #1=w1032, new element #2=w1008, index #2=w1031, new element #3=w1004, index #3=w1030, new element #4=w1006, index #4=w1029, new element #5=w1004, index #5=w1005, new element #6=w1001, index #6=w1003) -> (w1033:u16[])
              n715 = Initialize Array(u16 0 ("element"), 1 ("dimension size")) -> (w1022:u16[])
            }
            frame "Cue" {
              # "warmupType\n0 = Cue with reward (not possible to be in this state with value==0)\n1 = Cue then reward\n2 = Cue then reward (no lick)"
              # "Audio cue"
              # "lick did not occur or warmupType==1"
              # "lick occurred?"
              # "Ncycle"
              # "Audio_R"
              # "Ncycle"
              # "Audio_L"
              n716 = local read "warmupType"() -> (w1058:u8)
              n717 = Greater?(x=w1064, y=w1063) -> (0:w1067:bool)
              n718 = Greater?(x=w1066, y=w1065) -> (0:w1062:bool)
              n719 = Or(x=w1062, y=w1067) -> (x .or. y?=w1056:bool)
              n720 = Equal?(x=w1058, y=u8 1) -> (x = y?=w1052:bool)
              n721 = Not(x=w1056) -> (.not. x?=w1055:bool)
              n722 = call "myRIO_BRig_RT_dataMTrig_Audio_N__L.vi"() -> ("output_Audio_N__L"=w1069:i32)  [unwired: 11 in]
              n723 = call "myRIO_BRig_RT_dataMTrig_Audio_N__R.vi"() -> ("output_Audio_N__R"=w1068:i32)  [unwired: 11 in]
              n724 = call "myRIO_BRig_RT_dataMTrig_CueLed_N.vi"() -> ("output_CueLed_N"=w1049:i32)  [unwired: 11 in]
              n725 = Or(x=w1055, y=w1052) -> (x .or. y?=w1053:bool)
              n726 = case shown="True" w1053 {
                tunnel: w1069 -> [w1075 w1096]
                tunnel: w1068 -> [w1074 w1095]
                tunnel: w1061 -> [w1077 w1090]
                tunnel: [w1076 w1090] -> w1060
                tunnel: w1059 -> [_ w1088]
                tunnel: [myRIO_BRig_RT__Case_NonExp_stateList."Idle" ("t") w1087] -> w1054
                tunnel: w1052 -> [_ w1086]
                tunnel: w1051 -> [_ w1082]
                tunnel: w1050 -> [_ w1081]
                tunnel: w1049 -> [_ w1080]
                frame False {
                  w1070 = u16 0 ("new element/subarray")
                  # "lick occurred and warmupType==2"
                  n727 = call "myRIO_BRig_RT_dataMTrig_Solenoid_N__R.vi"() -> ("output_Solenoid_N__R"=w1071:i32)  [unwired: 11 in]
                  n728 = call "myRIO_BRig_RT_dataMTrig_Solenoid_N__L.vi"() -> ("output_Solenoid_N__L"=w1072:i32)  [unwired: 11 in]
                  n729 = Replace Array Subset(array=w1077, new element #1=w1070, index #1=w1075, new element #2=w1070, index #2=w1074, new element #3=w1070, index #3=w1072, new element #4=w1070, index #4=w1071) -> (w1076:u16[])
                }
                frame True {
                  n730 = Not(x=w1086) -> (.not. x?=w1085:bool)
                  n731 = Index Array(array=w1090, index #1=w1096, index #2=w1095, index #3=w1080) -> (element #1=w1094:u16, element #2=w1093:u16, element #3=w1079:u16)
                  n732 = Equal To 0?(x=w1094) -> (x = 0?=w1092:bool)
                  n733 = Equal To 0?(x=w1093) -> (x = 0?=w1091:bool)
                  n734 = Equal To 0?(x=w1079) -> (x = 0?=w1078:bool)
                  n735 = Compound Arithmetic op=AND(w1092, w1091, w1078) -> (w1084:bool)
                  n736 = And(x=w1084, y=w1085) -> (x .and. y?=w1083:bool)
                  n737 = case shown="True" w1083 {
                    tunnel: w1082 -> [_ w1104]
                    tunnel: w1081 -> [_ w1099]
                    frame False {
                    }
                    frame True {
                      n738 = local read "count_warmup_R"() -> (w1097:u16)
                      n739 = local read "count_warmup_L"() -> (w1102:u16)
                      n740 = Increment(x=w1097) -> (x+1=w1100:u16)
                      n741 = Increment(x=w1102) -> (x+1=w1103:u16)
                      n742 = Select(t=w1100, s=w1099, f=w1097) -> (s? t:f=w1098:u16)
                      n743 = Select(t=w1103, s=w1104, f=w1102) -> (s? t:f=w1101:u16)
                      n744 = local write "count_warmup_R"(w1098) -> ()
                      n745 = local write "count_warmup_L"(w1101) -> ()
                    }
                  }
                  n746 = Select(t=myRIO_BRig_RT__Case_NonExp_stateList."DispenseWater_pre", s=w1084, f=w1088) -> (s? t:f=w1087:T1)
                }
              }
            }
            frame "Cue_LED" {
              # "LED Cue"
              # "lick did not occur or warmupType==1"
              # "lick occurred?"
              n747 = local read "warmupType"() -> (w1117:u8)
              n748 = Greater?(x=w1123, y=w1122) -> (0:w1126:bool)
              n749 = Greater?(x=w1125, y=w1124) -> (0:w1121:bool)
              n750 = Or(x=w1121, y=w1126) -> (x .or. y?=w1115:bool)
              n751 = Equal?(x=w1117, y=u8 1) -> (x = y?=w1111:bool)
              n752 = Not(x=w1115) -> (.not. x?=w1114:bool)
              n753 = Or(x=w1114, y=w1111) -> (x .or. y?=w1112:bool)
              n754 = case shown="True" w1112 {
                tunnel: w1120 -> [w1133 w1153]
                tunnel: [w1132 w1153] -> w1119
                tunnel: w1118 -> [_ w1139]
                tunnel: [myRIO_BRig_RT__Case_NonExp_stateList."Idle" ("t") w1152] -> w1113
                tunnel: w1111 -> [_ w1138]
                tunnel: w1110 -> [_ w1150]
                tunnel: w1109 -> [_ w1149]
                tunnel: w1108 -> [w1127 w1148]
                tunnel: [w1127 w1141] -> w1107
                tunnel: w1106 -> [_ w1136]
                tunnel: w1105 -> [_ w1135]
                frame False {
                  w1128 = u16 0 ("new element/subarray")
                  # "lick occurred and warmupType==2"
                  n755 = call "myRIO_BRig_RT_dataMTrig_Solenoid_N__R.vi"() -> ("output_Solenoid_N__R"=w1129:i32)  [unwired: 11 in]
                  n756 = call "myRIO_BRig_RT_dataMTrig_Solenoid_N__L.vi"() -> ("output_Solenoid_N__L"=w1130:i32)  [unwired: 11 in]
                  n757 = Replace Array Subset(array=w1133, new element #1=w1128, new element #2=w1128, index #2=w1130, new element #3=w1128, index #3=w1129) -> (w1132:u16[])  [unwired: 1 in]
                }
                frame True {
                  w1146 = 0 ("index")
                  n758 = local read "Tcycle_Cue_LED_min"() -> (w1142:u16)
                  n759 = Index Array(array=w1148, index=w1146) -> (element=w1147:u16)
                  n760 = Increment(x=w1147) -> (x+1=w1145:u16)
                  n761 = Multiply(x=w1145, y=u16 5) -> (x*y=w1143:u16)
                  n762 = Replace Array Subset(array=w1148, new element=w1145, index=w1146) -> (w1141:u16[])
                  n763 = Less?(x=w1143, y=w1142) -> (x < y?=w1137:bool)
                  n764 = Not Or(1:w1138, 2:w1137) -> (0:w1151:bool)
                  n765 = case shown="True" w1151 {
                    tunnel: w1150 -> [_ w1161]
                    tunnel: w1149 -> [_ w1156]
                    frame False {
                    }
                    frame True {
                      n766 = local read "count_warmup_R"() -> (w1154:u16)
                      n767 = local read "count_warmup_L"() -> (w1159:u16)
                      n768 = Increment(x=w1154) -> (x+1=w1157:u16)
                      n769 = Increment(x=w1159) -> (x+1=w1160:u16)
                      n770 = Select(t=w1157, s=w1156, f=w1154) -> (s? t:f=w1155:u16)
                      n771 = Select(t=w1160, s=w1161, f=w1159) -> (s? t:f=w1158:u16)
                      n772 = local write "count_warmup_R"(w1155) -> ()
                      n773 = local write "count_warmup_L"(w1158) -> ()
                    }
                  }
                  n774 = Select(t=w1139, s=w1137, f=myRIO_BRig_RT__Case_NonExp_stateList."DispenseWater_pre" ("t")) -> (s? t:f=w1152:T1)
                  n775 = xnode "Read/Write Control"("FPGA VI Reference In"=w1136, "error in"=w1135, "CueLed_Event"=w1137) -> ("error out"=w1134:errorcluster)  [unwired: 1 out]
                  n776 = local write "error out"(w1134) -> ()
                }
              }
            }
            frame "RewardCalibration_pre" {
              (unwired) FALSE
              w1162 = FALSE
              w1173 = u8 0
              w1189 = u8 0
              # "Are we starting a RewardCalibration?\nOr are we stopping a RewardCalibration?\nOr is a RewardCalibration over?"
              # "RewCalib\nOnOff"
              # "N"
              # "Solenoid R"
              # "RewCalib\nOnOff"
              # "N"
              # "Solenoid L"
              n777 = local read "RewCalib_Trig_L"() -> (w1196:bool)
              n778 = local read "RewCalib_Trig_R"() -> (w1165:bool)
              n779 = call "myRIO_BRig_RT_dataMTrig_Solenoid_N__R.vi"() -> ("output_Solenoid_N__R"=w1167:i32)  [unwired: 11 in]
              n780 = call "myRIO_BRig_RT_dataMTrig_Solenoid_RewCalib_OnOff__R.vi"() -> ("output_Solenoid_RewCalib_OnOff__R"=w1164:i32)  [unwired: 11 in]
              n781 = call "myRIO_BRig_RT_dataMTrig_Solenoid_N__L.vi"() -> ("output_Solenoid_N__L"=w1182:i32)  [unwired: 11 in]
              n782 = call "myRIO_BRig_RT_dataMTrig_Solenoid_RewCalib_OnOff__L.vi"() -> ("output_Solenoid_RewCalib_OnOff__L"=w1183:i32)  [unwired: 11 in]
              n783 = Index Array(array=w1166, index #1=w1167, index #2=w1164) -> (element #1=w1177:u16, element #2=w1172:u16)
              n784 = Index Array(array=w1166, index #1=w1182, index #2=w1183) -> (element #1=w1193:u16, element #2=w1188:u16)
              n785 = Equal To 0?(x=w1177) -> (x = 0?=w1178:bool)
              n786 = Not Equal To 0?(x=w1172) -> (x != 0?=w1175:bool)
              n787 = Equal To 0?(x=w1193) -> (x = 0?=w1194:bool)
              n788 = Not Equal To 0?(x=w1188) -> (x != 0?=w1191:bool)
              n789 = local write "MTrig_Solenoid_trig__L"(w1162) -> ()
              n790 = local write "MTrig_Solenoid_trig__R"(w1162) -> ()
              n791 = Select(t=u8 1, s=w1165, f=w1173) -> (s? t:f=w1169:u8)
              n792 = Select(t=u8 1, s=w1196, f=w1189) -> (s? t:f=w1185:u8)
              n793 = Select(t=u8 2, s=w1178, f=w1173) -> (s? t:f=w1170:u8)
              n794 = Select(t=u8 4, s=w1175, f=w1173) -> (s? t:f=w1171:u8)
              n795 = Select(t=u8 2, s=w1194, f=w1189) -> (s? t:f=w1186:u8)
              n796 = Select(t=u8 4, s=w1191, f=w1189) -> (s? t:f=w1187:u8)
              n797 = Compound Arithmetic op=ADD(w1169, w1170, w1171) -> (w1168:u8)
              n798 = Compound Arithmetic op=ADD(w1185, w1186, w1187) -> (w1184:u8)
              n799 = case shown="7" w1184 {
                tunnel: w1166 -> [w1226 w1231 w1233 w1238 w1243 w1245 w1248 w1253]
                tunnel: [w1226 w1232 w1233 w1239 w1244 w1245 w1249 w1254] -> w1181
                tunnel: w1183 -> [_ w1229 _ w1236 w1241 _ w1247 w1252]
                tunnel: w1182 -> [_ w1230 _ w1237 w1242 _ _ _]
                frame 0, Default {
                }
                frame 1 {
                  n800 = Replace Array Subset(array=w1231, new element #1=u16 100 ("new element/subarray"), index #1=w1230, new element #2=u16 1 ("new element/subarray"), index #2=w1229) -> (w1232:u16[])
                }
                frame 2 {
                }
                frame 3 {
                  n801 = Replace Array Subset(array=w1238, new element #1=u16 100 ("new element/subarray"), index #1=w1237, new element #2=u16 1 ("new element/subarray"), index #2=w1236) -> (w1239:u16[])
                }
                frame 4 {
                  w1240 = u16 0 ("new element/subarray")
                  n802 = Replace Array Subset(array=w1243, new element #1=w1240, index #1=w1242, new element #2=w1240, index #2=w1241) -> (w1244:u16[])
                }
                frame 5 {
                }
                frame 6 {
                  n803 = Replace Array Subset(array=w1248, new element=u16 0 ("new element/subarray"), index=w1247) -> (w1249:u16[])
                }
                frame 7 {
                  n804 = local write "RewCalib_Trig_L"(FALSE ("RewCalib_Trig_L")) -> ()
                  n805 = Replace Array Subset(array=w1253, new element=u16 0 ("new element/subarray"), index=w1252) -> (w1254:u16[])
                }
              }
              n806 = case shown="7" w1168 {
                tunnel: w1181 -> [w1197 w1202 w1204 w1209 w1214 w1216 w1219 w1224]
                tunnel: [w1197 w1203 w1204 w1210 w1215 w1216 w1220 w1225] -> w1180
                tunnel: w1164 -> [_ w1200 _ w1207 w1212 _ w1218 w1223]
                tunnel: w1167 -> [_ w1201 _ w1208 w1213 _ _ _]
                frame 0, Default {
                }
                frame 1 {
                  n807 = Replace Array Subset(array=w1202, new element #1=u16 100 ("new element/subarray"), index #1=w1201, new element #2=u16 1 ("new element/subarray"), index #2=w1200) -> (w1203:u16[])
                }
                frame 2 {
                }
                frame 3 {
                  n808 = Replace Array Subset(array=w1209, new element #1=u16 100 ("new element/subarray"), index #1=w1208, new element #2=u16 1 ("new element/subarray"), index #2=w1207) -> (w1210:u16[])
                }
                frame 4 {
                  w1211 = u16 0 ("new element/subarray")
                  n809 = Replace Array Subset(array=w1214, new element #1=w1211, index #1=w1213, new element #2=w1211, index #2=w1212) -> (w1215:u16[])
                }
                frame 5 {
                }
                frame 6 {
                  n810 = Replace Array Subset(array=w1219, new element=u16 0 ("new element/subarray"), index=w1218) -> (w1220:u16[])
                }
                frame 7 {
                  n811 = local write "RewCalib_Trig_R"(FALSE ("RewCalib_Trig_L")) -> ()
                  n812 = Replace Array Subset(array=w1224, new element=u16 0 ("new element/subarray"), index=w1223) -> (w1225:u16[])
                }
              }
            }
            frame "DispenseWater_pre" {
              w1260 = u16 0 ("t")
              w1303 = u16 0 ("new element/subarray")
              # "just trust me on this one"
              # "RewCalib\nOnOff"
              # "RewCalib\nOnOff"
              # "nCycle"
              # "Solenoid__R"
              # "Tdelay"
              # "delay"
              # "nCycle"
              # "Solenoid__L"
              # "Tdelay"
              # "delay"
              # "Solenoid__R"
              # "count"
              # "Solenoid_Tcycle_R"
              # "Solenoid_Tcycle_L"
              # "Solenoid__L"
              # "count"
              n813 = call "myRIO_BRig_RT_dataMTrig_Solenoid_RewCalib_OnOff__L.vi"() -> ("output_Solenoid_RewCalib_OnOff__L"=w1267:i32)  [unwired: 11 in]
              n814 = call "myRIO_BRig_RT_dataMTrig_Solenoid_N__L.vi"() -> ("output_Solenoid_N__L"=w1258:i32)  [unwired: 11 in]
              n815 = call "myRIO_BRig_RT_dataMTrig_Solenoid_delay__L.vi"() -> ("output_Solenoid_delay__L"=w1301:i32)  [unwired: 11 in]
              n816 = call "myRIO_BRig_RT_dataMTrig_Solenoid_Tdelay__L.vi"() -> ("output_Solenoid_Tdelay__L"=w1300:i32)  [unwired: 11 in]
              n817 = call "myRIO_BRig_RT_dataMTrig_Solenoid_N__R.vi"() -> ("output_Solenoid_N__R"=w1256:i32)  [unwired: 11 in]
              n818 = call "myRIO_BRig_RT_dataMTrig_Solenoid_delay__R.vi"() -> ("output_Solenoid_delay__R"=w1290:i32)  [unwired: 11 in]
              n819 = call "myRIO_BRig_RT_dataMTrig_Solenoid_Tdelay__R.vi"() -> ("output_Solenoid_Tdelay__R"=w1289:i32)  [unwired: 11 in]
              n820 = call "myRIO_BRig_RT_dataMTrig_Solenoid_RewCalib_OnOff__R.vi"() -> ("output_Solenoid_RewCalib_OnOff__R"=w1263:i32)  [unwired: 11 in]
              n821 = Index Array(array=w1302, index #1=w1258, index #2=w1301, index #3=w1300, index #4=w1256, index #5=w1290, index #6=w1289, index #7=w1267, index #8=w1263) -> (element #1=w1259:u16, element #2=w1299:u16, element #3=w1294:u16, element #4=w1262:u16, element #5=w1284:u16, element #6=w1283:u16, element #7=w1268:u16, element #8=w1265:u16)
              n822 = Equal To 0?(x=w1299) -> (x = 0?=w1298:bool)
              n823 = Equal To 0?(x=w1284) -> (x = 0?=w1288:bool)
              n824 = local read "RewCalib_Trig_L"() -> (w1279:bool)
              n825 = local read "RewCalib_Trig_R"() -> (w1274:bool)
              n826 = Not Equal To 0?(x=w1259) -> (x != 0?=w1297:bool)
              n827 = Not Equal To 0?(x=w1262) -> (x != 0?=w1287:bool)
              n828 = local read "MTrig_Solenoid_Tcycle__L"() -> (w1296:u16)
              n829 = local read "MTrig_Solenoid_Tcycle__R"() -> (w1282:u16)
              n830 = Not Equal To 0?(x=w1268) -> (x != 0?=w1278:bool)
              n831 = Not Equal To 0?(x=w1265) -> (x != 0?=w1276:bool)
              n832 = Not(x=w1279) -> (.not. x?=w1277:bool)
              n833 = Not(x=w1274) -> (.not. x?=w1275:bool)
              n834 = And(x=w1278, y=w1277) -> (x .and. y?=w1273:bool)
              n835 = And(x=w1276, y=w1275) -> (x .and. y?=w1272:bool)
              n836 = call "myRIO_BRig_RT_dataMTrig_Solenoid_c__L.vi"() -> ("output_Solenoid_c__L"=w1305:i32)  [unwired: 11 in]
              n837 = call "myRIO_BRig_RT_dataMTrig_Solenoid_c__R.vi"() -> ("output_Solenoid_c__R"=w1304:i32)  [unwired: 11 in]
              n838 = Select(t=w1296, s=w1297, f=u16 0) -> (s? t:f=w1293:u16)
              n839 = Or(x=w1273, y=w1272) -> (x .or. y?=w1261:bool)
              n840 = Select(t=w1282, s=w1287, f=u16 0) -> (s? t:f=w1285:u16)
              n841 = Select(t=w1293, s=w1298, f=w1294) -> (s? t:f=w1291:u16)
              n842 = Select(t=w1285, s=w1288, f=w1283) -> (s? t:f=w1280:u16)
              n843 = call "myRIO_BRig_RT_dataMTrig_Solenoid_Tcycle__L.vi"() -> ("output_Solenoid_Tcycle__L"=w1292:i32)  [unwired: 11 in]
              n844 = call "myRIO_BRig_RT_dataMTrig_Solenoid_Tcycle__R.vi"() -> ("output_Solenoid_Tcycle__R"=w1281:i32)  [unwired: 11 in]
              n845 = Select(t=w1260, s=w1261, f=w1259) -> (s? t:f=w1257:u16)
              n846 = Select(t=w1260, s=w1261, f=w1262) -> (s? t:f=w1255:u16)
              n847 = Select(t=myRIO_BRig_RT__Case_NonExp_stateList."Idle" ("Enum"), s=w1261, f=myRIO_BRig_RT__Case_NonExp_stateList."DispenseWater" ("Enum")) -> (s? t:f=w1269:T1)
              n848 = Select(t=w1260, s=w1261, f=w1268) -> (s? t:f=w1266:u16)
              n849 = Select(t=w1260, s=w1261, f=w1265) -> (s? t:f=w1264:u16)
              n850 = Replace Array Subset(array=w1302, new element #1=w1303, index #1=w1305, new element #2=w1303, index #2=w1304, new element #3=w1291, index #3=w1292, new element #4=w1280, index #4=w1281, new element #5=w1266, index #5=w1267, new element #6=w1264, index #6=w1263, new element #7=w1257, index #7=w1258, new element #8=w1255, index #8=w1256) -> (w1306:u16[])
            }
            frame "DispenseWater" {
              # "D"
              # "C"
              # "B"
              # "A"
              # "(A) Add COUNT and INCREMENT\n(B) Is (A) smaller than Tcycle?\n(C) Are we dispensing water or in the delay phase?\n(D) If (A) is smaller than Tcycle   AND   if we are dispensing water\n      then send TRUE to solenoid"
              # "delay"
              # "Tcycle"
              # "Solenoid__R"
              # "count"
              # "delay"
              # "Tcycle"
              # "Solenoid__L"
              # "count"
              n851 = To Unsigned Word Integer(number=w1333) -> (unsigned 16bit integer=w1315:u16)
              n852 = call "myRIO_BRig_RT_dataMTrig_Solenoid_delay__R.vi"() -> ("output_Solenoid_delay__R"=w1319:i32)  [unwired: 11 in]
              n853 = call "myRIO_BRig_RT_dataMTrig_Solenoid_c__R.vi"() -> ("output_Solenoid_c__R"=w1318:i32)  [unwired: 11 in]
              n854 = call "myRIO_BRig_RT_dataMTrig_Solenoid_Tcycle__R.vi"() -> ("output_Solenoid_Tcycle__R"=w1320:i32)  [unwired: 11 in]
              n855 = call "myRIO_BRig_RT_dataMTrig_Solenoid_delay__L.vi"() -> ("output_Solenoid_delay__L"=w1335:i32)  [unwired: 11 in]
              n856 = call "myRIO_BRig_RT_dataMTrig_Solenoid_c__L.vi"() -> ("output_Solenoid_c__L"=w1327:i32)  [unwired: 11 in]
              n857 = call "myRIO_BRig_RT_dataMTrig_Solenoid_Tcycle__L.vi"() -> ("output_Solenoid_Tcycle__L"=w1336:i32)  [unwired: 11 in]
              n858 = Index Array(array=w1329, index #1=w1327, index #2=w1336, index #3=w1335, index #4=w1318, index #5=w1320, index #6=w1319) -> (element #1=w1334:u16, element #2=w1324:u16, element #3=w1332:u16, element #4=w1314:u16, element #5=w1311:u16, element #6=w1310:u16)
              n859 = Add(x=w1334, y=w1315) -> (x+y=w1325:u16)
              n860 = Add(x=w1314, y=w1315) -> (x+y=w1316:u16)
              n861 = Less?(x=w1325, y=w1324) -> (x < y?=w1308:bool)
              n862 = Equal To 0?(x=w1332) -> (x = 0?=w1331:bool)
              n863 = Less?(x=w1316, y=w1311) -> (x < y?=w1309:bool)
              n864 = Equal To 0?(x=w1310) -> (x = 0?=w1317:bool)
              n865 = And(x=w1308, y=w1331) -> (x .and. y?=w1330:bool)
              n866 = Or(x=w1308, y=w1309) -> (x .or. y?=w1307:bool)
              n867 = And(x=w1309, y=w1317) -> (x .and. y?=w1312:bool)
              n868 = Select(t=w1325, s=w1308, f=w1324) -> (s? t:f=w1326:u16)
              n869 = Select(t=w1316, s=w1309, f=w1311) -> (s? t:f=w1313:u16)
              n870 = Replace Array Subset(array=w1329, new element #1=w1326, index #1=w1327, new element #2=w1313, index #2=w1318) -> (w1328:u16[])
              n871 = Select(t=w1323, s=w1307, f=myRIO_BRig_RT__Case_NonExp_stateList."DispenseWater_post" ("Enum")) -> (s? t:f=w1321:T1)
            }
            frame "DispenseWater_post" {
              # "nCycle"
              # "delay"
              # "Solenoid__R"
              # "nCycle"
              # "delay"
              # "Solenoid__L"
              n872 = call "myRIO_BRig_RT_dataMTrig_Solenoid_N__L.vi"() -> ("output_Solenoid_N__L"=w1353:i32)  [unwired: 11 in]
              n873 = call "myRIO_BRig_RT_dataMTrig_Solenoid_delay__L.vi"() -> ("output_Solenoid_delay__L"=w1352:i32)  [unwired: 11 in]
              n874 = call "myRIO_BRig_RT_dataMTrig_Solenoid_N__R.vi"() -> ("output_Solenoid_N__R"=w1349:i32)  [unwired: 11 in]
              n875 = call "myRIO_BRig_RT_dataMTrig_Solenoid_delay__R.vi"() -> ("output_Solenoid_delay__R"=w1348:i32)  [unwired: 11 in]
              n876 = Index Array(array=w1355, index #1=w1353, index #2=w1352, index #3=w1349, index #4=w1348) -> (element #1=w1357:u16, element #2=w1356:u16, element #3=w1340:u16, element #4=w1342:u16)
              n877 = Not Equal To 0?(x=w1357) -> (x != 0?=w1358:bool)
              n878 = Not Equal To 0?(x=w1340) -> (x != 0?=w1341:bool)
              n879 = case shown="True" w1341 {
                selector: w1341 -> [_ w1362]
                tunnel: w1340 -> [w1360 w1368]
                tunnel: w1342 -> [_ w1369]
                tunnel: [w1360 w1366] -> w1339
                tunnel: [u16 0 w1365] -> w1338
                tunnel: [_ w1362] -> w1337
                frame False {
                }
                frame True {
                  n880 = Equal To 0?(x=w1369) -> (x = 0?=w1361:bool)
                  n881 = Decrement(x=w1368) -> (x-1=w1367:u16)
                  n882 = Select(t=w1367, s=w1361, f=w1368) -> (s? t:f=w1366:u16)
                  n883 = Select(t=u16 1, s=w1361, f=u16 0) -> (s? t:f=w1365:u16)
                }
              }
              n884 = case shown="True" w1358 {
                selector: w1358 -> [_ w1373]
                tunnel: w1357 -> [w1371 w1379]
                tunnel: w1356 -> [_ w1380]
                tunnel: [w1371 w1377] -> w1351
                tunnel: [u16 0 w1376] -> w1350
                tunnel: [_ w1373] -> w1347
                frame False {
                }
                frame True {
                  n885 = Equal To 0?(x=w1380) -> (x = 0?=w1372:bool)
                  n886 = Decrement(x=w1379) -> (x-1=w1378:u16)
                  n887 = Select(t=w1378, s=w1372, f=w1379) -> (s? t:f=w1377:u16)
                  n888 = Select(t=u16 1, s=w1372, f=u16 0) -> (s? t:f=w1376:u16)
                }
              }
              n889 = Or(x=w1347, y=w1337) -> (x .or. y?=w1346:bool)
              n890 = Replace Array Subset(array=w1355, new element #1=w1351, index #1=w1353, new element #2=w1350, index #2=w1352, new element #3=w1339, index #3=w1349, new element #4=w1338, index #4=w1348) -> (w1354:u16[])
              n891 = Select(t=myRIO_BRig_RT__Case_NonExp_stateList."DispenseWater_pre" ("Enum"), s=w1346, f=myRIO_BRig_RT__Case_NonExp_stateList."Idle" ("Enum")) -> (s? t:f=w1343:T1)
            }
            frame "TestConnection" {
              n892 = local read "Host Password"() -> (w1386:string)
              n893 = local read "Host UserName"() -> (w1387:string)
              n894 = call "myRIO_BRig_RT_comm_webdav_testConnect.vi"("input_password"=w1386, "input_username"=w1387) -> ("output_Iconnected"=w1384:bool)  [unwired: 9 in]
              n895 = Select(t="Connection accepted!" ("message"), s=w1384, f="Error!") -> (s? t:f=w1382:string)
              n896 = One Button Dialog(message=w1382) -> ()  [unwired: 1 in, 1 out]
            }
            frame "SendData" {
              n897 = local read "Data Set Prefix"() -> (w1389:string)
              n898 = local read "Host Password"() -> (w1390:string)
              n899 = local read "Host UserName"() -> (w1391:string)
              n900 = call "myRIO_BRig_RT_comm_webdav_sendData_all.vi"("Host Filename Prefix"=w1389, "Host Password"=w1390, "Host UserName"=w1391) -> ()  [unwired: 9 in]
            }
            frame "Get_FPGA_count_per_ms" {
              # "Used to automatically determine how many FPGA cycles in 1 ms"
              n901 = case shown="False" w1404 {
                selector: w1404 -> [w1406 _]
                tunnel: w1402 -> [_ w1419]
                tunnel: [w1410 w1419] -> w1401
                tunnel: w1400 -> [w1409 w1417]
                tunnel: w1399 -> [w1408 w1416]
                tunnel: [w1407 w1414] -> w1394
                tunnel: [w1406 w1413] -> w1398
                frame False {
                  n902 = Get Date/Time In Seconds() -> (seconds since 1Jan1904=w1411:timestamp)
                  n903 = xnode "Read/Write Control"("FPGA VI Reference In"=w1409, "error in"=w1408, "timeTrial_trig"=TRUE ("timeTrial")) -> ("error out"=w1407:errorcluster)  [unwired: 1 out]
                  n904 = To Double Precision Float(number=w1411) -> (double precision float=w1410:dbl)
                  n905 = local write "get_countPerMS"(w1406) -> ()
                }
                frame True {
                  w1415 = 1.0
                  n906 = Get Date/Time In Seconds() -> (seconds since 1Jan1904=w1420:timestamp)
                  n907 = To Double Precision Float(number=w1420) -> (double precision float=w1421:dbl)
                  n908 = Subtract(x=w1421, y=w1419) -> (x-y=w1418:dbl)
                  n909 = Less Or Equal?(x=w1415, y=w1418) -> (x <= y?=w1413:bool)
                  n910 = case shown="True" w1413 {
                    tunnel: w1417 -> [_ w1434]
                    tunnel: w1416 -> [w1422 w1433]
                    tunnel: w1415 -> [_ w1424]
                    tunnel: [w1422 w1423] -> w1414
                    frame False {
                    }
                    frame True {
                      n911 = xnode "Read/Write Control"("FPGA VI Reference In"=w1434, "error in"=w1433) -> ("FPGA VI Reference Out"=w1431:refnum<k20>, "error out"=w1430:errorcluster, "timeTrial_count"=w1425:u32)
                      n912 = Multiply(x=w1424, y=1000.0) -> (x*y=w1428:dbl)
                      n913 = To Double Precision Float(number=w1425) -> (double precision float=w1427:dbl)
                      n914 = Divide(x=w1427, y=w1428) -> (x/y=w1429:dbl)
                      n915 = local write "FPGA_count2ms"(w1429) -> ()
                      n916 = xnode "Read/Write Control"("FPGA VI Reference In"=w1431, "error in"=w1430, "timeTrial_trig"=FALSE ("timeTrial")) -> ("error out"=w1423:errorcluster)  [unwired: 1 out]
                    }
                  }
                }
              }
              n917 = Select(t=myRIO_BRig_RT__Case_NonExp_stateList."Idle" ("Enum"), s=w1398, f=w1396) -> (s? t:f=w1395:T1)
              n918 = local write "error out"(w1394) -> ()
            }
            frame "End" {
            }
          }
          n919 = local read "MTrig_Audio_trig__R"() -> (w91:bool)
          n920 = local read "MTrig_Audio_trig__L"() -> (w92:bool)
          n921 = local read "MTrig_Laser_trig"() -> (w90:bool)
          n922 = local read "MTrig_CueLed"() -> (w83:bool)
          n923 = Compound Arithmetic op=OR(w92, w91, w90, w83) -> (w89:bool)
          n924 = local read "START"() -> (w115:bool)
          n925 = local read "STOP_abort"() -> (w114:bool)
          n926 = case shown="True" w89 {
            frame False {
            }
            frame True {
              w131 = FALSE
              n927 = local write "MTrig_Audio_trig__R"(w131) -> ()
              n928 = local write "MTrig_Audio_trig__L"(w131) -> ()
              n929 = local write "MTrig_Laser_trig"(w131) -> ()
              n930 = local write "MTrig_CueLed"(w131) -> ()
            }
          }
          n931 = call "myRIO_BRig_RT_dataMTrig_main__NoExp.vi"("input_dataMTrig"=w118, "input_Audio_trig_L"=w92, "input_Audio_trig_R"=w91, "input_Laser_trig"=w90, "input_CueLed"=w83) -> ("output_dataMTrig"=w117:u16[], "output_Audio_L"=w109:bool, "output_Audio_R"=w110:bool, "output_Laser"=w88:bool, "output_CueLed"=w82:bool)  [unwired: 10 in]
          n932 = Or(x=w115, y=w114) -> (x .or. y?=w113:bool)
          n933 = Select(t=myRIO_BRig_RT__Case_NonExp_stateList."End" ("Enum"), s=w113, f=w112) -> (s? t:f=w111:T1)
          n934 = Not(x="MTrig_Laser_Switch") -> (.not. x?=w85:bool)
          n935 = And(x=w88, y=w85) -> (x .and. y?=w86:bool)
          n936 = And(x=w88, y="MTrig_Laser_Switch") -> (x .and. y?=w87:bool)
          n937 = xnode "Read/Write Control"("FPGA VI Reference In"=w98, "error in"=w97, "A1_SR"=w119, "A3_SL"=w120, "audioTrigger_L"=w109, "audioTrigger_R"=w110, "LC_Laser_l1"=w86, "LC_Laser_l2"=w87, "CueLed_Event"=w82) -> ("FPGA VI Reference Out"=w125:refnum<k20>, "error out"=w124:errorcluster)
          n938 = node-c288() -> ()  [unwired: 1 in, 1 out]
          "cState_NonExp" <- w123
        }
        n939 = node-c288(w70) -> ()  [unwired: 1 out]
        n940 = flat-sequence {
          tunnel: w63 -> [w81]
          tunnel: [w81] -> w62
          tunnel: w61 -> [w80]
          tunnel: [w80] -> w60
          frame #0 {
            w79 = FALSE
            n941 = local write "STOP_endBlock"(w79) -> ()
            n942 = local write "STOP_endTrial"(w79) -> ()
          }
        }
      }
      frame True {
        w1447 = u16 0
        w1464 = u16 0 ("idxDataBlock")
        w1466 = u16 100 ("new element/subarray")
        w1467 = u16 100 ("new element/subarray")
        w1487 = T6 refnum items=["Session NI_WebDAV"] ("output_hSession")
        w1496 = FALSE
        # "dummyState counter"
        # "audio__L\naudio__R"
        # "Audio params"
        # "nRewards"
        # "idxDataBlock"
        # "Solenoid_Tdelay_R"
        # "Solenoid_Tdelay_L"
        # "RewCalib_N__R"
        # "RewCalib_N__L"
        # "Save dataLick to file\nSend file to Host\nSave dataMTrig\nSend file to Host\nDisconnect"
        # "dataTrial"
        # "dataTrial"
        # "Solenoid_Tcycle_R"
        # "Solenoid_Tcycle_L"
        # "Laser_Tcycle"
        # "Audio_Tcycle_R"
        # "Audio_Tcycle_L"
        # "dataLick"
        # "dataLC"
        # "dataLC"
        # "dataBlock"
        # "dataBlock"
        # "dataMTrig"
        # "dataMTrig"
        # "dataExp"
        # "dataCurrent"
        # "dataExp"
        # "dataCurrent"
        # "spout"
        # "state"
        n943 = call "myRIO_BRig_RT_dataMTrig_Solenoid_Tcycle__L.vi"() -> ("output_Solenoid_Tcycle__L"=w1493:i32)  [unwired: 11 in]
        n944 = call "myRIO_BRig_RT_dataMTrig_Solenoid_Tcycle__R.vi"() -> ("output_Solenoid_Tcycle__R"=w1492:i32)  [unwired: 11 in]
        n945 = call "myRIO_BRig_RT_dataMTrig_Audio_Tcycle__L.vi"() -> ("output_Audio_Tcycle__L"=w1491:i32)  [unwired: 11 in]
        n946 = call "myRIO_BRig_RT_dataMTrig_Audio_Tcycle__R.vi"() -> ("output_Audio_Tcycle__R"=w1490:i32)  [unwired: 11 in]
        n947 = call "myRIO_BRig_RT_dataMTrig_Laser_Tcycle.vi"() -> ("output_Laser_Tcycle"=w1489:i32)  [unwired: 11 in]
        n948 = local read "Tcycle_Reward_min_L"() -> (w1468:u16)
        n949 = local read "Tcycle_Reward_min_R"() -> (w1469:u16)
        n950 = local read "MTrig_Solenoid_Tcycle__L"() -> (w1472:u16)
        n951 = local read "MTrig_Solenoid_Tcycle__R"() -> (w1471:u16)
        n952 = local read "MTrig_Laser_Tcycle"() -> (w1470:u16)
        n953 = call "myRIO_BRig_RT_dataMTrig_Solenoid_RewCalib_nCycle__L.vi"() -> ("output_Solenoid_RewCalib_nCycle__L"=w1475:i32)  [unwired: 11 in]
        n954 = call "myRIO_BRig_RT_dataMTrig_Solenoid_Tdelay__L.vi"() -> ("output_Solenoid_Tdelay__L"=w1477:i32)  [unwired: 11 in]
        n955 = call "myRIO_BRig_RT_dataMTrig_Solenoid_RewCalib_nCycle__R.vi"() -> ("output_Solenoid_RewCalib_nCycle__R"=w1476:i32)  [unwired: 11 in]
        n956 = call "myRIO_BRig_RT_dataMTrig_Solenoid_Tdelay__R.vi"() -> ("output_Solenoid_Tdelay__R"=w1478:i32)  [unwired: 11 in]
        n957 = case shown="False" w1457 {
          selector: w1457 -> [_ w1518]
          tunnel: w1456 -> [w1515 w1520]
          tunnel: [w1516 w1520] -> w1452
          tunnel: w1455 -> [_ w1519]
          tunnel: [w1517 w1519] -> w1453
          tunnel: [w1514 w1518] -> w1451
          frame False {
            n958 = call "myRIO__TCP_connect_forWriting.vi"("input_error"=w1515) -> ("output_error"=w1516:errorcluster, "output_connected"=w1514:bool, "output_hTCP"=w1517:refnum<k5>)  [unwired: 8 in]
          }
          frame True {
          }
        }
        n959 = call "myRIO_BRig_RT_dataLick_init.vi"() -> ("output_dataLick"=w1498:u16[][])  [unwired: 11 in]
        n960 = call "myRIO_BRig_RT_dataCurrent_init.vi"() -> ("output_dataCurrent"=w1505:u16[])  [unwired: 11 in]
        n961 = call "myRIO_BRig_RT_dataExp_init.vi"() -> ("output_dataExp"=w1504:u16[])  [unwired: 11 in]
        n962 = call "myRIO_BRig_RT_dataMTrig_init.vi"() -> ("output_dataMTrig"=w1495:u16[])  [unwired: 5 in]
        n963 = call "myRIO_BRig_RT_dataLC_init.vi"() -> ("output_dataLC"=w1502:u16[])  [unwired: 11 in]
        n964 = call "myRIO_BRig_RT_dataBlock_init.vi"() -> ("output_dataBlock"=w1503:u16[][])  [unwired: 11 in]
        n965 = call "myRIO_BRig_RT_dataTrial_init.vi"() -> ("output_dataTrial"=w1488:u16[][])  [unwired: 11 in]
        n966 = local write "I_connect_TCP"(w1451) -> ()
        n967 = Replace Array Subset(array=w1495, new element #1=w1467, index #1=w1475, new element #2=w1467, index #2=w1476, new element #3=w1466, index #3=w1477, new element #4=w1466, index #4=w1478, new element #5=w1472, index #5=w1493, new element #6=w1471, index #6=w1492, new element #7=w1468, index #7=w1491, new element #8=w1469, index #8=w1490, new element #9=w1470, index #9=w1489) -> (w1494:u16[])
        n968 = call "myRIO_BRig_RT_dataAnalog_init.vi"() -> ("output_dataAnalog"=w1462:u16[][])  [unwired: 11 in]
        n969 = call "myRIO_BRig_RT_TCP__start_exp.vi"("input_hTCP"=w1453, "input_I_connected_TCP"=w1451, "input_error"=w1452) -> ("output_hTCP"=w1450:refnum<k5>, "output_error"=w1449:errorcluster)  [unwired: 11 in]
        n970 = Get Date/Time In Seconds() -> (seconds since 1Jan1904=w1474:timestamp)
        n971 = call "myRIO_BRig_RT_arrTrig_init.vi"() -> ("output_arrTrig"=w1446:bool[])  [unwired: 11 in]
        n972 = To Double Precision Float(number=w1474) -> (double precision float=w1473:dbl)
        n973 = node-c288() -> (w1513:T3)  [unwired: 4 in]
        n974 = timed-loop {
          timing: w1513 -> [_]
          timing-out: [_] -> w1512
          shift-right: [w1647] -> _
          shift-left: myRIO_BRig_RT__Case_Exp_stateList."Start1" ("Enum") -> [w1571]
          shift-right: [w1605] -> _
          shift-left: enum16{"Left", "Right"}."Left" -> [w1687]
          tunnel: w1445 -> [w1685]
          tunnel: w1444 -> [w1577]
          shift-right: [w1680] -> _
          shift-left: w1510 -> [w1684]
          shift-right: [w1679] -> _
          shift-left: w1509 -> [w1683]
          tunnel: [w1663] -> w1507
          tunnel: [w1664] -> w1508
          shift-right: [w1665] -> w1479
          shift-left: w1505 -> [w1566]
          shift-right: [w1678] -> _
          shift-left: w1504 -> [w1638]
          shift-right: [w1659] -> w1483
          shift-left: w1494 -> [w1660]
          shift-right: [w1676] -> _
          shift-left: w1503 -> [w1677]
          shift-right: [w1674] -> _
          shift-left: w1502 -> [w1675]
          shift-right: [w1666] -> w1485
          shift-left: w1498 -> [w1667]
          shift-right: [w1636] -> _
          shift-left: w1496 -> [w1661]
          shift-right: [w1637] -> _
          shift-left: w1496 -> [w1662]
          shift-right: [w1645] -> _
          shift-left: w1488 -> [w1646]
          shift-right: [w1644] -> w1481
          shift-left: w1487 -> [w1642]
          shift-right: [w1643] -> w1482
          shift-left: FALSE ("output_Iconnected") -> [w1641]
          tunnel: "Data Set Prefix" -> [w1640]
          tunnel: [w1640] -> w1480
          tunnel: w1473 -> [w1639]
          shift-right: [w1634] -> _
          shift-left: 0 ("idxDataBlock") -> [w1635]
          shift-right: [w1631] -> _
          shift-left: w1464 -> [w1633]
          shift-right: [w1630] -> _
          shift-left: w1464 -> [w1632]
          shift-right: [w1624] -> w1460
          shift-left: 0 -> [w1610]
          shift-right: [w1606] -> _
          shift-left: w1447 -> [w1619]
          shift-right: [w1607] -> _
          shift-left: w1447 -> [w1616]
          shift-right: [w1615] -> _
          shift-left: w1447 -> [w1622]
          shift-right: [w1625] -> w1461
          shift-left: w1462 -> [w1626]
          tunnel: w1450 -> [w1614]
          tunnel: [w1613] -> w1459
          tunnel: w1451 -> [w1611]
          tunnel: [w1611] -> w1458
          tunnel: w1449 -> [w1612]
          tunnel: [w1574] -> w1454
          shift-right: [w1603] -> _
          shift-left: u16 0 -> [w1604]
          shift-right: [w1601] -> _
          shift-left: w1447 -> [w1602]
          shift-right: [w1598] -> _
          shift-left: w1446 -> [w1599]
          shift-right: [w1569] -> _
          shift-left: FALSE -> [w1572]
          stop <- w1673 stop-if-true
          # "arrTrig"
          # "arrTrig"
          # "LC_Laser_l2"
          # "LC_Event_l2"
          # "LC_Laser_l1"
          # "LC_Event_l1"
          # "CueLed"
          # "LC_Laser_l2"
          # "LC_Event_l2"
          # "LC_Laser_l1"
          # "LC_Event_l1"
          # "solenoid__R"
          # "solenoid__L"
          # "spout"
          # "iState"
          # "dataAnalog"
          # "index"
          # "iEvent"
          # "iBlock"
          # "iTrial"
          # "Laser"
          # "Audio R"
          # "Audio L"
          # "Solenoid R"
          # "Solenoid L"
          # "manual triggering"
          # "dataTrial"
          # "dataBlock"
          # "nRewards"
          # "dataExp"
          # "dataCurrent"
          # "audio__L\naudio__R"
          # "time stamp"
          # "nRewards"
          # "idxDataBlock"
          # "idxDataBlock"
          # "audio__L\naudio__R"
          # "dataLC"
          # "solenoid__R"
          # "solenoid__L"
          # "Did a lick occur?"
          # "Update lick counter"
          # "spout"
          # "spout"
          # "state"
          # "state"
          n975 = node-c288() -> ()  [unwired: 1 in, 1 out]
          n976 = flat-sequence {
            tunnel: w1577 -> [w1688]
            tunnel: [w1688] -> _
            tunnel: [w1689] -> w1573
            tunnel: [w1688] -> w1576
            frame #0 {
              n977 = Get Date/Time In Seconds() -> (seconds since 1Jan1904=w1689:timestamp)
            }
          }
          n978 = xnode "Read/Write Control"("FPGA VI Reference In"=w1685, "error in"=w1576) -> ("FPGA VI Reference Out"=w1629:refnum<k20>, "error out"=w1628:errorcluster, "A2_LickL"=w1680:u32, "A4_LickR"=w1679:u32)
          "A2" <- w1680
          "A4" <- w1679
          n979 = Greater?(x=w1680, y=w1684) -> (0:w1682:bool)
          n980 = Greater?(x=w1679, y=w1683) -> (0:w1681:bool)
          n981 = call "myRIO_BRig_RT_dataCurrent_IallReward_L.vi"() -> ("output_IallReward_L"=w1567:i32)  [unwired: 11 in]
          n982 = call "myRIO_BRig_RT_dataCurrent_IallReward_R.vi"() -> ("output_IallReward_R"=w1568:i32)  [unwired: 11 in]
          n983 = Or(x=w1682, y=w1681) -> (x .or. y?=w1686:bool)
          n984 = local read "MTrig_Solenoid_trig__L"() -> (w1657:bool)
          n985 = local read "MTrig_Solenoid_trig__R"() -> (w1656:bool)
          n986 = local read "MTrig_Audio_trig__L"() -> (w1655:bool)
          n987 = local read "MTrig_Audio_trig__R"() -> (w1654:bool)
          n988 = local read "MTrig_Laser_trig"() -> (w1653:bool)
          n989 = Index Array(array=w1566, index #1=w1567, index #2=w1568) -> (element #1=w1564:u16, element #2=w1565:u16)
          n990 = Not Equal To 0?(x=w1564) -> (x != 0?=→"allReward_L":bool)
          n991 = Not Equal To 0?(x=w1565) -> (x != 0?=→"allReward_R":bool)
          n992 = case shown="\"saveSettings2\"" w1571 {
            selector: w1571 -> [_ _ _ _ _ _ _ _ _ _ _ _ _ _ _ _ _ _ _ _ _ _ _ _ _ w2653 _ w2696 _ _ _ _ _ w2793 _ w2853 _ _ _ _ _ w2956 _ w3007 _ w3063 _ w3103 _ _ w3161 _ _ _ _ _ w3308 _ _ _ _ _ _ _ _ _ _ _ _ w3541 w3570]
            tunnel: [myRIO_BRig_RT__Case_Exp_stateList."Start2" ("Enum") myRIO_BRig_RT__Case_Exp_stateList."Start3" ("Enum") myRIO_BRig_RT__Case_Exp_stateList."saveSettings1" ("Enum") myRIO_BRig_RT__Case_Exp_stateList."saveSettings2" ("Enum") myRIO_BRig_RT__Case_Exp_stateList."saveSettings3" ("Enum") myRIO_BRig_RT__Case_Exp_stateList."saveSettings4" ("Enum") myRIO_BRig_RT__Case_Exp_stateList."saveSettings_LC_ENL_l1" ("Enum") myRIO_BRig_RT__Case_Exp_stateList."saveSettings_LC_ENL_l2" ("Enum") myRIO_BRig_RT__Case_Exp_stateList."saveSettings_LC_Cue_l1" ("Enum") myRIO_BRig_RT__Case_Exp_stateList."saveSettings_LC_Cue_l2" ("Enum") myRIO_BRig_RT__Case_Exp_stateList."saveSettings6_LC_l1_Other" ("Enum") myRIO_BRig_RT__Case_Exp_stateList."SaveSettings6_LC_l2_Other" ("Enum") myRIO_BRig_RT__Case_Exp_stateList."setSettings_Audio" ("Enum") myRIO_BRig_RT__Case_Exp_stateList."setSettings_Laser" ("Enum") myRIO_BRig_RT__Case_Exp_stateList."commConnect" ("Enum") w2410 myRIO_BRig_RT__Case_Exp_stateList."initTrial" ("Enum") w2464 myRIO_BRig_RT__Case_Exp_stateList."initTrial3" ("Enum") myRIO_BRig_RT__Case_Exp_stateList."initTrial_LC_ENL1" ("Enum") myRIO_BRig_RT__Case_Exp_stateList."ENL1_pre" ("Enum") myRIO_BRig_RT__Case_Exp_stateList."initTrial_LC_Cue1" ("Enum") myRIO_BRig_RT__Case_Exp_stateList."initTrial_LC_Sel" ("Enum") myRIO_BRig_RT__Case_Exp_stateList."initTrial4" ("Enum") w2628 w2650 myRIO_BRig_RT__Case_Exp_stateList."ENL1Penalty" ("Enum") w2697 myRIO_BRig_RT__Case_Exp_stateList."endExp" ("Enum") myRIO_BRig_RT__Case_Exp_stateList."endExp" ("Enum") myRIO_BRig_RT__Case_Exp_stateList."endExp" ("Enum") myRIO_BRig_RT__Case_Exp_stateList."endExp" ("Enum") w2770 w2787 myRIO_BRig_RT__Case_Exp_stateList."Cue1Penalty" ("Enum") w2851 myRIO_BRig_RT__Case_Exp_stateList."endExp" ("Enum") myRIO_BRig_RT__Case_Exp_stateList."endExp" ("Enum") myRIO_BRig_RT__Case_Exp_stateList."endExp" ("Enum") myRIO_BRig_RT__Case_Exp_stateList."endExp" ("Enum") w2929 w2955 myRIO_BRig_RT__Case_Exp_stateList."SelectReward" ("Enum") w3008 myRIO_BRig_RT__Case_Exp_stateList."SelectRewardPost" ("Enum") w3064 myRIO_BRig_RT__Case_Exp_stateList."SelectWrong" ("Enum") w3099 myRIO_BRig_RT__Case_Exp_stateList."endTrial1" ("Enum") myRIO_BRig_RT__Case_Exp_stateList."SelectTimeout" ("Enum") w3163 myRIO_BRig_RT__Case_Exp_stateList."endTrial1" ("Enum") myRIO_BRig_RT__Case_Exp_stateList."endTrial2" ("Enum") myRIO_BRig_RT__Case_Exp_stateList."endTrial3" ("Enum") w3233 w3291 w3308 myRIO_BRig_RT__Case_Exp_stateList."initBlock" ("Enum") w3331 myRIO_BRig_RT__Case_Exp_stateList."commUpload_dataExp" ("Enum") myRIO_BRig_RT__Case_Exp_stateList."endBlock" ("Enum") myRIO_BRig_RT__Case_Exp_stateList."commUpload_dataLC" ("Enum") myRIO_BRig_RT__Case_Exp_stateList."commUpload_dataTrial" ("Enum") myRIO_BRig_RT__Case_Exp_stateList."commUpload_dataCurrent" ("Enum") myRIO_BRig_RT__Case_Exp_stateList."saveData_dataCurrent" ("Enum") myRIO_BRig_RT__Case_Exp_stateList."saveData_dataExp" ("Enum") myRIO_BRig_RT__Case_Exp_stateList."saveData_dataLC" ("Enum") myRIO_BRig_RT__Case_Exp_stateList."saveData_dataTrial" ("Enum") myRIO_BRig_RT__Case_Exp_stateList."commUpload_pre" ("Enum") w3540 w3569] -> w1647
            tunnel: [w1715 w1730 w1748 w1811 w1869 w1931 w1990 w2050 w2110 w2170 w2230 w2269 w2309 w2338 w2401 w2409 w2434 w2451 w2481 w2523 w2551 w2572 w2591 w2614 w2638 w2662 w2683 w2701 w2713 w2731 w2746 w2761 w2769 w2809 w2833 w2850 w2867 w2884 w2899 w2914 w2938 w2970 w2991 w3005 w3019 w3061 w3081 w3109 w3126 w3142 w3169 w3188 w3200 w3216 w3253 w3268 w3307 w3320 w3334 w3360 w3377 w3394 w3411 w3428 w3452 w3468 w3491 w3507 w3527 w3557 w3586] -> w1605
            tunnel: w1687 -> [w1715 w1730 w1748 w1811 w1869 w1931 w1990 w2050 w2110 w2170 w2230 w2269 w2309 w2338 w2401 w2411 w2434 w2451 w2481 w2523 w2551 w2572 w2591 w2614 w2638 w2662 w2683 w2701 w2713 w2731 w2746 w2761 w2769 w2809 w2833 w2850 w2867 w2884 w2899 w2914 w2938 w2970 w2991 w3005 w3019 w3061 w3081 w3109 w3126 w3142 w3169 w3188 w3200 w3216 w3253 w3268 w3307 w3320 w3334 w3360 w3377 w3394 w3411 w3428 w3452 w3468 w3491 w3507 w3527 w3557 w3586]
            tunnel: w1686 -> [w1718 w1733 w1745 w1814 w1872 w1934 w1993 w2053 w2113 w2173 w2233 w2272 w2312 w2341 w2404 w2426 w2441 w2465 w2500 w2534 w2561 w2580 w2600 w2623 w2629 w2649 w2686 w2704 w2719 w2734 w2749 w2764 w2773 w2792 w2839 w2857 w2872 w2887 w2902 w2917 w2937 w2969 w2996 w3015 w3046 w3069 w3092 w3112 w3125 w3154 w3174 w3185 w3204 w3215 w3260 w3290 w3311 w3317 w3339 w3363 w3380 w3397 w3414 w3431 w3455 w3471 w3494 w3510 w3530 w3560 w3589]
            tunnel: w1682 -> [w1717 w1732 w1746 w1813 w1871 w1933 w1992 w2052 w2112 w2172 w2232 w2271 w2311 w2340 w2403 w2425 w2440 w2466 w2499 w2535 w2562 w2581 w2601 w2624 w2642 w2664 w2685 w2703 w2718 w2733 w2748 w2763 w2783 w2810 w2838 w2856 w2871 w2886 w2901 w2916 w2919 w2945 w2995 w3014 w3045 w3068 w3091 w3111 w3124 w3153 w3173 w3186 w3205 w3214 w3259 w3289 w3310 w3318 w3340 w3362 w3379 w3396 w3413 w3430 w3454 w3470 w3493 w3509 w3529 w3559 w3588]
            tunnel: w1681 -> [w1716 w1731 w1747 w1812 w1870 w1932 w1991 w2051 w2111 w2171 w2231 w2270 w2310 w2339 w2402 w2424 w2439 w2467 w2498 w2536 w2563 w2582 w2602 w2625 w2641 w2663 w2684 w2702 w2717 w2732 w2747 w2762 w2782 w2811 w2837 w2855 w2870 w2885 w2900 w2915 w2918 w2944 w2994 w3013 w3044 w3067 w3090 w3110 w3123 w3152 w3172 w3187 w3206 w3213 w3258 w3288 w3309 w3319 w3341 w3361 w3378 w3395 w3412 w3429 w3453 w3469 w3492 w3508 w3528 w3558 w3587]
            tunnel: [w1718 w1733 w1745 w1814 w1872 w1934 w1993 w2053 w2113 w2173 w2233 w2272 w2312 w2341 w2404 w2426 w2441 w2465 w2500 w2534 w2561 w2580 w2600 w2623 w2629 w2649 w2686 w2704 w2719 w2734 w2749 w2764 w2773 w2792 w2839 w2857 w2872 w2887 w2902 w2917 w2937 w2969 w2996 w3015 w3046 w3069 w3092 w3112 w3125 w3154 w3174 w3185 w3204 w3215 w3260 w3290 w3311 w3317 w3339 w3363 w3380 w3397 w3414 w3431 w3455 w3471 w3494 w3510 w3530 w3560 w3589] -> w1670
            tunnel: [w1717 w1732 w1746 w1813 w1871 w1933 w1992 w2052 w2112 w2172 w2232 w2271 w2311 w2340 w2403 w2425 w2440 w2466 w2499 w2535 w2562 w2581 w2601 w2624 w2642 w2664 w2685 w2703 w2718 w2733 w2748 w2763 w2783 w2810 w2838 w2856 w2871 w2886 w2901 w2916 w2919 w2945 w2995 w3014 w3045 w3068 w3091 w3111 w3124 w3153 w3173 w3186 w3205 w3214 w3259 w3289 w3310 w3318 w3340 w3362 w3379 w3396 w3413 w3430 w3454 w3470 w3493 w3509 w3529 w3559 w3588] -> w1669
            tunnel: [w1716 w1731 w1747 w1812 w1870 w1932 w1991 w2051 w2111 w2171 w2231 w2270 w2310 w2339 w2402 w2424 w2439 w2467 w2498 w2536 w2563 w2582 w2602 w2625 w2641 w2663 w2684 w2702 w2717 w2732 w2747 w2762 w2782 w2811 w2837 w2855 w2870 w2885 w2900 w2915 w2918 w2944 w2994 w3013 w3044 w3067 w3090 w3110 w3123 w3152 w3172 w3187 w3206 w3213 w3258 w3288 w3309 w3319 w3341 w3361 w3378 w3395 w3412 w3429 w3453 w3469 w3492 w3508 w3528 w3558 w3587] -> w1668
            tunnel: w1566 -> [w1714 w1729 w1744 w1778 w1854 w1873 w1935 w2049 w2109 w2169 w2229 w2268 w2308 w2336 w2355 w2417 w2433 w2463 w2470 w2510 w2550 w2571 w2590 w2613 w2630 w2652 w2677 w2700 w2714 w2730 w2745 w2760 w2772 w2794 w2832 w2854 w2868 w2883 w2898 w2913 w2931 w2958 w2971 w3010 w3021 w3066 w3082 w3108 w3122 w3143 w3171 w3184 w3197 w3218 w3235 w3266 w3306 w3321 w3342 w3357 w3374 w3391 w3408 w3419 w3445 w3460 w3480 w3504 w3520 w3539 w3568]
            tunnel: w1638 -> [w1713 w1728 w1743 w1809 w1867 w1928 w1987 w2047 w2107 w2167 w2227 w2266 w2306 w2329 w2347 w2414 w2438 w2462 w2468 w2505 w2553 w2564 w2594 w2617 w2640 w2661 w2676 w2698 w2716 w2729 w2744 w2759 w2768 w2808 w2830 w2849 w2869 w2882 w2897 w2912 w2921 w2946 w2992 w3012 w3038 w3062 w3083 w3106 w3121 w3145 w3168 w3183 w3203 w3207 w3234 w3281 w3305 w3322 w3343 w3356 w3373 w3390 w3407 w3420 w3449 w3465 w3476 w3503 w3524 w3554 w3583]
            tunnel: [w1714 w1729 w1744 w1778 w1854 w1873 w1935 w2049 w2109 w2169 w2229 w2268 w2308 w2336 w2354 w2416 w2433 w2456 w2469 w2509 w2550 w2570 w2589 w2612 w2627 w2651 w2678 w2699 w2714 w2730 w2745 w2760 w2771 w2788 w2831 w2852 w2868 w2883 w2898 w2913 w2930 w2957 w2993 w3009 w3039 w3065 w3084 w3107 w3122 w3146 w3170 w3184 w3196 w3217 w3235 w3264 w3306 w3321 w3342 w3357 w3374 w3391 w3408 w3419 w3445 w3460 w3480 w3504 w3520 w3539 w3568] -> w1579
            tunnel: [w1713 w1728 w1743 w1808 w1866 w1923 w1986 w2047 w2107 w2167 w2227 w2266 w2306 w2329 w2346 w2415 w2438 w2461 w2468 w2505 w2553 w2564 w2594 w2617 w2640 w2661 w2676 w2698 w2716 w2729 w2744 w2759 w2768 w2808 w2830 w2849 w2869 w2882 w2897 w2912 w2921 w2946 w2992 w3012 w3038 w3062 w3083 w3106 w3121 w3145 w3168 w3183 w3203 w3207 w3234 w3281 w3305 w3322 w3343 w3356 w3373 w3390 w3407 w3420 w3449 w3465 w3479 w3503 w3524 w3554 w3583] -> w1678
            tunnel: [_ _ _ _ _ _ _ _ _ _ _ _ _ _ _ _ _ _ _ _ _ _ _ _ _ _ _ _ _ _ _ _ _ _ _ _ _ _ _ _ _ _ _ w3003 _ _ _ _ _ _ _ _ _ _ _ _ _ _ _ _ _ _ _ _ _ _ _ _ _ _ _] -> w1596
            tunnel: [_ _ _ _ _ _ _ _ _ _ _ _ _ _ _ _ _ _ _ _ _ _ _ _ _ _ _ _ _ _ _ _ _ _ _ _ _ _ _ _ _ _ _ w3004 _ _ _ _ _ _ _ _ _ _ _ _ _ _ _ _ _ _ _ _ _ _ _ _ _ _ _] -> w1650
            tunnel: w1677 -> [w1711 w1726 w1741 w1780 w1856 w1929 w1988 w2048 w2108 w2168 w2228 w2267 w2307 w2334 w2398 w2406 w2435 w2446 w2491 w2532 w2559 w2567 w2586 w2609 w2639 w2660 w2673 w2694 w2715 w2727 w2742 w2757 w2781 w2807 w2829 w2847 w2865 w2880 w2895 w2910 w2943 w2967 w2989 w3011 w3023 w3059 w3080 w3104 w3119 w3144 w3167 w3181 w3199 w3222 w3256 w3277 w3303 w3324 w3345 w3354 w3371 w3388 w3405 w3425 w3439 w3462 w3486 w3501 w3522 w3552 w3581]
            tunnel: [w1711 w1726 w1741 w1780 w1856 w1929 w1988 w2048 w2108 w2168 w2228 w2267 w2307 w2334 w2398 w2405 w2432 w2446 w2491 w2532 w2559 w2567 w2586 w2609 w2639 w2660 w2673 w2694 w2715 w2727 w2742 w2757 w2781 w2807 w2829 w2847 w2865 w2880 w2895 w2910 w2943 w2967 w2989 w3011 w3022 w3059 w3080 w3104 w3119 w3144 w3167 w3181 w3198 w3222 w3256 w3277 w3303 w3324 w3345 w3354 w3371 w3388 w3405 w3425 w3439 w3462 w3486 w3501 w3522 w3552 w3581] -> w1676
            tunnel: w1675 -> [w1712 w1727 w1742 w1779 w1855 w1930 w1989 w2045 w2105 w2165 w2225 w2264 w2304 w2335 w2399 w2427 w2437 w2460 w2480 w2533 w2560 w2573 w2592 w2615 w2637 w2648 w2674 w2695 w2712 w2728 w2743 w2758 w2780 w2796 w2828 w2848 w2866 w2881 w2896 w2911 w2942 w2968 w2990 w3006 w3036 w3060 w3079 w3105 w3120 w3141 w3166 w3182 w3202 w3221 w3257 w3280 w3304 w3323 w3344 w3355 w3372 w3389 w3406 w3426 w3448 w3464 w3488 w3499 w3523 w3553 w3582]
            tunnel: [w1712 w1727 w1742 w1779 w1855 w1930 w1989 w2046 w2106 w2166 w2226 w2265 w2305 w2335 w2399 w2427 w2437 w2460 w2480 w2533 w2560 w2573 w2592 w2615 w2637 w2648 w2674 w2695 w2712 w2728 w2743 w2758 w2780 w2796 w2828 w2848 w2866 w2881 w2896 w2911 w2942 w2968 w2990 w3006 w3036 w3060 w3079 w3105 w3120 w3141 w3166 w3182 w3202 w3221 w3257 w3280 w3304 w3323 w3344 w3355 w3372 w3389 w3406 w3426 w3448 w3464 w3488 w3499 w3523 w3553 w3582] -> w1674
            tunnel: [_ _ _ _ _ _ _ _ _ _ _ _ _ _ _ _ _ _ _ _ _ _ _ _ _ _ _ _ _ _ _ _ _ _ _ _ _ _ _ _ _ _ _ _ _ _ _ _ _ _ _ _ _ _ _ _ TRUE _ _ _ _ _ _ _ _ _ _ _ _ _ _] -> w1671
            tunnel: w1662 -> [_ _ _ _ _ _ _ _ _ _ _ _ _ _ _ _ _ _ _ _ _ _ _ _ _ _ _ _ _ _ _ _ _ w2806 _ _ _ _ _ _ _ _ _ _ _ _ _ _ _ _ _ _ _ _ _ _ _ _ _ _ _ _ _ _ _ _ _ _ _ _ _]
            tunnel: w1661 -> [_ _ _ _ _ _ _ _ _ _ _ _ _ _ _ _ _ _ _ _ _ _ _ _ _ _ _ _ _ _ _ _ _ w2805 _ _ _ _ _ _ _ _ _ _ _ _ _ _ _ _ _ _ _ _ _ _ _ _ _ _ _ _ _ _ _ _ _ _ _ _ _]
            tunnel: [_ _ _ _ _ _ _ _ _ _ _ _ _ _ _ _ _ _ _ _ _ _ _ _ _ _ _ _ _ _ _ _ w2767 w2806 _ _ _ _ _ _ _ _ _ _ _ _ _ _ _ _ _ _ _ _ _ _ _ _ _ _ _ _ _ _ _ _ _ _ _ _ _] -> w1637
            tunnel: [_ _ _ _ _ _ _ _ _ _ _ _ _ _ _ _ _ _ _ _ _ _ _ _ _ _ _ _ _ _ _ _ w2766 w2805 _ _ _ _ _ _ _ _ _ _ _ _ _ _ _ _ _ _ _ _ _ _ _ _ _ _ _ _ _ _ _ _ _ _ _ _ _] -> w1636
            tunnel: w1646 -> [w1709 w1724 w1739 w1770 w1852 w1918 w1985 w2032 w2097 w2152 w2212 w2239 w2289 w2328 w2397 w2423 w2436 w2459 w2483 w2525 w2549 w2569 w2588 w2611 w2636 w2659 w2671 w2693 w2710 w2725 w2740 w2755 w2779 w2804 w2826 w2846 w2863 w2878 w2893 w2908 w2941 w2966 w2979 w3002 w3034 w3058 w3075 w3098 w3118 w3137 w3160 w3180 w3195 w3220 w3249 w3276 w3301 w3325 w3346 w3353 w3370 w3387 w3404 w3424 w3447 w3463 w3487 w3502 w3517 w3551 w3580]
            tunnel: [w1709 w1724 w1739 w1770 w1852 w1918 w1985 w2032 w2097 w2152 w2212 w2239 w2289 w2328 w2397 w2423 w2436 w2459 w2482 w2524 w2542 w2568 w2587 w2610 w2636 w2659 w2671 w2693 w2710 w2725 w2740 w2755 w2779 w2804 w2826 w2846 w2863 w2878 w2893 w2908 w2941 w2966 w2979 w3002 w3034 w3058 w3075 w3098 w3118 w3137 w3160 w3180 w3195 w3219 w3249 w3276 w3301 w3325 w3346 w3353 w3370 w3387 w3404 w3424 w3447 w3463 w3487 w3502 w3517 w3551 w3580] -> w1645
            tunnel: [w1708 w1723 w1738 w1769 w1851 w1917 w1984 w2031 w2096 w2151 w2211 w2238 w2288 w2327 w2396 w2422 w2443 w2458 w2493 w2531 w2558 w2579 w2599 w2622 w2635 w2658 w2670 w2692 w2709 w2724 w2739 w2754 w2778 w2803 w2825 w2845 w2862 w2877 w2892 w2907 w2940 w2965 w2978 w3001 w3033 w3057 w3074 w3097 w3117 w3136 w3159 w3179 w3194 w3212 w3255 w3275 w3299 w3326 w3336 w3352 w3369 w3386 w3403 w3423 w3451 w3467 w3490 w3506 w3526 w3556 w3585] -> w1644
            tunnel: [w1707 w1722 w1737 w1768 w1850 w1916 w1983 w2030 w2095 w2150 w2210 w2237 w2287 w2326 w2395 w2421 w2442 w2457 w2492 w2530 w2557 w2578 w2598 w2621 w2634 w2657 w2669 w2691 w2708 w2723 w2738 w2753 w2777 w2802 w2824 w2844 w2861 w2876 w2891 w2906 w2939 w2964 w2977 w3000 w3032 w3056 w3073 w3096 w3116 w3135 w3158 w3178 w3193 w3211 w3254 w3274 w3300 w3312 w3333 w3358 w3375 w3392 w3409 w3427 w3450 w3466 w3489 w3505 w3525 w3555 w3584] -> w1643
            tunnel: w1642 -> [w1708 w1723 w1738 w1769 w1851 w1917 w1984 w2031 w2096 w2151 w2211 w2238 w2288 w2327 w2396 w2422 w2443 w2458 w2493 w2531 w2558 w2579 w2599 w2622 w2635 w2658 w2670 w2692 w2709 w2724 w2739 w2754 w2778 w2803 w2825 w2845 w2862 w2877 w2892 w2907 w2940 w2965 w2978 w3001 w3033 w3057 w3074 w3097 w3117 w3136 w3159 w3179 w3194 w3212 w3255 w3275 w3299 _ w3336 w3352 w3369 w3386 w3403 w3423 w3451 w3467 w3490 w3506 w3526 w3556 w3585]
            tunnel: w1641 -> [w1707 w1722 w1737 w1768 w1850 w1916 w1983 w2030 w2095 w2150 w2210 w2237 w2287 w2326 w2395 w2421 w2442 w2457 w2492 w2530 w2557 w2578 w2598 w2621 w2634 w2657 w2669 w2691 w2708 w2723 w2738 w2753 w2777 w2802 w2824 w2844 w2861 w2876 w2891 w2906 w2939 w2964 w2977 w3000 w3032 w3056 w3073 w3096 w3116 w3135 w3158 w3178 w3193 w3211 w3254 w3274 w3300 _ w3333 w3358 w3375 w3392 w3409 w3427 w3450 w3466 w3489 w3505 w3525 w3555 w3584]
            tunnel: w1640 -> [_ _ _ _ _ _ _ _ _ _ _ _ _ _ _ _ _ _ _ _ _ _ _ _ _ _ _ _ _ _ _ _ _ _ _ _ _ _ _ _ _ _ _ _ _ _ _ _ _ _ _ _ _ _ _ _ _ _ _ w3350 w3367 w3384 w3401 w3421 _ _ _ _ _ _ _]
            tunnel: w1639 -> [_ _ _ _ _ _ _ _ _ _ _ _ _ _ _ _ _ _ _ _ _ _ _ _ _ _ _ _ _ _ _ _ _ _ _ _ _ _ _ _ _ _ _ _ _ _ _ _ _ _ _ _ _ _ _ _ _ _ _ _ _ _ _ _ _ _ w3481 _ _ _ _]
            tunnel: [w1706 w1721 w1736 w1767 w1849 w1915 w1982 w2029 w2094 w2149 w2209 w2236 w2286 w2325 w2394 w2412 w2430 w2455 w2494 w2529 w2556 w2577 w2597 w2620 w2633 w2656 w2668 w2690 w2707 w2722 w2737 w2752 w2776 w2801 w2823 w2843 w2860 w2875 w2890 w2905 w2936 w2963 w2976 w2999 w3017 w3055 w3072 w3095 w3115 w3134 w3157 w3177 w3192 w3210 w3252 w3261 w3298 w3315 w3335 w3349 w3366 w3383 w3400 w3418 w3434 w3459 w3475 w3498 w3515 w3550 w3579] -> w1634
            tunnel: w1635 -> [w1706 w1721 w1736 w1767 w1849 w1915 w1982 w2029 w2094 w2149 w2209 w2236 w2286 w2325 w2394 _ _ w2455 w2494 w2529 w2556 w2577 w2597 w2620 w2633 w2656 w2668 w2690 w2707 w2722 w2737 w2752 w2776 w2801 w2823 w2843 w2860 w2875 w2890 w2905 w2936 w2963 w2976 w2999 w3017 w3055 w3072 w3095 w3115 w3134 w3157 w3177 w3192 w3210 w3252 w3262 w3298 w3315 w3335 w3349 w3366 w3383 w3400 w3418 w3434 w3459 w3475 w3498 w3515 w3550 w3579]
            tunnel: w1633 -> [w1705 w1720 w1735 w1766 w1848 w1914 w1981 w2028 w2093 w2148 w2208 w2235 w2285 w2324 w2393 w2420 w2429 w2454 w2490 w2528 w2555 w2576 w2596 w2619 w2632 w2655 w2667 w2689 w2706 w2721 w2736 w2751 w2775 w2800 w2822 w2842 w2859 w2874 w2889 w2904 w2935 w2962 w2975 w2998 w3031 w3054 w3071 w3094 w3114 w3133 w3156 w3176 w3191 w3209 w3251 w3273 w3297 w3314 w3338 w3348 w3365 w3382 w3399 w3417 w3433 w3458 w3474 w3497 w3514 w3549 w3578]
            tunnel: w1632 -> [w1704 w1719 w1734 w1765 w1847 w1913 w1980 w2027 w2092 w2147 w2207 w2234 w2284 w2323 w2392 w2419 w2428 w2453 w2489 w2527 w2554 w2575 w2595 w2618 w2631 w2654 w2666 w2688 w2705 w2720 w2735 w2750 w2774 w2799 w2821 w2841 w2858 w2873 w2888 w2903 w2934 w2961 w2974 w2997 w3028 w3053 w3070 w3093 w3113 w3132 w3155 w3175 w3190 w3208 w3250 w3272 w3296 w3313 w3337 w3347 w3364 w3381 w3398 w3416 w3432 w3457 w3473 w3496 w3513 w3548 w3577]
            tunnel: [w1705 w1720 w1735 w1766 w1848 w1914 w1981 w2028 w2093 w2148 w2208 w2235 w2285 w2324 w2393 w2420 w2429 w2454 w2490 w2528 w2555 w2576 w2596 w2619 w2632 w2655 w2667 w2689 w2706 w2721 w2736 w2751 w2775 w2800 w2822 w2842 w2859 w2874 w2889 w2904 w2935 w2962 w2975 w2998 w3030 w3054 w3071 w3094 w3114 w3133 w3156 w3176 w3191 w3209 w3251 w3273 w3297 w3314 w3338 w3348 w3365 w3382 w3399 w3417 w3433 w3458 w3474 w3497 w3514 w3549 w3578] -> w1631
            tunnel: [w1704 w1719 w1734 w1765 w1847 w1913 w1980 w2027 w2092 w2147 w2207 w2234 w2284 w2323 w2392 w2419 w2428 w2453 w2489 w2527 w2554 w2575 w2595 w2618 w2631 w2654 w2666 w2688 w2705 w2720 w2735 w2750 w2774 w2799 w2821 w2841 w2858 w2873 w2888 w2903 w2934 w2961 w2974 w2997 w3029 w3053 w3070 w3093 w3113 w3132 w3155 w3175 w3190 w3208 w3250 w3272 w3296 w3313 w3337 w3347 w3364 w3381 w3398 w3416 w3432 w3457 w3473 w3496 w3513 w3548 w3577] -> w1630
            tunnel: w1629 -> [w1703 _ _ _ _ _ _ _ _ _ _ _ _ w2320 w2389 _ _ w2450 w2497 w2519 w2540 _ _ w2605 _ _ _ _ _ _ _ _ _ w2798 _ _ _ _ _ _ w2932 w2960 _ _ _ _ _ _ _ w3131 _ _ _ _ w3231 _ w3294 _ _ _ _ _ _ _ _ _ _ _ _ _ _]
            tunnel: w1628 -> [w1702 _ _ _ _ _ _ _ _ _ _ _ _ w2319 w2390 _ _ w2449 w2496 w2518 w2539 _ _ w2604 _ _ _ _ _ _ _ _ _ w2797 _ _ _ _ _ _ w2933 w2959 _ _ _ _ _ _ _ w3130 _ _ _ _ w3230 _ w3293 _ _ _ _ _ _ _ _ _ _ _ _ _ _]
            tunnel: [_ _ _ _ _ _ _ _ _ _ _ _ _ _ _ _ _ _ _ _ _ _ _ _ _ w2646 _ _ _ _ _ _ _ w2784 _ _ _ _ _ _ w2925 w2951 _ _ _ _ _ _ _ _ _ _ _ _ _ _ _ _ _ _ _ _ _ _ _ _ _ _ _ _ _] -> w1587
            tunnel: [_ _ _ _ _ _ _ _ _ _ _ _ _ _ _ _ _ _ _ _ _ _ _ _ _ w2645 _ _ _ _ _ _ _ w2785 _ _ _ _ _ _ w2924 w2950 _ _ _ _ _ _ _ _ _ _ _ _ _ _ _ _ _ _ _ _ _ _ _ _ _ _ _ _ _] -> w1586
            tunnel: [_ _ _ _ _ _ _ _ _ _ _ _ _ _ _ _ _ _ _ _ _ _ TRUE ("Recording") _ _ _ _ _ _ _ _ _ _ _ _ _ _ _ _ _ _ _ _ _ _ _ _ _ _ _ _ _ _ _ _ _ _ _ _ _ _ _ _ _ _ _ _ _ _ _ _] -> w1623
            tunnel: [_ _ _ _ _ _ _ _ _ _ _ _ _ _ _ TRUE _ _ _ _ _ _ _ _ _ _ _ _ _ _ _ _ _ _ _ _ _ _ _ _ _ _ _ _ _ _ _ _ _ _ _ _ _ _ _ _ _ _ _ _ _ _ _ _ _ _ _ _ _ _ _] -> w1620
            tunnel: [_ _ _ _ _ _ _ _ _ _ _ _ _ _ _ _ _ TRUE _ _ _ _ _ _ _ _ _ _ _ _ _ _ _ _ _ _ _ _ _ _ _ _ _ _ _ _ _ _ _ _ _ _ _ _ _ _ _ _ _ _ _ _ _ _ _ _ _ _ _ _ _] -> w1618
            tunnel: [_ _ _ _ _ _ _ _ _ _ _ _ _ _ _ _ _ w2445 _ _ _ _ _ _ _ _ _ _ _ _ _ _ _ _ _ _ _ _ _ _ _ _ _ _ _ _ _ _ _ _ _ _ _ _ _ _ _ _ _ _ _ _ _ _ _ _ _ _ _ _ _] -> w1617
            tunnel: w1604 -> [_ _ _ _ _ _ _ _ _ _ _ _ _ _ _ _ _ _ _ _ _ _ _ _ _ _ _ _ _ _ _ _ _ _ _ _ _ _ _ _ _ _ _ _ _ _ _ _ _ _ _ _ _ _ _ _ _ _ _ _ _ _ _ _ _ _ _ _ _ w3546 w3575]
            tunnel: [_ _ _ _ _ _ _ _ _ _ _ _ _ _ _ _ _ _ _ _ _ _ _ _ _ _ _ _ _ _ _ _ _ _ _ _ _ _ _ _ _ _ _ _ _ _ _ _ _ _ _ _ _ _ _ _ _ _ _ _ _ _ _ _ _ _ _ _ _ w3544 w3573] -> w1603
            tunnel: w1599 -> [_ _ _ _ _ _ _ _ _ _ _ _ _ _ _ _ _ _ _ _ w2541 w2566 w2585 w2608 w2626 w2647 w2665 w2687 _ _ _ _ w2765 w2795 w2820 w2840 _ _ _ _ w2926 w2952 _ _ _ _ _ _ _ _ _ _ _ _ _ _ _ _ _ _ _ _ _ _ _ _ _ _ _ _ _]
            tunnel: [_ _ _ _ _ _ _ _ _ _ _ _ _ _ _ _ _ _ _ w2507 w2541 w2565 w2584 w2607 w2626 w2647 w2665 w2687 _ _ _ _ w2765 w2795 w2820 w2840 _ _ _ _ w2926 w2952 _ _ _ _ _ _ _ _ _ _ _ _ _ _ _ _ _ _ _ _ _ _ _ _ _ _ _ _ _] -> w1598
            tunnel: [_ _ _ _ _ _ _ _ _ _ _ _ _ _ _ _ _ _ _ _ _ _ _ _ _ w2644 _ _ _ _ _ _ _ w2789 _ _ _ _ _ _ w2923 w2949 _ _ _ _ _ _ _ _ _ _ _ _ _ _ _ _ _ _ _ _ _ _ _ _ _ _ _ _ _] -> w1591
            tunnel: [_ _ _ _ _ _ _ _ _ _ _ _ _ _ _ _ _ _ _ _ _ _ _ _ _ w2643 _ _ _ _ _ _ _ w2790 _ _ _ _ _ _ w2922 w2948 _ _ _ _ _ _ _ _ _ _ _ _ _ _ _ _ _ _ _ _ _ _ _ _ _ _ _ _ _] -> w1589
            tunnel: [_ _ _ _ _ _ _ _ _ _ _ _ _ _ _ _ _ _ _ _ _ _ _ _ _ _ _ _ _ _ _ _ _ w2791 _ _ _ _ _ _ _ _ _ _ _ _ _ _ _ _ _ _ _ _ _ _ _ _ _ _ _ _ _ _ _ _ _ _ _ _ _] -> w1595
            tunnel: [_ _ _ _ _ _ _ _ _ _ _ _ _ _ _ w2407 _ _ _ _ _ _ _ _ _ _ _ _ _ _ _ _ _ _ _ _ _ _ _ _ _ _ _ _ _ _ _ _ _ _ _ _ _ _ _ _ _ _ _ _ _ _ _ _ _ _ _ _ _ _ _] -> w1578
            frame "Start1", Default {
              w1701 = FALSE ("SelectionState")
              n993 = xnode "Read/Write Control"("FPGA VI Reference In"=w1703, "error in"=w1702, "SelectionState"=w1701, "LR_reward_Laser_l1"=w1701, "LR_wrong_Laser_l1"=w1701, "LR_reward_Event_l1"=w1701, "LR_wrong_Event_l1"=w1701, "Left(F)_or_Right(T)"=w1701, "ignoreWrong"=w1701, "SelectionState"=w1701, "LR_reward_Laser_l2"=w1701, "LR_wrong_laser_l2"=w1701, "LR_reward_Event_l2"=w1701, "LR_wrong_Event_l2"=w1701, "LC_Event_l1"=w1701, "LC_Laser_l1"=w1701, "LC_Laser_l2"=w1701, "LC_Event_l2"=w1701, "CueLed_Event"=w1701, "I_allReward"=w1701) -> ()  [unwired: 2 out]
            }
            frame "Start2" {
            }
            frame "Start3" {
            }
            frame "saveSettings1" {
              n994 = call "myRIO_BRig_RT_dataExp_Tcycle_Reward_min_L.vi"() -> ("output_Tcycle_Reward_min_L"=w1754:i32)  [unwired: 11 in]
              n995 = local read "Tcycle_Reward_min_L"() -> (w1753:u16)
              n996 = call "myRIO_BRig_RT_dataExp_Audio_freq__L.vi"() -> ("output_Audio_freq__L"=w1786:i32)  [unwired: 11 in]
              n997 = call "myRIO_BRig_RT_dataExp_Audio_freq__R.vi"() -> ("output_Audio_freq__R"=w1785:i32)  [unwired: 11 in]
              n998 = call "myRIO_BRig_RT_dataExp_Audio_amp__L.vi"() -> ("output_Audio_amp__L"=w1784:i32)  [unwired: 11 in]
              n999 = call "myRIO_BRig_RT_dataExp_Audio_amp__R.vi"() -> ("output_Audio_amp__R"=w1782:i32)  [unwired: 11 in]
              n1000 = call "myRIO_BRig_RT_dataExp_TPB_min__L.vi"() -> ("output_TPB_min__L"=w1794:i32)  [unwired: 11 in]
              n1001 = call "myRIO_BRig_RT_dataExp_TPB_min__R.vi"() -> ("output_TPB_min__R"=w1792:i32)  [unwired: 11 in]
              n1002 = call "myRIO_BRig_RT_dataExp_TPB_max__L.vi"() -> ("output_TPB_max__L"=w1790:i32)  [unwired: 11 in]
              n1003 = call "myRIO_BRig_RT_dataExp_TPB_max__R.vi"() -> ("output_TPB_max__R"=w1788:i32)  [unwired: 11 in]
              n1004 = call "myRIO_BRig_RT_dataExp_Cue1Param_AudioLed_Count_Switch.vi"() -> ("output_Cue1Param_AudioLed_Count_Switch"=w1760:i32)  [unwired: 11 in]
              n1005 = call "myRIO_BRig_RT_dataExp_Cue1Param_AudioLed_Probability_Switch.vi"() -> ("output_Cue1Param_AudioLed_Probability_Switch"=w1758:i32)  [unwired: 11 in]
              n1006 = call "myRIO_BRig_RT_dataExp_Cue1Param_CueType_Switch.vi"() -> ("output_Cue1Param_CueType_Switch"=w1756:i32)  [unwired: 11 in]
              n1007 = call "myRIO_BRig_RT_dataExp_ItrialUntilReward.vi"() -> ("output_I_trialUntilReward"=w1807:i32)  [unwired: 11 in]
              n1008 = call "myRIO_BRig_RT_dataExp_IblockUntilReward.vi"() -> ("output_I_blockUntilReward"=w1803:i32)  [unwired: 11 in]
              n1009 = call "myRIO_BRig_RT_dataExp_CueCycles.vi"() -> ("output_CueCycles"=w1802:i32)  [unwired: 11 in]
              n1010 = call "myRIO_BRig_RT_dataExp_ENL_min.vi"() -> ("output_ENL_min"=w1800:i32)  [unwired: 11 in]
              n1011 = call "myRIO_BRig_RT_dataExp_ENL_max.vi"() -> ("output_ENL_max"=w1798:i32)  [unwired: 11 in]
              n1012 = call "myRIO_BRig_RT_dataExp_ENL_penalty.vi"() -> ("output_ENL_penalty"=w1796:i32)  [unwired: 11 in]
              n1013 = local read "Audio_Freq__L"() -> (w1764:u8)
              n1014 = local read "Audio_Freq__R"() -> (w1762:u8)
              n1015 = local read "Audio_Amp__L"() -> (w1783:u16)
              n1016 = local read "TpB_Min_L"() -> (w1793:u16)
              n1017 = local read "TpB_Min_R"() -> (w1791:u16)
              n1018 = local read "TpB_Max_L"() -> (w1789:u16)
              n1019 = local read "TpB_Max_R"() -> (w1787:u16)
              n1020 = local read "Audio_Amp__R"() -> (w1781:u16)
              n1021 = local read "TrialUntilReward"() -> (w1806:bool)
              n1022 = local read "CueCycles"() -> (w1801:u16)
              n1023 = local read "Tcycle_ENL_min"() -> (w1799:u16)
              n1024 = local read "Tcycle_ENL_max"() -> (w1797:u16)
              n1025 = local read "Tcycle_ENLPenalty"() -> (w1795:u16)
              n1026 = local read "Cue1Param_AudioLed_Count_Switch"() -> (w1759:u16)
              n1027 = local read "Cue1Param_AudioLed_Probability_Switch"() -> (w1757:u16)
              n1028 = local read "Cue1Param_CueType_Switch"() -> (w1755:u16)
              n1029 = local read "Tcycle_Reward_max_L"() -> (w1751:u16)
              n1030 = call "myRIO_BRig_RT_dataExp_Tcycle_Reward_max_L.vi"() -> ("output_Tcycle_Reward_max_L"=w1752:i32)  [unwired: 11 in]
              n1031 = To Unsigned Word Integer(number=w1762) -> (unsigned 16bit integer=w1761:u16)
              n1032 = To Unsigned Word Integer(number=w1764) -> (unsigned 16bit integer=w1763:u16)
              n1033 = Boolean To (0,1)(Boolean=w1806) -> (0, 1=w1805:i16)
              n1034 = To Unsigned Word Integer(number=w1805) -> (unsigned 16bit integer=w1804:u16)
              n1035 = call "myRIO_BRig_RT_dataExp_Tcycle_Reward_step_L.vi"() -> ("output_Tcycle_Reward_step_L"=w1750:i32)  [unwired: 11 in]
              n1036 = local read "Tcycle_Reward_step_L"() -> (w1749:u16)
              n1037 = local read "BUR_min"() -> (w1775:u16)
              n1038 = local read "BUR_max"() -> (w1776:u16)
              n1039 = Not Equal To 0?(x=w1775) -> (x != 0?=w1774:bool)
              n1040 = Not Equal To 0?(x=w1776) -> (x != 0?=w1773:bool)
              n1041 = And(x=w1774, y=w1773) -> (x .and. y?=w1772:bool)
              n1042 = Boolean To (0,1)(Boolean=w1772) -> (0, 1=w1777:i16)
              n1043 = To Unsigned Word Integer(number=w1777) -> (unsigned 16bit integer=w1771:u16)
              n1044 = Replace Array Subset(array=w1809, new element #1=w1804, index #1=w1807, new element #2=w1771, index #2=w1803, new element #3=w1801, index #3=w1802, new element #4=w1799, index #4=w1800, new element #5=w1797, index #5=w1798, new element #6=w1795, index #6=w1796, new element #7=w1793, index #7=w1794, new element #8=w1791, index #8=w1792, new element #9=w1789, index #9=w1790, new element #10=w1787, index #10=w1788, new element #11=w1763, index #11=w1786, new element #12=w1761, index #12=w1785, new element #13=w1783, index #13=w1784, new element #14=w1781, index #14=w1782, new element #15=w1759, index #15=w1760, new element #16=w1757, index #16=w1758, new element #17=w1755, index #17=w1756, new element #18=w1753, index #18=w1754, new element #19=w1751, index #19=w1752, new element #20=w1749, index #20=w1750) -> (w1808:u16[])
            }
            frame "saveSettings2" {
              n1045 = call "myRIO_BRig_RT_dataExp_Tcycle_Reward_min_R.vi"() -> ("output_Tcycle_Reward_min_R"=w1828:i32)  [unwired: 11 in]
              n1046 = local read "Tcycle_Reward_min_R"() -> (w1827:u16)
              n1047 = call "myRIO_BRig_RT_dataExp_Tcycle_Cue1_Audio_min.vi"() -> ("output_Tcycle_Cue1_Audio_min"=w1859:i32)  [unwired: 11 in]
              n1048 = call "myRIO_BRig_RT_dataExp_Tcycle_Cue1_Audio_max.vi"() -> ("output_Tcycle_Cue1_Audio_max"=w1858:i32)  [unwired: 11 in]
              n1049 = call "myRIO_BRig_RT_dataExp_Tcycle_Cue1Penalty_Audio.vi"() -> ("output_Tcycle_Cue1Penalty_Audio"=w1857:i32)  [unwired: 11 in]
              n1050 = call "myRIO_BRig_RT_dataExp_Tcycle_RewardPost.vi"() -> ("output_Tcycle_RewardPost"=w1865:i32)  [unwired: 11 in]
              n1051 = call "myRIO_BRig_RT_dataExp_Tcycle_Wrong.vi"() -> ("output_Tcycle_Wrong"=w1863:i32)  [unwired: 11 in]
              n1052 = call "myRIO_BRig_RT_dataExp_Tcycle_Timeout.vi"() -> ("output_Tcycle_Timeout"=w1861:i32)  [unwired: 11 in]
              n1053 = call "myRIO_BRig_RT_dataExp_Tcycle_Cue1_LED_min.vi"() -> ("output_Tcycle_Cue1_LED_min"=w1834:i32)  [unwired: 11 in]
              n1054 = call "myRIO_BRig_RT_dataExp_Tcycle_Cue1_LED_max.vi"() -> ("output_Tcycle_Cue1_LED_max"=w1833:i32)  [unwired: 11 in]
              n1055 = call "myRIO_BRig_RT_dataExp_Tcycle_Cue1Penalty_LED.vi"() -> ("output_Tcycle_Cue1Penalty_LED"=w1832:i32)  [unwired: 11 in]
              n1056 = call "myRIO_BRig_RT_dataExp_SolenoidProbability_L.vi"() -> ("output_SolenoidProbability_L"=w1844:i32)  [unwired: 11 in]
              n1057 = call "myRIO_BRig_RT_dataExp_SolenoidProbability_R.vi"() -> ("output_SolenoidProbability_R"=w1843:i32)  [unwired: 11 in]
              n1058 = call "myRIO_BRig_RT_dataExp_Cue1Param_AudioLed_Count_NS.vi"() -> ("output_Cue1Param_AudioLed_Count_NS"=w1840:i32)  [unwired: 11 in]
              n1059 = call "myRIO_BRig_RT_dataExp_Cue1Param_AudioLed_Probability_NS.vi"() -> ("output_Cue1Param_AudioLed_Probability_NS"=w1838:i32)  [unwired: 11 in]
              n1060 = call "myRIO_BRig_RT_dataExp_Cue1Param_CueType_NS.vi"() -> ("output_Cue1Param_CueType_NS"=w1836:i32)  [unwired: 11 in]
              n1061 = call "myRIO_BRig_RT_dataExp_nBlock.vi"() -> ("output_nBlock"=w1815:i32)  [unwired: 11 in]
              n1062 = call "myRIO_BRig_RT_dataExp_nTrial.vi"() -> ("output_nTrial"=w1817:i32)  [unwired: 11 in]
              n1063 = call "myRIO_BRig_RT_dataExp_runTime_seconds.vi"() -> ("output_RunTime_minutes"=w1820:i32)  [unwired: 11 in]
              n1064 = call "myRIO_BRig_RT_dataExp_Tcycle_Selection.vi"() -> ("output_Tcycle_Selection"=w1822:i32)  [unwired: 11 in]
              n1065 = local read "Tcycle_CuePenalty_Audio"() -> (w1853:u16)
              n1066 = local read "Tcycle_Cue_Audio_max"() -> (w1845:u16)
              n1067 = local read "Tcycle_Cue_Audio_min"() -> (w1846:u16)
              n1068 = local read "Tcycle_RewardPost"() -> (w1864:u16)
              n1069 = local read "Tcycle_Wrong"() -> (w1862:u16)
              n1070 = local read "Tcycle_Timeout"() -> (w1860:u16)
              n1071 = local read "Tcycle_Selection"() -> (w1821:u16)
              n1072 = local read "Cue1Param_AudioLed_Count_NS"() -> (w1839:u16)
              n1073 = local read "Cue1Param_AudioLed_Probability_NS"() -> (w1837:u16)
              n1074 = local read "Cue1Param_CueType_NS"() -> (w1835:u16)
              n1075 = local read "Tcycle_CuePenalty_LED"() -> (w1829:u16)
              n1076 = local read "SolenoidProbability_R"() -> (w1841:u16)
              n1077 = local read "SolenoidProbability_L"() -> (w1842:u16)
              n1078 = local read "Tcycle_Cue_LED_min"() -> (w1831:u16)
              n1079 = local read "Tcycle_Cue_LED_max"() -> (w1830:u16)
              n1080 = local read "Tcycle_Reward_max_R"() -> (w1825:u16)
              n1081 = call "myRIO_BRig_RT_dataExp_Tcycle_Reward_max_R.vi"() -> ("output_Tcycle_Reward_max_R"=w1826:i32)  [unwired: 11 in]
              n1082 = call "myRIO_BRig_RT_dataExp_Tcycle_Reward_step_R.vi"() -> ("output_Tcycle_Reward_step_R"=w1824:i32)  [unwired: 11 in]
              n1083 = local read "Tcycle_Reward_step_R"() -> (w1823:u16)
              n1084 = Replace Array Subset(array=w1867, new element #1=u16 0, index #1=w1815, new element #2=u16 0, index #2=w1817, new element #3=u16 0, index #3=w1820, new element #4=w1821, index #4=w1822, new element #5=w1864, index #5=w1865, new element #6=w1862, index #6=w1863, new element #7=w1860, index #7=w1861, new element #8=w1846, index #8=w1859, new element #9=w1845, index #9=w1858, new element #10=w1853, index #10=w1857, new element #11=w1842, index #11=w1844, new element #12=w1841, index #12=w1843, new element #13=w1839, index #13=w1840, new element #14=w1837, index #14=w1838, new element #15=w1835, index #15=w1836, new element #16=w1831, index #16=w1834, new element #17=w1830, index #17=w1833, new element #18=w1829, index #18=w1832, new element #19=w1827, index #19=w1828, new element #20=w1825, index #20=w1826, new element #21=w1823, index #21=w1824) -> (w1866:u16[])
            }
            frame "saveSettings3" {
              w1879 = 100.0 ("y")
              n1085 = call "myRIO_BRig_RT_dataExp_laser1_Freq.vi"() -> ("output_laser1_Freq"=w1912:i32)  [unwired: 11 in]
              n1086 = call "myRIO_BRig_RT_dataExp_laser1_Tpeak.vi"() -> ("output_laser1_Tpeak"=w1907:i32)  [unwired: 11 in]
              n1087 = call "myRIO_BRig_RT_dataExp_laser1_Tshutter.vi"() -> ("output_laser1_Tshutter"=w1902:i32)  [unwired: 11 in]
              n1088 = call "myRIO_BRig_RT_dataExp_FPGA_f_count2ms.vi"() -> ("output_FPGA_f_count2ms"=w1897:i32)  [unwired: 11 in]
              n1089 = call "myRIO_BRig_RT_dataExp_laser1_Power_min.vi"() -> ("output_laser1_Power_min"=w1892:i32)  [unwired: 11 in]
              n1090 = call "myRIO_BRig_RT_dataExp_laser1_Power_max.vi"() -> ("output_laser1_Power_max"=w1885:i32)  [unwired: 11 in]
              n1091 = call "myRIO_BRig_RT_dataExp_laser1_Power_step.vi"() -> ("output_laser1_Power_step"=w1884:i32)  [unwired: 11 in]
              n1092 = call "myRIO_BRig_RT_dataExp_laser1_duration.vi"() -> ("output_laser1_duration"=w1887:i32)  [unwired: 11 in]
              n1093 = local read "Laser_Tshutter_l1"() -> (w1899:dbl)
              n1094 = local read "Laser_Tpeak_l1"() -> (w1904:dbl)
              n1095 = local read "Laser_power_max_l1"() -> (w1878:dbl)
              n1096 = local read "Laser_power_step_l1"() -> (w1877:dbl)
              n1097 = local read "Laser_power_min_l1"() -> (w1889:dbl)
              n1098 = local read "Laser_Freq_l1"() -> (w1911:dbl)
              n1099 = call "myRIO_BRig_RT_dataExp_BUR_min.vi"() -> ("output_BUR_min"=w1927:i32)  [unwired: 11 in]
              n1100 = call "myRIO_BRig_RT_dataExp_BUR_max.vi"() -> ("output_BUR_max"=w1925:i32)  [unwired: 11 in]
              n1101 = call "myRIO_BRig_RT_dataExp_Audio_sp__L.vi"() -> ("output_Audio_sp__L"=w1922:i32)  [unwired: 11 in]
              n1102 = call "myRIO_BRig_RT_dataExp_Audio_sp__R.vi"() -> ("output_Audio_sp__R"=w1921:i32)  [unwired: 11 in]
              n1103 = local read "FPGA_count2ms"() -> (w1894:dbl)
              n1104 = local read "sp_LeftSpout"() -> (w1920:u16)
              n1105 = local read "BUR_max"() -> (w1924:u16)
              n1106 = local read "sp_RightSpout"() -> (w1919:u16)
              n1107 = local read "BUR_min"() -> (w1926:u16)
              n1108 = Multiply(x=w1911, y=w1879) -> (x*y=w1910:dbl)
              n1109 = Multiply(x=w1904, y=w1879) -> (x*y=w1906:dbl)
              n1110 = Multiply(x=w1899, y=w1879) -> (x*y=w1901:dbl)
              n1111 = Multiply(x=w1894, y=w1879) -> (x*y=w1896:dbl)
              n1112 = Multiply(x=w1889, y=w1879) -> (x*y=w1891:dbl)
              n1113 = Multiply(x=w1878, y=w1879) -> (x*y=w1883:dbl)
              n1114 = Multiply(x=w1877, y=w1879) -> (x*y=w1881:dbl)
              n1115 = Round To Nearest(number=w1910) -> (nearest integer value=w1909:dbl)
              n1116 = Round To Nearest(number=w1906) -> (nearest integer value=w1905:dbl)
              n1117 = Round To Nearest(number=w1901) -> (nearest integer value=w1900:dbl)
              n1118 = Round To Nearest(number=w1896) -> (nearest integer value=w1895:dbl)
              n1119 = Round To Nearest(number=w1891) -> (nearest integer value=w1890:dbl)
              n1120 = Round To Nearest(number=w1883) -> (nearest integer value=w1882:dbl)
              n1121 = Round To Nearest(number=w1881) -> (nearest integer value=w1880:dbl)
              n1122 = To Unsigned Word Integer(number=w1909) -> (unsigned 16bit integer=w1908:u16)
              n1123 = To Unsigned Word Integer(number=w1905) -> (unsigned 16bit integer=w1903:u16)
              n1124 = To Unsigned Word Integer(number=w1900) -> (unsigned 16bit integer=w1898:u16)
              n1125 = To Unsigned Word Integer(number=w1895) -> (unsigned 16bit integer=w1893:u16)
              n1126 = To Unsigned Word Integer(number=w1890) -> (unsigned 16bit integer=w1888:u16)
              n1127 = To Unsigned Word Integer(number=w1882) -> (unsigned 16bit integer=w1876:u16)
              n1128 = To Unsigned Word Integer(number=w1880) -> (unsigned 16bit integer=w1875:u16)
              n1129 = local read "Laser_duration_l1"() -> (w1886:u16)
              n1130 = Replace Array Subset(array=w1928, new element #1=w1926, index #1=w1927, new element #2=w1924, index #2=w1925, new element #3=w1920, index #3=w1922, new element #4=w1919, index #4=w1921, new element #5=w1908, index #5=w1912, new element #6=w1903, index #6=w1907, new element #7=w1898, index #7=w1902, new element #8=w1893, index #8=w1897, new element #9=w1888, index #9=w1892, new element #10=w1876, index #10=w1885, new element #11=w1875, index #11=w1884, new element #12=w1886, index #12=w1887) -> (w1923:u16[])
            }
            frame "saveSettings4" {
              w1948 = 100.0 ("y")
              n1131 = call "myRIO_BRig_RT_dataExp_laser2_Freq.vi"() -> ("output_laser2_Freq"=w1937:i32)  [unwired: 11 in]
              n1132 = call "myRIO_BRig_RT_dataExp_laser2_Tpeak.vi"() -> ("output_laser2_Tpeak"=w1939:i32)  [unwired: 11 in]
              n1133 = call "myRIO_BRig_RT_dataExp_laser2_Tshutter.vi"() -> ("output_laser2_Tshutter"=w1941:i32)  [unwired: 11 in]
              n1134 = call "myRIO_BRig_RT_dataExp_laser2_Power_min.vi"() -> ("output_laser2_Power_min"=w1956:i32)  [unwired: 11 in]
              n1135 = call "myRIO_BRig_RT_dataExp_laser2_Power_max.vi"() -> ("output_laser2_Power_max"=w1955:i32)  [unwired: 11 in]
              n1136 = call "myRIO_BRig_RT_dataExp_laser2_Power_step.vi"() -> ("output_laser2_Power_step"=w1954:i32)  [unwired: 11 in]
              n1137 = call "myRIO_BRig_RT_dataExp_laser2_duration.vi"() -> ("output_laser2_duration"=w1953:i32)  [unwired: 11 in]
              n1138 = call "myRIO_BRig_RT_dataExp_CueLed_Freq.vi"() -> ("output_CueLed_Freq"=w1945:i32)  [unwired: 11 in]
              n1139 = call "myRIO_BRig_RT_dataExp_CueLed_Tpeak.vi"() -> ("output_CueLed_Tpeak"=w1944:i32)  [unwired: 11 in]
              n1140 = local read "Laser_Tshutter_l2"() -> (w1971:dbl)
              n1141 = local read "Laser_Tpeak_l2"() -> (w1974:dbl)
              n1142 = local read "Laser_power_max_l2"() -> (w1961:dbl)
              n1143 = local read "Laser_power_step_l2"() -> (w1960:dbl)
              n1144 = local read "Laser_power_min_l2"() -> (w1968:dbl)
              n1145 = local read "Laser_Freq_l2"() -> (w1979:dbl)
              n1146 = local read "CueLed_Tpeak"() -> (w1946:dbl)
              n1147 = local read "CueLed_Freq"() -> (w1947:dbl)
              n1148 = Multiply(x=w1979, y=w1948) -> (x*y=w1978:dbl)
              n1149 = Multiply(x=w1974, y=w1948) -> (x*y=w1976:dbl)
              n1150 = Multiply(x=w1971, y=w1948) -> (x*y=w1973:dbl)
              n1151 = Multiply(x=w1968, y=w1948) -> (x*y=w1970:dbl)
              n1152 = Multiply(x=w1961, y=w1948) -> (x*y=w1965:dbl)
              n1153 = Multiply(x=w1960, y=w1948) -> (x*y=w1963:dbl)
              n1154 = Multiply(x=w1947, y=w1948) -> (x*y=w1949:dbl)
              n1155 = Multiply(x=w1946, y=w1948) -> (x*y=w1950:dbl)
              n1156 = Round To Nearest(number=w1978) -> (nearest integer value=w1977:dbl)
              n1157 = Round To Nearest(number=w1976) -> (nearest integer value=w1975:dbl)
              n1158 = Round To Nearest(number=w1973) -> (nearest integer value=w1972:dbl)
              n1159 = Round To Nearest(number=w1970) -> (nearest integer value=w1969:dbl)
              n1160 = Round To Nearest(number=w1965) -> (nearest integer value=w1964:dbl)
              n1161 = Round To Nearest(number=w1963) -> (nearest integer value=w1962:dbl)
              n1162 = Round To Nearest(number=w1949) -> (nearest integer value=w1952:dbl)
              n1163 = Round To Nearest(number=w1950) -> (nearest integer value=w1951:dbl)
              n1164 = To Unsigned Word Integer(number=w1977) -> (unsigned 16bit integer=w1936:u16)
              n1165 = To Unsigned Word Integer(number=w1975) -> (unsigned 16bit integer=w1938:u16)
              n1166 = To Unsigned Word Integer(number=w1972) -> (unsigned 16bit integer=w1940:u16)
              n1167 = To Unsigned Word Integer(number=w1969) -> (unsigned 16bit integer=w1967:u16)
              n1168 = To Unsigned Word Integer(number=w1964) -> (unsigned 16bit integer=w1959:u16)
              n1169 = To Unsigned Word Integer(number=w1962) -> (unsigned 16bit integer=w1958:u16)
              n1170 = To Unsigned Word Integer(number=w1952) -> (unsigned 16bit integer=w1943:u16)
              n1171 = To Unsigned Word Integer(number=w1951) -> (unsigned 16bit integer=w1942:u16)
              n1172 = local read "Laser_duration_l2"() -> (w1966:u16)
              n1173 = Replace Array Subset(array=w1987, new element #1=w1936, index #1=w1937, new element #2=w1938, index #2=w1939, new element #3=w1940, index #3=w1941, new element #4=w1967, index #4=w1956, new element #5=w1959, index #5=w1955, new element #6=w1958, index #6=w1954, new element #7=w1966, index #7=w1953, new element #8=w1943, index #8=w1945, new element #9=w1942, index #9=w1944) -> (w1986:u16[])
            }
            frame "saveSettings_LC_ENL_l1" {
              # "Selection First"
              # "Count"
              # "Tdelay"
              # "Probability"
              # "OnOff"
              # "Block"
              # "delayOpt"
              # "Count"
              # "Tdelay"
              # "Probability"
              # "OnOff"
              # "Block"
              # "ENL1 All"
              # "delayOpt"
              # "Count"
              # "Tdelay"
              # "Probability"
              # "OnOff"
              # "Block"
              # "ENL1 First"
              n1174 = local read "LC_ENL1_delayOpt_Switch_l1"() -> (w2025:bool)
              n1175 = call "myRIO_BRig_RT_dataLC_ENL1_Block_NS_l1.vi"() -> ("output_ENL1_All_Block"=w2022:i32)  [unwired: 11 in]
              n1176 = call "myRIO_BRig_RT_dataLC_ENL1_OnOff_NS_l1.vi"() -> ("output_ENL1_OnOff_NS_l1"=w2012:i32)  [unwired: 11 in]
              n1177 = call "myRIO_BRig_RT_dataLC_ENL1_Probability_NS_l1.vi"() -> ("output_ENL1_Probability_NS_l1"=w2011:i32)  [unwired: 11 in]
              n1178 = call "myRIO_BRig_RT_dataLC_ENL1_Tdelay_NS_l1.vi"() -> ("output_ENL1_Tdelay_NS_l1"=w2010:i32)  [unwired: 11 in]
              n1179 = call "myRIO_BRig_RT_dataLC_ENL1_Count_NS_l1.vi"() -> ("output_ENL1_Count_NS_l1"=w2009:i32)  [unwired: 11 in]
              n1180 = call "myRIO_BRig_RT_dataLC_ENL1_delayOpt_NS_l1.vi"() -> ("output_ENL1_delayOpt_NS_l1"=w2008:i32)  [unwired: 11 in]
              n1181 = call "myRIO_BRig_RT_dataLC_ENL1_Block_Switch_l1.vi"() -> ("output_ENL1_Block_Switch_l1"=w2044:i32)  [unwired: 11 in]
              n1182 = call "myRIO_BRig_RT_dataLC_ENL1_OnOff_Switch_l1.vi"() -> ("output_ENL1_OnOff_Switch_l1"=w2042:i32)  [unwired: 11 in]
              n1183 = call "myRIO_BRig_RT_dataLC_ENL1_Probability_Switch_l1.vi"() -> ("output_ENL1_Probability_Switch_l1"=w2038:i32)  [unwired: 11 in]
              n1184 = call "myRIO_BRig_RT_dataLC_ENL1_Tdelay_Switch_l1.vi"() -> ("output_ENL1_Tdelay_Switch_l1"=w2036:i32)  [unwired: 11 in]
              n1185 = call "myRIO_BRig_RT_dataLC_ENL1_Count_Switch_l1.vi"() -> ("output_ENL1_Count_Switch_l1"=w2034:i32)  [unwired: 11 in]
              n1186 = call "myRIO_BRig_RT_dataLC_ENL1_delayOpt_Switch_l1.vi"() -> ("output_ENL1_delayOpt_Switch_l1"=w2024:i32)  [unwired: 11 in]
              n1187 = local read "LC_ENL1_Count_Switch_l1"() -> (w2033:u16)
              n1188 = local read "LC_ENL1_Probability_Switch_l1"() -> (w2037:u16)
              n1189 = local read "LC_ENL1_Block_Switch_l1"() -> (w2043:u16)
              n1190 = local read "LC_ENL1_Tdelay_Switch_l1"() -> (w2035:u16)
              n1191 = local read "LC_ENL1_OnOff_Switch_l1"() -> (w2041:bool)
              n1192 = call "myRIO_BRig_RT_dataLC_Selection_Block_Switch_l1.vi"() -> ("output_Selection_Block_Switch_l1"=w2006:i32)  [unwired: 11 in]
              n1193 = call "myRIO_BRig_RT_dataLC_Selection_OnOff_Switch_l1.vi"() -> ("output_Selection_OnOff_Switch_l1"=w2005:i32)  [unwired: 11 in]
              n1194 = call "myRIO_BRig_RT_dataLC_Selection_Probability_Switch_l1.vi"() -> ("output_Selection_Probability_Switch_l1"=w2004:i32)  [unwired: 11 in]
              n1195 = call "myRIO_BRig_RT_dataLC_Selection_Tdelay_Switch_l1.vi"() -> ("output_Selection_Tdelay_Switch_l1"=w2003:i32)  [unwired: 11 in]
              n1196 = call "myRIO_BRig_RT_dataLC_Selection_Count_Switch_l1.vi"() -> ("output_Selection_Count_Switch_l1"=w2002:i32)  [unwired: 11 in]
              n1197 = local read "LC_ENL1_OnOff_NS_l1"() -> (w2018:bool)
              n1198 = local read "LC_ENL1_Probability_NS_l1"() -> (w2016:u16)
              n1199 = local read "LC_ENL1_delayOpt_NS_l1"() -> (w2014:bool)
              n1200 = local read "LC_Sel_Probability_Switch_l1"() -> (w1997:u16)
              n1201 = local read "LC_ENL1_Tdelay_NS_l1"() -> (w2007:u16)
              n1202 = local read "LC_ENL1_Block_NS_l1"() -> (w2019:u16)
              n1203 = local read "LC_ENL1_Count_NS_l1"() -> (w2015:u16)
              n1204 = local read "LC_Sel_Tdelay_Switch_l1"() -> (w1996:u16)
              n1205 = local read "LC_Sel_OnOff_Switch_l1"() -> (w2000:bool)
              n1206 = local read "LC_Sel_Count_Switch_l1"() -> (w1995:u16)
              n1207 = local read "LC_Sel_Block_Switch_l1"() -> (w1999:u16)
              n1208 = Boolean To (0,1)(Boolean=w2025) -> (0, 1=w2026:i16)
              n1209 = Boolean To (0,1)(Boolean=w2041) -> (0, 1=w2040:i16)
              n1210 = Boolean To (0,1)(Boolean=w2018) -> (0, 1=w2021:i16)
              n1211 = To Unsigned Word Integer(number=w2026) -> (unsigned 16bit integer=w2023:u16)
              n1212 = To Unsigned Word Integer(number=w2040) -> (unsigned 16bit integer=w2039:u16)
              n1213 = Boolean To (0,1)(Boolean=w2014) -> (0, 1=w2020:i16)
              n1214 = To Unsigned Word Integer(number=w2021) -> (unsigned 16bit integer=w2017:u16)
              n1215 = Boolean To (0,1)(Boolean=w2000) -> (0, 1=w2001:i16)
              n1216 = To Unsigned Word Integer(number=w2020) -> (unsigned 16bit integer=w2013:u16)
              n1217 = To Unsigned Word Integer(number=w2001) -> (unsigned 16bit integer=w1998:u16)
              n1218 = Replace Array Subset(array=w2045, new element #1=w2043, index #1=w2044, new element #2=w2039, index #2=w2042, new element #3=w2037, index #3=w2038, new element #4=w2035, index #4=w2036, new element #5=w2033, index #5=w2034, new element #6=w2023, index #6=w2024, new element #7=w2019, index #7=w2022, new element #8=w2017, index #8=w2012, new element #9=w2016, index #9=w2011, new element #10=w2007, index #10=w2010, new element #11=w2015, index #11=w2009, new element #12=w2013, index #12=w2008, new element #13=w1999, index #13=w2006, new element #14=w1998, index #14=w2005, new element #15=w1997, index #15=w2004, new element #16=w1996, index #16=w2003, new element #17=w1995, index #17=w2002) -> (w2046:u16[])
            }
            frame "saveSettings_LC_ENL_l2" {
              # "Selection First"
              # "Count"
              # "Tdelay"
              # "Probability"
              # "OnOff"
              # "Block"
              # "delayOpt"
              # "Count"
              # "Tdelay"
              # "Probability"
              # "OnOff"
              # "Block"
              # "ENL1 All"
              # "delayOpt"
              # "Count"
              # "Tdelay"
              # "Probability"
              # "OnOff"
              # "Block"
              # "ENL1 First"
              n1219 = call "myRIO_BRig_RT_dataLC_ENL1_Block_Switch_l2.vi"() -> ("output_ENL1_Block_Switch_l2"=w2065:i32)  [unwired: 11 in]
              n1220 = call "myRIO_BRig_RT_dataLC_ENL1_OnOff_Switch_l2.vi"() -> ("output_ENL1_OnOff_Switch_l2"=w2066:i32)  [unwired: 11 in]
              n1221 = call "myRIO_BRig_RT_dataLC_ENL1_Probability_Switch_l2.vi"() -> ("output_ENL1_Probability_Switch_l2"=w2067:i32)  [unwired: 11 in]
              n1222 = call "myRIO_BRig_RT_dataLC_ENL1_Tdelay_Switch_l2.vi"() -> ("output_ENL1_Tdelay_Switch_l2"=w2068:i32)  [unwired: 11 in]
              n1223 = call "myRIO_BRig_RT_dataLC_ENL1_Count_Switch_l2.vi"() -> ("output_ENL1_Count_Switch_l2"=w2069:i32)  [unwired: 11 in]
              n1224 = call "myRIO_BRig_RT_dataLC_ENL1_delayOpt_Switch_l2.vi"() -> ("output_ENL1_delayOpt_Switch_l2"=w2070:i32)  [unwired: 11 in]
              n1225 = local read "LC_ENL1_delayOpt_Switch_l2"() -> (w2090:bool)
              n1226 = call "myRIO_BRig_RT_dataLC_ENL1_Block_NS_l2.vi"() -> ("output_ENL1_Block_NS_l2"=w2059:i32)  [unwired: 11 in]
              n1227 = call "myRIO_BRig_RT_dataLC_ENL1_OnOff_NS_l2.vi"() -> ("output_ENL1_OnOff_NS_l2"=w2060:i32)  [unwired: 11 in]
              n1228 = call "myRIO_BRig_RT_dataLC_ENL1_Probability_NS_l2.vi"() -> ("output_ENL1_Probability_NS_l2"=w2061:i32)  [unwired: 11 in]
              n1229 = call "myRIO_BRig_RT_dataLC_ENL1_Tdelay_NS_l2.vi"() -> ("output_ENL1_Tdelay_NS_l2"=w2062:i32)  [unwired: 11 in]
              n1230 = call "myRIO_BRig_RT_dataLC_ENL1_Count_NS_l2.vi"() -> ("output_ENL1_Count_NS_l2"=w2063:i32)  [unwired: 11 in]
              n1231 = call "myRIO_BRig_RT_dataLC_ENL1_delayOpt_NS_l2.vi"() -> ("output_ENL1_delayOpt_NS_l2"=w2064:i32)  [unwired: 11 in]
              n1232 = local read "LC_ENL1_Count_Switch_l2"() -> (w2098:u16)
              n1233 = local read "LC_ENL1_Probability_Switch_l2"() -> (w2100:u16)
              n1234 = local read "LC_ENL1_Block_Switch_l2"() -> (w2104:u16)
              n1235 = local read "LC_ENL1_Tdelay_Switch_l2"() -> (w2099:u16)
              n1236 = local read "LC_ENL1_OnOff_Switch_l2"() -> (w2103:bool)
              n1237 = call "myRIO_BRig_RT_dataLC_Selection_Block_Switch_l2.vi"() -> ("output_Selection_Block_Switch_l2"=w2058:i32)  [unwired: 11 in]
              n1238 = call "myRIO_BRig_RT_dataLC_Selection_OnOff_Switch_l2.vi"() -> ("output_Selection_OnOff_Switch_l2"=w2057:i32)  [unwired: 11 in]
              n1239 = call "myRIO_BRig_RT_dataLC_Selection_Probability_Switch_l2.vi"() -> ("output_Selection_Probability_Switch_l1"=w2056:i32)  [unwired: 11 in]
              n1240 = call "myRIO_BRig_RT_dataLC_Selection_Tdelay_Switch_l2.vi"() -> ("output_Selection_Tdelay_Switch_l2"=w2055:i32)  [unwired: 11 in]
              n1241 = call "myRIO_BRig_RT_dataLC_Selection_Count_Switch_l2.vi"() -> ("output_Selection_Count_Switch_l2"=w2054:i32)  [unwired: 11 in]
              n1242 = local read "LC_ENL1_OnOff_NS_l2"() -> (w2085:bool)
              n1243 = local read "LC_ENL1_Probability_NS_l2"() -> (w2083:u16)
              n1244 = local read "LC_ENL1_delayOpt_NS_l2"() -> (w2081:bool)
              n1245 = local read "LC_Sel_Probability_Switch_l2"() -> (w2074:u16)
              n1246 = local read "LC_ENL1_Tdelay_NS_l2"() -> (w2079:u16)
              n1247 = local read "LC_ENL1_Block_NS_l2"() -> (w2086:u16)
              n1248 = local read "LC_ENL1_Count_NS_l2"() -> (w2082:u16)
              n1249 = local read "LC_Sel_Tdelay_Switch_l2"() -> (w2073:u16)
              n1250 = local read "LC_Sel_OnOff_Switch_l2"() -> (w2077:bool)
              n1251 = local read "LC_Sel_Count_Switch_l2"() -> (w2072:u16)
              n1252 = local read "LC_Sel_Block_Switch_l2"() -> (w2076:u16)
              n1253 = Boolean To (0,1)(Boolean=w2090) -> (0, 1=w2091:i16)
              n1254 = Boolean To (0,1)(Boolean=w2103) -> (0, 1=w2102:i16)
              n1255 = Boolean To (0,1)(Boolean=w2085) -> (0, 1=w2088:i16)
              n1256 = To Unsigned Word Integer(number=w2091) -> (unsigned 16bit integer=w2089:u16)
              n1257 = To Unsigned Word Integer(number=w2102) -> (unsigned 16bit integer=w2101:u16)
              n1258 = Boolean To (0,1)(Boolean=w2081) -> (0, 1=w2087:i16)
              n1259 = To Unsigned Word Integer(number=w2088) -> (unsigned 16bit integer=w2084:u16)
              n1260 = Boolean To (0,1)(Boolean=w2077) -> (0, 1=w2078:i16)
              n1261 = To Unsigned Word Integer(number=w2087) -> (unsigned 16bit integer=w2080:u16)
              n1262 = To Unsigned Word Integer(number=w2078) -> (unsigned 16bit integer=w2075:u16)
              n1263 = Replace Array Subset(array=w2105, new element #1=w2104, index #1=w2065, new element #2=w2101, index #2=w2066, new element #3=w2100, index #3=w2067, new element #4=w2099, index #4=w2068, new element #5=w2098, index #5=w2069, new element #6=w2089, index #6=w2070, new element #7=w2086, index #7=w2059, new element #8=w2084, index #8=w2060, new element #9=w2083, index #9=w2061, new element #10=w2079, index #10=w2062, new element #11=w2082, index #11=w2063, new element #12=w2080, index #12=w2064, new element #13=w2076, index #13=w2058, new element #14=w2075, index #14=w2057, new element #15=w2074, index #15=w2056, new element #16=w2073, index #16=w2055, new element #17=w2072, index #17=w2054) -> (w2106:u16[])
            }
            frame "saveSettings_LC_Cue_l1" {
              # "Selection All"
              # "Count"
              # "Tdelay"
              # "Probability"
              # "OnOff"
              # "Block"
              # "delayOpt"
              # "Count"
              # "Tdelay"
              # "Probability"
              # "OnOff"
              # "Block"
              # "Cue1 All"
              # "delayOpt"
              # "Count"
              # "Tdelay"
              # "Probability"
              # "OnOff"
              # "Block"
              # "Cue1 First"
              n1264 = call "myRIO_BRig_RT_dataLC_Cue1_delayOpt_Switch_l1.vi"() -> ("output_Cue1_delayOpt_Switch_l1"=w2145:i32)  [unwired: 11 in]
              n1265 = call "myRIO_BRig_RT_dataLC_Cue1_Block_Switch_l1.vi"() -> ("output_Cue1_Block_Switch_l1"=w2164:i32)  [unwired: 11 in]
              n1266 = call "myRIO_BRig_RT_dataLC_Cue1_OnOff_Switch_l1.vi"() -> ("output_Cue1_OnOff_Switch_l1"=w2162:i32)  [unwired: 11 in]
              n1267 = call "myRIO_BRig_RT_dataLC_Cue1_Probability_Switch_l1.vi"() -> ("output_Cue1_Probability_Switch_l1"=w2158:i32)  [unwired: 11 in]
              n1268 = call "myRIO_BRig_RT_dataLC_Cue1_Tdelay_Switch_l1.vi"() -> ("output_Cue1_Tdelay_Switch_l1"=w2156:i32)  [unwired: 11 in]
              n1269 = call "myRIO_BRig_RT_dataLC_Cue1_Count_Switch_l1.vi"() -> ("output_Cue1_Count_Switch_l1"=w2154:i32)  [unwired: 11 in]
              n1270 = local read "LC_Cue1_delayOpt_Switch_l1"() -> (w2144:bool)
              n1271 = call "myRIO_BRig_RT_dataLC_Cue1_Block_NS_l1.vi"() -> ("output_Cue1_Block_NS_l1"=w2142:i32)  [unwired: 11 in]
              n1272 = call "myRIO_BRig_RT_dataLC_Cue1_OnOff_NS_l1.vi"() -> ("output_Cue1_OnOff_NS_l1"=w2141:i32)  [unwired: 11 in]
              n1273 = call "myRIO_BRig_RT_dataLC_Cue1_Probability_NS_l1.vi"() -> ("output_Cue1_l1_All_Probability"=w2140:i32)  [unwired: 11 in]
              n1274 = call "myRIO_BRig_RT_dataLC_Cue1_Tdelay_NS_l1.vi"() -> ("output_Cue1_Tdelay_NS_l1"=w2139:i32)  [unwired: 11 in]
              n1275 = call "myRIO_BRig_RT_dataLC_Cue1_Count_NS_l1.vi"() -> ("output_Cue1_Count_NS_l1"=w2138:i32)  [unwired: 11 in]
              n1276 = call "myRIO_BRig_RT_dataLC_Cue1_delayOpt_NS_l1.vi"() -> ("output_Cue1_delayOpt_NS_l1"=w2137:i32)  [unwired: 11 in]
              n1277 = local read "LC_Cue1_Count_Switch_l1"() -> (w2153:u16)
              n1278 = local read "LC_Cue1_Probability_Switch_l1"() -> (w2157:u16)
              n1279 = local read "LC_Cue1_Block_Switch_l1"() -> (w2163:u16)
              n1280 = local read "LC_Cue1_Tdelay_Switch_l1"() -> (w2155:u16)
              n1281 = local read "LC_Cue1_OnOff_Switch_l1"() -> (w2161:bool)
              n1282 = local read "LC_Cue1_OnOff_NS_l1"() -> (w2133:bool)
              n1283 = call "myRIO_BRig_RT_dataLC_Selection_Block_NS_l1.vi"() -> ("output_Selection_Block_NS_l1"=w2126:i32)  [unwired: 11 in]
              n1284 = call "myRIO_BRig_RT_dataLC_Selection_OnOff_NS_l1.vi"() -> ("output_Selection_OnOff_NS_l1"=w2125:i32)  [unwired: 11 in]
              n1285 = call "myRIO_BRig_RT_dataLC_Selection_Probability_NS_l1.vi"() -> ("output_Selection_Probability_NS_l1"=w2124:i32)  [unwired: 11 in]
              n1286 = call "myRIO_BRig_RT_dataLC_Selection_Tdelay_NS_l1.vi"() -> ("output_Selection_Tdelay_NS_l1"=w2123:i32)  [unwired: 11 in]
              n1287 = call "myRIO_BRig_RT_dataLC_Selection_Count_NS_l1.vi"() -> ("output_Selection_Count_NS_l1"=w2116:i32)  [unwired: 11 in]
              n1288 = local read "LC_Cue1_delayOpt_NS_l1"() -> (w2134:bool)
              n1289 = local read "LC_Cue1_Probability_NS_l1"() -> (w2130:u16)
              n1290 = local read "LC_Cue1_Tdelay_NS_l1"() -> (w2129:u16)
              n1291 = local read "LC_Cue1_Count_NS_l1"() -> (w2128:u16)
              n1292 = local read "LC_Cue1_Block_NS_l1"() -> (w2132:u16)
              n1293 = local read "LC_Sel_Probability_NS_l1"() -> (w2118:u16)
              n1294 = local read "LC_Sel_Tdelay_NS_l1"() -> (w2117:u16)
              n1295 = local read "LC_Sel_OnOff_NS_l1"() -> (w2120:bool)
              n1296 = local read "LC_Sel_Count_NS_l1"() -> (w2115:u16)
              n1297 = local read "LC_Sel_Block_NS_l1"() -> (w2122:u16)
              n1298 = Boolean To (0,1)(Boolean=w2144) -> (0, 1=w2146:i16)
              n1299 = Boolean To (0,1)(Boolean=w2161) -> (0, 1=w2160:i16)
              n1300 = Boolean To (0,1)(Boolean=w2133) -> (0, 1=w2136:i16)
              n1301 = To Unsigned Word Integer(number=w2146) -> (unsigned 16bit integer=w2143:u16)
              n1302 = To Unsigned Word Integer(number=w2160) -> (unsigned 16bit integer=w2159:u16)
              n1303 = To Unsigned Word Integer(number=w2136) -> (unsigned 16bit integer=w2131:u16)
              n1304 = Boolean To (0,1)(Boolean=w2134) -> (0, 1=w2135:i16)
              n1305 = Boolean To (0,1)(Boolean=w2120) -> (0, 1=w2121:i16)
              n1306 = To Unsigned Word Integer(number=w2135) -> (unsigned 16bit integer=w2127:u16)
              n1307 = To Unsigned Word Integer(number=w2121) -> (unsigned 16bit integer=w2119:u16)
              n1308 = Replace Array Subset(array=w2165, new element #1=w2163, index #1=w2164, new element #2=w2159, index #2=w2162, new element #3=w2157, index #3=w2158, new element #4=w2155, index #4=w2156, new element #5=w2153, index #5=w2154, new element #6=w2143, index #6=w2145, new element #7=w2132, index #7=w2142, new element #8=w2131, index #8=w2141, new element #9=w2130, index #9=w2140, new element #10=w2129, index #10=w2139, new element #11=w2128, index #11=w2138, new element #12=w2127, index #12=w2137, new element #13=w2122, index #13=w2126, new element #14=w2119, index #14=w2125, new element #15=w2118, index #15=w2124, new element #16=w2117, index #16=w2123, new element #17=w2115, index #17=w2116) -> (w2166:u16[])
            }
            frame "saveSettings_LC_Cue_l2" {
              # "Selection All"
              # "Count"
              # "Tdelay"
              # "Probability"
              # "OnOff"
              # "Block"
              # "delayOpt"
              # "Count"
              # "Tdelay"
              # "Probability"
              # "OnOff"
              # "Block"
              # "Cue1 All"
              # "delayOpt"
              # "Count"
              # "Tdelay"
              # "Probability"
              # "OnOff"
              # "Block"
              # "Cue1 First"
              n1309 = call "myRIO_BRig_RT_dataLC_Cue1_delayOpt_Switch_l2.vi"() -> ("output_Cue1_delayOpt_Switch_l2"=w2205:i32)  [unwired: 11 in]
              n1310 = call "myRIO_BRig_RT_dataLC_Cue1_Block_Switch_l2.vi"() -> ("output_Cue1_Block_Switch_l2"=w2224:i32)  [unwired: 11 in]
              n1311 = call "myRIO_BRig_RT_dataLC_Cue1_OnOff_Switch_l2.vi"() -> ("output_Cue1_OnOff_Switch_l2"=w2222:i32)  [unwired: 11 in]
              n1312 = call "myRIO_BRig_RT_dataLC_Cue1_Probability_Switch_l2.vi"() -> ("output_Cue1_l2_First_Probability"=w2218:i32)  [unwired: 11 in]
              n1313 = call "myRIO_BRig_RT_dataLC_Cue1_Tdelay_Switch_l2.vi"() -> ("output_Cue1_Tdelay_Switch_l2"=w2216:i32)  [unwired: 11 in]
              n1314 = call "myRIO_BRig_RT_dataLC_Cue1_Count_Switch_l2.vi"() -> ("output_Cue1_Count_Switch_l2"=w2214:i32)  [unwired: 11 in]
              n1315 = local read "LC_Cue1_delayOpt_Switch_l2"() -> (w2204:bool)
              n1316 = call "myRIO_BRig_RT_dataLC_Cue1_Block_NS_l2.vi"() -> ("output_Cue1_Block_NS_l2"=w2202:i32)  [unwired: 11 in]
              n1317 = call "myRIO_BRig_RT_dataLC_Cue1_OnOff_NS_l2.vi"() -> ("output_Cue1_OnOff_NS_l2"=w2201:i32)  [unwired: 11 in]
              n1318 = call "myRIO_BRig_RT_dataLC_Cue1_Probability_NS_l2.vi"() -> ("output_Cue1_l2_All_Probability"=w2200:i32)  [unwired: 11 in]
              n1319 = call "myRIO_BRig_RT_dataLC_Cue1_Tdelay_NS_l2.vi"() -> ("output_Cue1_Tdelay_NS_l2"=w2199:i32)  [unwired: 11 in]
              n1320 = call "myRIO_BRig_RT_dataLC_Cue1_Count_NS_l2.vi"() -> ("output_Cue1_Count_NS_l2"=w2198:i32)  [unwired: 11 in]
              n1321 = call "myRIO_BRig_RT_dataLC_Cue1_delayOpt_NS_l2.vi"() -> ("output_Cue1_delayOpt_NS_l2"=w2197:i32)  [unwired: 11 in]
              n1322 = local read "LC_Cue1_Count_Switch_l2"() -> (w2213:u16)
              n1323 = local read "LC_Cue1_Probability_Switch_l2"() -> (w2217:u16)
              n1324 = local read "LC_Cue1_Block_Switch_l2"() -> (w2223:u16)
              n1325 = local read "LC_Cue1_Tdelay_Switch_l2"() -> (w2215:u16)
              n1326 = local read "LC_Cue1_OnOff_Switch_l2"() -> (w2221:bool)
              n1327 = local read "LC_Cue1_OnOff_NS_l2"() -> (w2193:bool)
              n1328 = call "myRIO_BRig_RT_dataLC_Selection_Block_NS_l2.vi"() -> ("output_Selection_Block_NS_l2"=w2178:i32)  [unwired: 11 in]
              n1329 = call "myRIO_BRig_RT_dataLC_Selection_OnOff_NS_l2.vi"() -> ("output_Selection_OnOff_NS_l2"=w2177:i32)  [unwired: 11 in]
              n1330 = call "myRIO_BRig_RT_dataLC_Selection_Probability_NS_l2.vi"() -> ("output_Selection_Probability_NS_l2"=w2176:i32)  [unwired: 11 in]
              n1331 = call "myRIO_BRig_RT_dataLC_Selection_Tdelay_NS_l2.vi"() -> ("output_Selection_Tdelay_NS_l2"=w2175:i32)  [unwired: 11 in]
              n1332 = call "myRIO_BRig_RT_dataLC_Selection_Count_NS_l2.vi"() -> ("output_Selection_Count_NS_l2"=w2174:i32)  [unwired: 11 in]
              n1333 = local read "LC_Cue1_delayOpt_NS_l2"() -> (w2194:bool)
              n1334 = local read "LC_Cue1_Probability_NS_l2"() -> (w2190:u16)
              n1335 = local read "LC_Cue1_Tdelay_NS_l2"() -> (w2189:u16)
              n1336 = local read "LC_Cue1_Count_NS_l2"() -> (w2188:u16)
              n1337 = local read "LC_Cue1_Block_NS_l2"() -> (w2192:u16)
              n1338 = local read "LC_Sel_Probability_NS_l2"() -> (w2182:u16)
              n1339 = local read "LC_Sel_Tdelay_NS_l2"() -> (w2181:u16)
              n1340 = local read "LC_Sel_OnOff_NS_l2"() -> (w2184:bool)
              n1341 = local read "LC_Sel_Count_NS_l2"() -> (w2180:u16)
              n1342 = local read "LC_Sel_Block_NS_l2"() -> (w2186:u16)
              n1343 = Boolean To (0,1)(Boolean=w2204) -> (0, 1=w2206:i16)
              n1344 = Boolean To (0,1)(Boolean=w2221) -> (0, 1=w2220:i16)
              n1345 = Boolean To (0,1)(Boolean=w2193) -> (0, 1=w2196:i16)
              n1346 = To Unsigned Word Integer(number=w2206) -> (unsigned 16bit integer=w2203:u16)
              n1347 = To Unsigned Word Integer(number=w2220) -> (unsigned 16bit integer=w2219:u16)
              n1348 = To Unsigned Word Integer(number=w2196) -> (unsigned 16bit integer=w2191:u16)
              n1349 = Boolean To (0,1)(Boolean=w2194) -> (0, 1=w2195:i16)
              n1350 = Boolean To (0,1)(Boolean=w2184) -> (0, 1=w2185:i16)
              n1351 = To Unsigned Word Integer(number=w2195) -> (unsigned 16bit integer=w2187:u16)
              n1352 = To Unsigned Word Integer(number=w2185) -> (unsigned 16bit integer=w2183:u16)
              n1353 = Replace Array Subset(array=w2225, new element #1=w2223, index #1=w2224, new element #2=w2219, index #2=w2222, new element #3=w2217, index #3=w2218, new element #4=w2215, index #4=w2216, new element #5=w2213, index #5=w2214, new element #6=w2203, index #6=w2205, new element #7=w2192, index #7=w2202, new element #8=w2191, index #8=w2201, new element #9=w2190, index #9=w2200, new element #10=w2189, index #10=w2199, new element #11=w2188, index #11=w2198, new element #12=w2187, index #12=w2197, new element #13=w2186, index #13=w2178, new element #14=w2183, index #14=w2177, new element #15=w2182, index #15=w2176, new element #16=w2181, index #16=w2175, new element #17=w2180, index #17=w2174) -> (w2226:u16[])
            }
            frame "saveSettings6_LC_l1_Other" {
              # "Trial"
              # "Tdelay"
              # "Probability"
              # "OnOff"
              # "Block"
              # "Wrong"
              # "Trial"
              # "Tdelay"
              # "Probability"
              # "OnOff"
              # "Block"
              # "Reward"
              n1354 = call "myRIO_BRig_RT_dataLC_Wrong_Block_l1.vi"() -> ("output_Wrong_Block_l1"=w2251:i32)  [unwired: 11 in]
              n1355 = call "myRIO_BRig_RT_dataLC_Wrong_OnOff_l1.vi"() -> ("output_Wrong_OnOff_l1"=w2250:i32)  [unwired: 11 in]
              n1356 = call "myRIO_BRig_RT_dataLC_Wrong_Probability_l1.vi"() -> ("output_Wrong_Probability_l1"=w2249:i32)  [unwired: 11 in]
              n1357 = call "myRIO_BRig_RT_dataLC_Wrong_Tdelay_l1.vi"() -> ("output_Wrong_Tdelay_l1"=w2248:i32)  [unwired: 11 in]
              n1358 = call "myRIO_BRig_RT_dataLC_Wrong_Trial_l1.vi"() -> ("output_Wrong_Trial_l1"=w2247:i32)  [unwired: 11 in]
              n1359 = call "myRIO_BRig_RT_dataLC_Reward_Block_l1.vi"() -> ("output_Reward_Block_l1"=w2263:i32)  [unwired: 11 in]
              n1360 = call "myRIO_BRig_RT_dataLC_Reward_OnOff_l1.vi"() -> ("output_Reward_OnOff_l1"=w2261:i32)  [unwired: 11 in]
              n1361 = call "myRIO_BRig_RT_dataLC_Reward_Probability_l1.vi"() -> ("output_Reward_Probability_l1"=w2257:i32)  [unwired: 11 in]
              n1362 = call "myRIO_BRig_RT_dataLC_Reward_Tdelay_l1.vi"() -> ("output_Reward_Tdelay_l1"=w2255:i32)  [unwired: 11 in]
              n1363 = call "myRIO_BRig_RT_dataLC_Reward_Trial_l1.vi"() -> ("output_Reward_Trial_l1"=w2253:i32)  [unwired: 11 in]
              n1364 = local read "LC_Wrong_OnOff_l1"() -> (w2245:bool)
              n1365 = local read "LC_Wrong_Probability_l1"() -> (w2242:u16)
              n1366 = local read "LC_Wrong_Block_l1"() -> (w2244:u16)
              n1367 = local read "LC_Wrong_Tdelay_l1"() -> (w2241:u16)
              n1368 = local read "LC_Wrong_Trial_l1"() -> (w2240:u16)
              n1369 = local read "LC_Reward_Probability_l1"() -> (w2256:u16)
              n1370 = local read "LC_Reward_Block_l1"() -> (w2262:u16)
              n1371 = local read "LC_Reward_Tdelay_l1"() -> (w2254:u16)
              n1372 = local read "LC_Reward_OnOff_l1"() -> (w2260:bool)
              n1373 = local read "LC_Reward_Trial_l1"() -> (w2252:u16)
              n1374 = Boolean To (0,1)(Boolean=w2245) -> (0, 1=w2246:i16)
              n1375 = Boolean To (0,1)(Boolean=w2260) -> (0, 1=w2259:i16)
              n1376 = To Unsigned Word Integer(number=w2246) -> (unsigned 16bit integer=w2243:u16)
              n1377 = To Unsigned Word Integer(number=w2259) -> (unsigned 16bit integer=w2258:u16)
              n1378 = Replace Array Subset(array=w2264, new element #1=w2262, index #1=w2263, new element #2=w2258, index #2=w2261, new element #3=w2256, index #3=w2257, new element #4=w2254, index #4=w2255, new element #5=w2252, index #5=w2253, new element #6=w2244, index #6=w2251, new element #7=w2243, index #7=w2250, new element #8=w2242, index #8=w2249, new element #9=w2241, index #9=w2248, new element #10=w2240, index #10=w2247) -> (w2265:u16[])
            }
            frame "SaveSettings6_LC_l2_Other" {
              # "Trial"
              # "Tdelay"
              # "Probability"
              # "OnOff"
              # "Block"
              # "Wrong"
              # "Trial"
              # "Tdelay"
              # "Probability"
              # "OnOff"
              # "Block"
              # "Reward"
              n1379 = call "myRIO_BRig_RT_dataLC_Wrong_Block_l2.vi"() -> ("output_Wrong_Block_l2"=w2274:i32)  [unwired: 11 in]
              n1380 = call "myRIO_BRig_RT_dataLC_Wrong_OnOff_l2.vi"() -> ("output_Wrong_OnOff_l2"=w2275:i32)  [unwired: 11 in]
              n1381 = call "myRIO_BRig_RT_dataLC_Wrong_Probability_l2.vi"() -> ("output_Wrong_Probability_l2"=w2276:i32)  [unwired: 11 in]
              n1382 = call "myRIO_BRig_RT_dataLC_Wrong_Tdelay_l2.vi"() -> ("output_Wrong_Tdelay_l2"=w2277:i32)  [unwired: 11 in]
              n1383 = call "myRIO_BRig_RT_dataLC_Wrong_Trial_l2.vi"() -> ("output_Wrong_Trial_l2"=w2278:i32)  [unwired: 11 in]
              n1384 = call "myRIO_BRig_RT_dataLC_Reward_Block_l2.vi"() -> ("output_Reward_Block_l2"=w2279:i32)  [unwired: 11 in]
              n1385 = call "myRIO_BRig_RT_dataLC_Reward_OnOff_l2.vi"() -> ("output_Reward_OnOff_l2"=w2280:i32)  [unwired: 11 in]
              n1386 = call "myRIO_BRig_RT_dataLC_Reward_Probability_l2.vi"() -> ("output_Reward_Probability_l2"=w2281:i32)  [unwired: 11 in]
              n1387 = call "myRIO_BRig_RT_dataLC_Reward_Tdelay_l2.vi"() -> ("output_Reward_Tdelay_l2"=w2282:i32)  [unwired: 11 in]
              n1388 = call "myRIO_BRig_RT_dataLC_Reward_Trial_l2.vi"() -> ("output_Reward_Trial_l2"=w2283:i32)  [unwired: 11 in]
              n1389 = local read "LC_Wrong_OnOff_l2"() -> (w2295:bool)
              n1390 = local read "LC_Wrong_Probability_l2"() -> (w2292:u16)
              n1391 = local read "LC_Wrong_Block_l2"() -> (w2294:u16)
              n1392 = local read "LC_Wrong_Tdelay_l2"() -> (w2291:u16)
              n1393 = local read "LC_Wrong_Trial_l2"() -> (w2290:u16)
              n1394 = local read "LC_Reward_Probability_l2"() -> (w2299:u16)
              n1395 = local read "LC_Reward_Block_l2"() -> (w2303:u16)
              n1396 = local read "LC_Reward_Tdelay_l2"() -> (w2298:u16)
              n1397 = local read "LC_Reward_OnOff_l2"() -> (w2302:bool)
              n1398 = local read "LC_Reward_Trial_l2"() -> (w2297:u16)
              n1399 = Boolean To (0,1)(Boolean=w2295) -> (0, 1=w2296:i16)
              n1400 = Boolean To (0,1)(Boolean=w2302) -> (0, 1=w2301:i16)
              n1401 = To Unsigned Word Integer(number=w2296) -> (unsigned 16bit integer=w2293:u16)
              n1402 = To Unsigned Word Integer(number=w2301) -> (unsigned 16bit integer=w2300:u16)
              n1403 = Replace Array Subset(array=w2304, new element #1=w2303, index #1=w2279, new element #2=w2300, index #2=w2280, new element #3=w2299, index #3=w2281, new element #4=w2298, index #4=w2282, new element #5=w2297, index #5=w2283, new element #6=w2294, index #6=w2274, new element #7=w2293, index #7=w2275, new element #8=w2292, index #8=w2276, new element #9=w2291, index #9=w2277, new element #10=w2290, index #10=w2278) -> (w2305:u16[])
            }
            frame "setSettings_Audio" {
              # "amp_L"
              # "amp_R"
              # "freq_L"
              # "freq_R"
              n1404 = call "myRIO_BRig_RT_dataExp_Audio_amp__L.vi"() -> ("output_Audio_amp__L"=w2333:i32)  [unwired: 11 in]
              n1405 = call "myRIO_BRig_RT_dataExp_Audio_amp__R.vi"() -> ("output_Audio_amp__R"=w2332:i32)  [unwired: 11 in]
              n1406 = call "myRIO_BRig_RT_dataExp_Audio_freq__L.vi"() -> ("output_Audio_freq__L"=w2331:i32)  [unwired: 11 in]
              n1407 = call "myRIO_BRig_RT_dataExp_Audio_freq__R.vi"() -> ("output_Audio_freq__R"=w2330:i32)  [unwired: 11 in]
              n1408 = Index Array(array=w2329, index #1=w2333, index #2=w2332, index #3=w2331, index #4=w2330) -> (element #1=w2318:u16, element #2=w2317:u16, element #3=w2322:u16, element #4=w2321:u16)
              n1409 = To Unsigned Byte Integer(number=w2322) -> (unsigned 8bit integer=w2316:u8)
              n1410 = To Unsigned Byte Integer(number=w2321) -> (unsigned 8bit integer=w2315:u8)
              n1411 = xnode "Read/Write Control"("FPGA VI Reference In"=w2320, "error in"=w2319, "audioAmp_L"=w2318, "audioAmp_R"=w2317, "audioFreq_L_kHz"=w2316, "audioFreq_R_kHz"=w2315) -> ("error out"=w2314:errorcluster)  [unwired: 1 out]
              n1412 = local write "error out"(w2314) -> ()
            }
            frame "setSettings_Laser" {
              w2364 = u32 0 ("laser2_selRew_Ndelay")
              # "tDelay"
              # "Wrong l1"
              # "Reward l1"
              n1413 = call "myRIO_BRig_RT_dataExp_IallReward.vi"() -> ("output_I_allReward"=w2345:i32)  [unwired: 11 in]
              n1414 = local read "Laser_Tpeak_l1"() -> (w2375:dbl)
              n1415 = local read "Laser_Tshutter_l1"() -> (w2373:dbl)
              n1416 = local read "Laser_Freq_l1"() -> (w2374:dbl)
              n1417 = local read "Laser_duration_l1"() -> (w2349:u16)
              n1418 = local read "Laser_Tpeak_l2"() -> (w2371:dbl)
              n1419 = local read "Laser_Tshutter_l2"() -> (w2369:dbl)
              n1420 = local read "Laser_Freq_l2"() -> (w2370:dbl)
              n1421 = local read "Laser_duration_l2"() -> (w2348:u16)
              n1422 = local read "CueLed_Freq"() -> (w2358:dbl)
              n1423 = local read "CueLed_Tpeak"() -> (w2359:dbl)
              n1424 = local read "I_allReward"() -> (w2344:bool)
              n1425 = call "myRIO_BRig_RT_dataLC_Reward_Tdelay_l1.vi"() -> ("output_Reward_Tdelay_l1"=w2387:i32)  [unwired: 11 in]
              n1426 = call "myRIO_BRig_RT_dataLC_Wrong_Tdelay_l1.vi"() -> ("output_Wrong_Tdelay_l1"=w2388:i32)  [unwired: 11 in]
              n1427 = local read "FPGA_count2ms"() -> (w2360:dbl)
              n1428 = Index Array(array=w2355, index #1=w2387, index #2=w2388) -> (element #1=w2386:u16, element #2=w2385:u16)
              n1429 = To Double Precision Float(number=w2386) -> (double precision float=w2382:dbl)
              n1430 = To Double Precision Float(number=w2385) -> (double precision float=w2379:dbl)
              n1431 = Boolean To (0,1)(Boolean=w2344) -> (0, 1=w2343:i16)
              n1432 = To Unsigned Word Integer(number=w2343) -> (unsigned 16bit integer=w2342:u16)
              n1433 = Replace Array Subset(array=w2347, new element=w2342, index=w2345) -> (w2346:u16[])
              n1434 = To Unsigned Word Integer(number=w2360) -> (unsigned 16bit integer=w2376:u16)
              n1435 = call "myRIO_BRig_RT__calc_laser_FPGA_N.vi"("input_FPGA_ms2count"=w2360, "input_Tpeak"=w2375, "input_Freq"=w2374, "input_Tshutter"=w2373, "input_duration"=w2349) -> ("output_laser_Npeak"=w2363:u32, "output_laser_Nvalley"=w2362:u32, "output_laser_Nshutter"=w2361:u32, "output_laser_Nduration"=w2372:u32, "output_laser_Tduration"=w2353:u16)  [unwired: 6 in]
              n1436 = Multiply(x=w2360, y=w2382) -> (x*y=w2383:dbl)
              n1437 = Multiply(x=w2360, y=w2379) -> (x*y=w2380:dbl)
              n1438 = call "myRIO_BRig_RT__calc_laser_FPGA_N__CueLed.vi"("input_FPGA_ms2count"=w2360, "input_Tpeak"=w2359, "input_Freq"=w2358) -> ("output_laser_Npeak"=w2357:u32, "output_laser_Nvalley"=w2356:u32)  [unwired: 11 in]
              n1439 = call "myRIO_BRig_RT__calc_laser_FPGA_N.vi"("input_FPGA_ms2count"=w2360, "input_Tpeak"=w2371, "input_Freq"=w2370, "input_Tshutter"=w2369, "input_duration"=w2348) -> ("output_laser_Npeak"=w2368:u32, "output_laser_Nvalley"=w2367:u32, "output_laser_Nshutter"=w2366:u32, "output_laser_Nduration"=w2365:u32, "output_laser_Tduration"=w2352:u16)  [unwired: 6 in]
              n1440 = Round Toward +Infinity(x=w2383) -> (ceil(x): smallest int >= x=w2384:dbl)
              n1441 = Round Toward +Infinity(x=w2380) -> (ceil(x): smallest int >= x=w2381:dbl)
              n1442 = To Unsigned Long Integer(number=w2384) -> (unsigned 32bit integer=w2378:u32)
              n1443 = To Unsigned Long Integer(number=w2381) -> (unsigned 32bit integer=w2377:u32)
              n1444 = xnode "Read/Write Control"("FPGA VI Reference In"=w2389, "error in"=w2390, "I_allReward"=w2344, "LC_nPeak_l1"=w2363, "LC_nValley_l1"=w2362, "LC_nShutter_l1"=w2361, "LR_reward_nDelay_l1"=w2378, "LR_wrong_nDelay_l1"=w2377, "LR_reward_nTotal_l1"=w2372, "LR_wrong_nTotal_l1"=w2372, "k1__counter_per_ms"=w2376, "LC_nPeak_l2"=w2368, "LC_nValley_l2"=w2367, "LC_nShutter_l2"=w2366, "LR_reward_nDelay_l2"=w2364, "LR_wrong_nDelay_l2"=w2364, "LR_reward_nTotal_l2"=w2365, "LR_wrong_nTotal_l2"=w2365, "CueLed_nPeak"=w2357, "CueLed_nValley"=w2356) -> ("error out"=→"error out":errorcluster)  [unwired: 1 out]
              n1445 = call "myRIO_BRig_RT_dataCurrent_laser1_pulse_duration.vi"() -> ("output_laser1_pulse_duration"=w2351:i32)  [unwired: 11 in]
              n1446 = call "myRIO_BRig_RT_dataCurrent_laser2_pulse_duration.vi"() -> ("output_laser2_pulse_duration"=w2350:i32)  [unwired: 11 in]
              n1447 = Replace Array Subset(array=w2355, new element #1=w2353, index #1=w2351, new element #2=w2352, index #2=w2350) -> (w2354:u16[])
            }
            frame "initBlock" {
              n1448 = local write "nRewards_cur"(u16 0 ("nRewards_cur")) -> ()
              n1449 = call "myRIO_Brig_RT__Case_Exp_State_initBlock__v2.vi"("input_spout"=w2411, "input_dataCurrent"=w2417, "input_dataExp"=w2414, "input_dataBlock"=w2406) -> ("output_state"=w2410:T2, "output_spout"=w2409:enum16{"Left", "Right"}, "idxDataBlock"=w2412:i32, "output_dataCurrent"=w2416:u16[], "output_dataExp"=w2415:u16[], "output_TpB_target"=→"TpB_target":u16, "output_iBlock"=w2407:u16, "output_dataBlock"=w2405:u16[][])  [unwired: 4 in]
              "iBlock" <- w2407
              "cSpout" <- w2409
            }
            frame "initBlock2" {
              n1450 = call "myRIO_BRig_RT__Case_Exp_State_initBlock2.vi"("input_spout"=w2434, "input_dataBlock"=w2435, "input_dataCurrent"=w2433) -> ("idxDataBlock"=w2430:i32, "output_dataBlock"=w2432:u16[][])  [unwired: 7 in]
            }
            frame "initTrial" {
              n1451 = xnode "Read/Write Control"("FPGA VI Reference In"=w2450, "error in"=w2449, "SelectionState"=FALSE) -> ("error out"=w2448:errorcluster)  [unwired: 1 out]
              n1452 = call "myRIO_Brig_RT__Case_Exp_State_initTrial__v2.vi"("input_spout"=w2451, "input_dataBlock"=w2446, "input_dataExp"=w2462, "input_dataCurrent"=w2463) -> ("output_state"=w2464:T2, "output_dataExp"=w2461:u16[], "output_dataCurrent"=w2456:u16[], "output_iTrial"=w2445:u16, "output_SolenoidReward"=→"SolenoidReward":bool)  [unwired: 3 in]
              "iTrial" <- w2445
              n1453 = local write "error out"(w2448) -> ()
            }
            frame "initTrial2" {
              # "trialUntilReward"
              n1454 = call "myRIO_BRig_RT__Case_Exp_subState_LC__initTrial__v4.vi"("input_dataCurrent"=w2470, "input_dataExp"=w2468, "input_dataLC"=w2480, "input_spout"=w2481, "input_dataTrial"=w2483) -> ("output_dataTrial"=w2482:u16[][], "output_LR_Wrong_Laser_l2"=w2472:bool, "output_dataCurrent"=w2469:u16[], "output_LR_Reward_Laser_l2"=w2473:bool, "output_LR_Reward_Event_l1"=w2479:bool, "output_LR_Wrong_Event_l1"=w2478:bool, "output_LR_Reward_Laser_l1"=w2477:bool, "output_LR_Wrong_Laser_l1"=w2476:bool, "output_LR_Reward_Event_l2"=w2475:bool, "output_LR_Wrong_Event_l2"=w2474:bool)  [unwired: 5 in]
              n1455 = call "myRIO_BRig_RT_dataExp_ItrialUntilReward.vi"() -> ("output_I_trialUntilReward"=w2487:i32)  [unwired: 11 in]
              n1456 = Index Array(array=w2468, index=w2487) -> (element=w2486:u16)
              n1457 = Equal?(x=w2481, y=enum16{"Left", "Right"}."Right") -> (x = y?=w2485:bool)
              n1458 = Not Equal To 0?(x=w2486) -> (x != 0?=w2484:bool)
              n1459 = xnode "Read/Write Control"("FPGA VI Reference In"=w2497, "error in"=w2496, "Left(F)_or_Right(T)"=w2485, "ignoreWrong"=w2484, "LR_reward_Event_l1"=w2479, "LR_wrong_Event_l1"=w2478, "LR_reward_Laser_l1"=w2477, "LR_wrong_Laser_l1"=w2476, "LR_reward_Event_l2"=w2475, "LR_wrong_Event_l2"=w2474, "LR_reward_Laser_l2"=w2473, "LR_wrong_laser_l2"=w2472) -> ("error out"=w2471:errorcluster)  [unwired: 1 out]
              n1460 = local write "error out"(w2471) -> ()
            }
            frame "initTrial3" {
              # "Cue1_CueType"
              n1461 = call "myRIO_BRig_RT_dataExp_CueLed.vi"() -> ("output_CueLed"=w2504:i32)  [unwired: 11 in]
              n1462 = call "myRIO_BRig_RT_arrTrig_init.vi"() -> ("output_arrTrig"=w2508:bool[])  [unwired: 11 in]
              n1463 = Index Array(array=w2505, index=w2504) -> (element=w2503:u16)
              n1464 = call "myRIO_BRig_RT_arrTrig_Cue1_CueType_AudioLed.vi"() -> ("output_arrTrig_Cue1_CueType_AudioLed"=w2506:i32)  [unwired: 11 in]
              n1465 = Not Equal To 0?(x=w2503) -> (x != 0?=w2502:bool)
              n1466 = call "myRIO_BRig_RT__Case_Exp_State_initTrial_dataTrial.vi"("input_spout"=w2523, "input_dataCurrent"=w2510, "input_dataExp"=w2505, "input_dataTrial"=w2525) -> ("output_laserPower_l2"=w2512:u16, "output_dataCurrent"=w2509:u16[], "output_dataTrial"=w2524:u16[][], "output_laserPower_l1"=w2520:u16)  [unwired: 4 in]
              n1467 = To Double Precision Float(number=w2520) -> (double precision float=w2522:dbl)
              n1468 = To Double Precision Float(number=w2512) -> (double precision float=w2515:dbl)
              n1469 = Replace Array Subset(array=w2508, new element=w2502, index=w2506) -> (w2507:bool[])
              n1470 = Divide(x=w2522, y=100.0 ("x")) -> (x/y=w2517:dbl)
              "power_l1" <- w2517
              n1471 = Divide(x=w2515, y=100.0 ("x")) -> (x/y=w2513:dbl)
              "power_l2" <- w2513
              n1472 = call "myRIO__convert__Voltage_to_FPGAvalue.vi"("input_voltage"=w2517) -> ("output_PortC"=w2516:i16)  [unwired: 9 in, 1 out]
              n1473 = call "myRIO__convert__Voltage_to_FPGAvalue.vi"("input_voltage"=w2513) -> ("output_PortC"=w2511:i16)  [unwired: 9 in, 1 out]
              n1474 = xnode "Read/Write Control"("FPGA VI Reference In"=w2519, "error in"=w2518, "AnaOut_0"=w2516, "AnaOut_1"=w2511) -> ("error out"=w2501:errorcluster)  [unwired: 1 out]
              n1475 = local write "error out"(w2501) -> ()
            }
            frame "initTrial4" {
              n1476 = call "myRIO_BRig_RT_dataTrial_activeRecording.vi"() -> ("output_activeRecording"=w2545:i32)  [unwired: 11 in]
              n1477 = call "myRIO_BRig_RT_dataCurrent_idxDataTrial.vi"() -> ("output_idxDataTrial"=w2548:i32)  [unwired: 11 in]
              n1478 = Index Array(array=w2550, index=w2548) -> (element=w2547:u16)
              n1479 = xnode "Read/Write Control"("FPGA VI Reference In"=w2540, "error in"=w2539, "A6_Act"="Recording") -> ("error out"=w2537:errorcluster)  [unwired: 1 out]
              n1480 = Boolean To (0,1)(Boolean="Recording") -> (0, 1=w2544:i16)
              n1481 = To Long Integer(number=w2547) -> (32bit integer=w2546:i32)
              n1482 = To Unsigned Word Integer(number=w2544) -> (unsigned 16bit integer=w2543:u16)
              n1483 = local write "error out"(w2537) -> ()
              n1484 = Replace Array Subset(array=w2549, new element=w2543, index (row)=w2546, index (col)=w2545) -> (w2542:u16[][])
            }
            frame "initTrial_LC_ENL1" {
              n1485 = call "myRIO_BRig_RT__Case_Exp_State_initTrial_LC_ENL1__v4.vi"("input_dataTrial"=w2569, "input_spout"=w2572, "input_arrTrig"=w2566, "input_dataBlock"=w2567, "input_dataLC"=w2573, "input_dataCurrent"=w2571) -> ("output_arrTrig"=w2565:bool[], "output_dataTrial"=w2568:u16[][], "output_dataCurrent"=w2570:u16[])  [unwired: 3 in]
            }
            frame "initTrial_LC_Cue1" {
              n1486 = call "myRIO_BRig_RT__Case_Exp_State_initTrial_LC_Cue1__v4.vi"("input_dataTrial"=w2588, "input_spout"=w2591, "input_arrTrig"=w2585, "input_dataBlock"=w2586, "input_dataLC"=w2592, "input_dataCurrent"=w2590) -> ("output_arrTrig"=w2584:bool[], "output_dataTrial"=w2587:u16[][], "output_dataCurrent"=w2589:u16[])  [unwired: 3 in]
            }
            frame "initTrial_LC_Sel" {
              n1487 = xnode "Read/Write Control"("FPGA VI Reference In"=w2605, "error in"=w2604, "A6_Act"=FALSE) -> ("error out"=w2606:errorcluster)  [unwired: 1 out]
              n1488 = local write "error out"(w2606) -> ()
              n1489 = call "myRIO_BRig_RT__Case_Exp_State_initTrial_LC_Sel__v4.vi"("input_dataTrial"=w2611, "input_spout"=w2614, "input_arrTrig"=w2608, "input_dataBlock"=w2609, "input_dataLC"=w2615, "input_dataCurrent"=w2613) -> ("output_arrTrig"=w2607:bool[], "output_dataTrial"=w2610:u16[][], "output_dataCurrent"=w2612:u16[])  [unwired: 3 in]
            }
            frame "ENL1_pre" {
              n1490 = call "myRIO_BRig_RT__Case_Exp_State_Enl1Pre__v3.vi"("input_I_lick"=w2629, "input_arrTrig"=w2626, "input_dataCurrent"=w2630) -> ("output_dataCurrent"=w2627:u16[], "output_state"=w2628:T2)  [unwired: 3 in, 4 out]
            }
            frame "ENL1" {
              n1491 = call "myRIO_BRig_RT__Case_Exp_State_ENL1__v3.vi"("I_lick"=w2649, "input_arrTrig"=w2647, "input_state"=w2653, "input_dataCurrent"=w2652) -> ("output_l1_laserOn"=w2645:bool, "output_l1_laserEvent"=w2646:bool, "output_state"=w2650:T2, "output_dataCurrent"=w2651:u16[], "output_l2_laserEvent"=w2644:bool, "output_l2_laserOn"=w2643:bool)  [unwired: 2 in]
            }
            frame "ENL1Penalty_pre" {
              # "Tcycle"
              # "counter"
              n1492 = call "myRIO_BRig_RT_dataCurrent_Tcycle_generic.vi"() -> ("output_Tcycle_generic"=w2680:i32)  [unwired: 11 in]
              n1493 = call "myRIO_BRig_RT_dataCurrent_count_generic.vi"() -> ("output_count_generic"=w2682:i32)  [unwired: 11 in]
              n1494 = call "myRIO_BRig_RT_dataExp_ENL_penalty.vi"() -> ("output_ENL_penalty"=w2675:i32)  [unwired: 11 in]
              n1495 = Index Array(array=w2676, index=w2675) -> (element=w2679:u16)
              n1496 = Replace Array Subset(array=w2677, new element #1=u16 0 ("new element/subarray"), index #1=w2682, new element #2=w2679, index #2=w2680) -> (w2678:u16[])
            }
            frame "ENL1Penalty" {
              n1497 = call "myRIO_BRig_RT__Case_Exp_State_ENL1Penalty.vi"("input_state"=w2696, "input_dataCurrent"=w2700) -> ("output_state"=w2697:T2, "output_dataCurrent"=w2699:u16[])  [unwired: 8 in]
            }
            frame "ENL2_pre" {
            }
            frame "ENL2" {
            }
            frame "ENL2Penalty_pre" {
            }
            frame "ENL2Penalty" {
            }
            frame "Cue1_pre" {
              n1498 = call "myRIO_BRig_RT__Case_Exp_State_Cue1Pre__v3.vi"("input_dataCurrent"=w2772, "input_dataExp"=w2768, "input_arrTrig"=w2765, "input_spout"=w2769) -> ("output_audioR"=w2766:bool, "output_audioL"=w2767:bool, "output_state"=w2770:T2, "output_dataCurrent"=w2771:u16[])  [unwired: 7 in, 5 out]
            }
            frame "Cue1" {
              n1499 = call "myRIO_BRig_RT__Case_Exp_State_Cue1__v4.vi"("input_state"=w2793, "input_dataCurrent"=w2794, "I_lick"=w2792, "input_arrTrig"=w2795) -> ("output_SelectionState"=w2786:bool, "output_CueLed_Event"=w2791:bool, "output_state"=w2787:T2, "output_dataCurrent"=w2788:u16[], "output_l1_laserEvent"=w2784:bool, "output_l1_laserOn"=w2785:bool, "output_l2_laserEvent"=w2789:bool, "output_l2_laserOn"=w2790:bool)  [unwired: 8 in]
              n1500 = xnode "Read/Write Control"("FPGA VI Reference In"=w2798, "error in"=w2797, "SelectionState"=w2786) -> ()  [unwired: 2 out]
            }
            frame "Cue1Penalty_pre" {
              # "Tcycle"
              # "counter"
              n1501 = call "myRIO_BRig_RT_dataCurrent_Tcycle_generic.vi"() -> ("output_Tcycle_generic"=w2834:i32)  [unwired: 11 in]
              n1502 = call "myRIO_BRig_RT_dataCurrent_count_generic.vi"() -> ("output_count_generic"=w2836:i32)  [unwired: 11 in]
              n1503 = call "myRIO_BRig_RT_dataExp_CueLed.vi"() -> ("output_CueLed"=w2818:i32)  [unwired: 11 in]
              n1504 = call "myRIO_BRig_RT_dataExp_Tcycle_Cue1Penalty_Audio.vi"() -> ("output_Tcycle_Cue1Penalty_Audio"=w2819:i32)  [unwired: 11 in]
              n1505 = call "myRIO_BRig_RT_dataExp_Tcycle_Cue1Penalty_LED.vi"() -> ("output_Tcycle_Cue1Penalty_LED"=w2817:i32)  [unwired: 11 in]
              n1506 = Index Array(array=w2830, index #1=w2818, index #2=w2819, index #3=w2817) -> (element #1=w2816:u16, element #2=w2814:u16, element #3=w2813:u16)
              n1507 = Equal To 0?(x=w2816) -> (x = 0?=w2815:bool)
              n1508 = Select(t=w2814, s=w2815, f=w2813) -> (s? t:f=w2812:u16)
              n1509 = Replace Array Subset(array=w2832, new element #1=u16 0 ("new element/subarray"), index #1=w2836, new element #2=w2812, index #2=w2834) -> (w2831:u16[])
            }
            frame "Cue1Penalty" {
              n1510 = call "myRIO_BRig_RT__Case_Exp_State_Cue1Penalty.vi"("input_state"=w2853, "input_dataCurrent"=w2854) -> ("output_state"=w2851:T2, "output_dataCurrent"=w2852:u16[])  [unwired: 8 in]
            }
            frame "Cue2_pre" {
            }
            frame "Cue2" {
            }
            frame "Cue2Penalty_pre" {
            }
            frame "Cue2Penalty" {
            }
            frame "Selection_pre" {
              n1511 = xnode "Read/Write Control"("FPGA VI Reference In"=w2932, "error in"=w2933) -> ("error out"=w2920:errorcluster, "SelectReward"=w2927:bool, "SelectWrong"=w2928:bool)  [unwired: 1 out]
              n1512 = local write "error out"(w2920) -> ()
              n1513 = call "myRIO_BRig_RT__Case_Exp_State_SelectPre__v4.vi"("input_dataCurrent"=w2931, "input_SelectWrong"=w2928, "input_SelectReward"=w2927, "input_dataExp"=w2921, "input_LickL"=w2919, "input_LickR"=w2918, "input_arrTrig"=w2926) -> ("output_state"=w2929:T2, "output_dataCurrent"=w2930:u16[], "output_l1_laserEvent"=w2925:bool, "output_l1_laserOn"=w2924:bool, "output_l2_laserOn"=w2922:bool, "output_l2_laserEvent"=w2923:bool)  [unwired: 3 in]
            }
            frame "Selection" {
              n1514 = xnode "Read/Write Control"("FPGA VI Reference In"=w2960, "error in"=w2959) -> ("error out"=w2947:errorcluster, "SelectReward"=w2954:bool, "SelectWrong"=w2953:bool)  [unwired: 1 out]
              n1515 = local write "error out"(w2947) -> ()
              n1516 = call "myRIO_BRig_RT__Case_Exp_State_Selection__v4.vi"("input_dataCurrent"=w2958, "input_state"=w2956, "input_dataExp"=w2946, "input_LickL"=w2945, "input_FPGA_SelectReward"=w2954, "input_FPGA_SelectWrong"=w2953, "input_LickR"=w2944, "input_arrTrig"=w2952) -> ("output_state"=w2955:T2, "output_dataCurrent"=w2957:u16[], "output_LC_Event_l1"=w2951:bool, "output_LC_Laser_l2"=w2948:bool, "output_LC_Event_l2"=w2949:bool, "output_LC_Laser_l1"=w2950:bool)  [unwired: 2 in]
            }
            frame "SelectReward_pre" {
              # "iState"
              # "nRewTrials"
              # "Tcycle\nGeneric"
              # "counter"
              n1517 = call "myRIO_BRig_RT_dataCurrent_nRewTrials.vi"() -> ("output_nRewTrials"=w2984:i32)  [unwired: 11 in]
              n1518 = call "myRIO_BRig_RT_dataCurrent_Tcycle_reward.vi"() -> ("output_Tcycle_reward"=w2973:i32)  [unwired: 11 in]
              n1519 = Index Array(array=w2971, index #1=w2984, index #2=w2973) -> (element #1=w2983:u16, element #2=w2972:u16)
              n1520 = Increment(x=w2983) -> (x+1=w2982:u16)
              n1521 = call "myRIO_BRig_RT__Case_Exp_subState_LC__Reward.vi"("input_spout"=w2991, "input_dataCurrent"=w2971, "input_dataLC"=w2990) -> ()  [unwired: 6 in, 2 out]
              n1522 = call "myRIO_BRig_RT_dataCurrent_count_generic.vi"() -> ("output_count_generic"=w2986:i32)  [unwired: 11 in]
              n1523 = call "myRIO_BRig_RT_dataCurrent_Tcycle_generic.vi"() -> ("output_Tcycle_generic"=w2987:i32)  [unwired: 11 in]
              n1524 = call "myRIO_BRig_RT_dataCurrent_iState.vi"() -> ("output_iState"=w2981:i32)  [unwired: 11 in]
              n1525 = Replace Array Subset(array=w2971, new element #1=w2982, index #1=w2984, new element #2=u16 0 ("new element/subarray"), index #2=w2986, new element #3=w2972, index #3=w2987, new element #4=u16 1 ("new element/subarray"), index #4=w2981) -> (w2993:u16[])
            }
            frame "SelectReward" {
              n1526 = call "myRIO_BRig_RT__Case_Exp_State_Reward.vi"("input_dataCurrent"=w3010, "input_state"=w3007, "input_spout"=w3005) -> ("output_dataCurrent"=w3009:u16[], "output_state"=w3008:T2, "output__L"=w3003:bool, "output__R"=w3004:bool)  [unwired: 9 in]
            }
            frame "SelectRewardPost_pre" {
              # "nRewards"
              # "nRewTrials"
              # "Tcycle"
              # "counter"
              n1527 = call "myRIO_BRig_RT_dataBlock_nRewards__L.vi"() -> ("output_nRewards__L"=w3026:i32)  [unwired: 11 in]
              n1528 = call "myRIO_BRig_RT_dataBlock_nRewards__R.vi"() -> ("output_nRewards__R"=w3025:i32)  [unwired: 11 in]
              n1529 = call "myRIO_BRig_RT_dataCurrent_Tcycle_generic.vi"() -> ("output_Tcycle_generic"=w3041:i32)  [unwired: 11 in]
              n1530 = call "myRIO_BRig_RT_dataCurrent_count_generic.vi"() -> ("output_count_generic"=w3043:i32)  [unwired: 11 in]
              n1531 = case shown="\"Left\", Default" w3019 {
                tunnel: w3031 -> [w3048 w3052]
                tunnel: [w3047 w3052] -> w3030
                tunnel: [w3049 w3050] -> w3029
                tunnel: w3028 -> [w3049 w3051]
                frame "Left", Default {
                  n1532 = Increment(x=w3048) -> (x+1=w3047:u16)
                }
                frame "Right" {
                  n1533 = Increment(x=w3051) -> (x+1=w3050:u16)
                }
              }
              "nRewards_Left" <- w3030
              "nRewards_Right" <- w3029
              n1534 = Equal?(x=w3019, y=enum16{"Left", "Right"}."Left") -> (x = y?=w3018:bool)
              n1535 = Select(t=w3026, s=w3018, f=w3025) -> (s? t:f=w3024:i32)
              n1536 = call "myRIO_BRig_RT_dataExp_Tcycle_RewardPost.vi"() -> ("output_Tcycle_RewardPost"=w3037:i32)  [unwired: 11 in]
              n1537 = call "myRIO_BRig_RT_dataCurrent_nRewTrials.vi"() -> ("output_nRewTrials"=w3027:i32)  [unwired: 11 in]
              n1538 = Index Array(array=w3038, index=w3037) -> (element=w3040:u16)
              n1539 = Index Array(array=w3021, index=w3027) -> (element=w3016:u16)
              n1540 = Replace Array Subset(array=w3021, new element #1=u16 0 ("new element/subarray"), index #1=w3043, new element #2=w3040, index #2=w3041) -> (w3039:u16[])
              n1541 = Replace Array Subset(array=w3023, new element=w3016, index (row)=w3017, index (col)=w3024) -> (w3022:u16[][])
              n1542 = local write "nRewards_cur"(w3016) -> ()
            }
            frame "SelectRewardPost" {
              n1543 = call "myRIO_BRig_RT__Case_Exp_State_RewardPost.vi"("input_state"=w3063, "input_dataCurrent"=w3066) -> ("output_state"=w3064:T2, "output_dataCurrent"=w3065:u16[])  [unwired: 8 in]
            }
            frame "SelectWrong_pre" {
              # "iState"
              # "Tcycle"
              # "counter"
              n1544 = call "myRIO_BRig_RT_dataCurrent_Tcycle_generic.vi"() -> ("output_Tcycle_generic"=w3087:i32)  [unwired: 11 in]
              n1545 = call "myRIO_BRig_RT_dataCurrent_count_generic.vi"() -> ("output_count_generic"=w3089:i32)  [unwired: 11 in]
              n1546 = call "myRIO_BRig_RT_dataExp_Tcycle_Wrong.vi"() -> ("output_Tcycle_Wrong"=w3085:i32)  [unwired: 11 in]
              n1547 = call "myRIO_BRig_RT__Case_Exp_subState_LC__Wrong.vi"("input_spout"=w3081, "input_dataCurrent"=w3082, "input_dataLC"=w3079) -> ()  [unwired: 6 in, 2 out]
              n1548 = Index Array(array=w3083, index=w3085) -> (element=w3086:u16)
              n1549 = call "myRIO_BRig_RT_dataCurrent_iState.vi"() -> ("output_iState"=w3077:i32)  [unwired: 11 in]
              n1550 = Replace Array Subset(array=w3082, new element #1=u16 0 ("new element/subarray"), index #1=w3089, new element #2=w3086, index #2=w3087, new element #3=u16 2 ("new element/subarray"), index #3=w3077) -> (w3084:u16[])
            }
            frame "SelectWrong" {
              n1551 = call "myRIO_BRig_RT__Case_Exp_State_Wrong.vi"("input_state"=w3103, "input_dataCurrent"=w3108) -> ("output_state"=w3100:T2, "output_dataCurrent"=w3107:u16[])  [unwired: 8 in]
              n1552 = Not Equal?(x=w3103, y=w3100) -> (x != y?=w3102:bool)
              n1553 = Select(t=myRIO_BRig_RT__Case_Exp_stateList."SelectWrong_post" ("Enum"), s=w3102, f=w3100) -> (s? t:f=w3099:T2)
            }
            frame "SelectWrong_post" {
            }
            frame "SelectTimeout_pre" {
              # "iState"
              # "Tcycle"
              # "counter"
              n1554 = xnode "Read/Write Control"("FPGA VI Reference In"=w3131, "error in"=w3130, "SelectionState"=FALSE) -> ("error out"=w3128:errorcluster)  [unwired: 1 out]
              n1555 = call "myRIO_BRig_RT_dataCurrent_Tcycle_generic.vi"() -> ("output_Tcycle_generic"=w3149:i32)  [unwired: 11 in]
              n1556 = call "myRIO_BRig_RT_dataCurrent_count_generic.vi"() -> ("output_count_generic"=w3147:i32)  [unwired: 11 in]
              n1557 = call "myRIO_BRig_RT_dataExp_Tcycle_Timeout.vi"() -> ("output_Tcycle_Timeout"=w3151:i32)  [unwired: 11 in]
              n1558 = local write "error out"(w3128) -> ()
              n1559 = call "myRIO_BRig_RT__Case_Exp_subState_LC__Timeout.vi"("input_spout"=w3142, "input_dataCurrent"=w3143, "input_dataLC"=w3141) -> ()  [unwired: 6 in, 2 out]
              n1560 = Index Array(array=w3145, index=w3151) -> (element=w3150:u16)
              n1561 = call "myRIO_BRig_RT_dataCurrent_iState.vi"() -> ("output_iState"=w3139:i32)  [unwired: 11 in]
              n1562 = Replace Array Subset(array=w3143, new element #1=u16 0 ("new element/subarray"), index #1=w3147, new element #2=w3150, index #2=w3149, new element #3=u16 3 ("new element/subarray"), index #3=w3139) -> (w3146:u16[])
            }
            frame "SelectTimeout" {
              n1563 = call "myRIO_BRig_RT__Case_Exp_State_Timeout.vi"("input_dataLC"=w3166, "input_state"=w3161, "input_dataCurrent"=w3171) -> ("output_state"=w3162:T2, "output_dataCurrent"=w3170:u16[])  [unwired: 6 in, 1 out]
              n1564 = Not Equal?(x=w3161, y=w3162) -> (x != y?=w3165:bool)
              n1565 = Select(t=myRIO_BRig_RT__Case_Exp_stateList."SelectTimeout_post" ("Enum"), s=w3165, f=w3162) -> (s? t:f=w3163:T2)
            }
            frame "SelectTimeout_post" {
            }
            frame "endTrial1" {
              # "Update dataBlock"
              n1566 = call "myRIO_BRig_RT__Case_Exp_State_endTrial1.vi"("input_spout"=w3200, "input_dataBlock"=w3199, "input_dataCurrent"=w3197) -> ("output_dataBlock"=w3198:u16[][], "output_dataCurrent"=w3196:u16[])  [unwired: 7 in]
            }
            frame "endTrial2" {
              # "update dataTrial"
              n1567 = call "myRIO_BRig_RT__Case_Exp_State_endTrial2.vi"("input_dataExp"=w3207, "input_spout"=w3216, "input_dataTrial"=w3220, "input_dataCurrent"=w3218) -> ("output_dataTrial"=w3219:u16[][], "output_dataCurrent"=w3217:u16[])  [unwired: 6 in]
            }
            frame "endTrial3" {
              # "nRewTrials"
              # "iTrial"
              # "I_blockUntilReward"
              # "TPB"
              # "end block?"
              n1568 = local read "STOP_endTrial"() -> (w3241:bool)
              n1569 = local read "STOP_abort"() -> (w3240:bool)
              n1570 = xnode "Read/Write Control"("FPGA VI Reference In"=w3231, "error in"=w3230, "SelectionState"=FALSE) -> ("error out"=w3224:errorcluster)  [unwired: 1 out]
              n1571 = local read "START"() -> (w3238:bool)
              n1572 = call "myRIO_BRig_RT_dataExp_IblockUntilReward.vi"() -> ("output_I_blockUntilReward"=w3248:i32)  [unwired: 11 in]
              n1573 = Index Array(array=w3234, index=w3248) -> (element=w3232:u16)
              n1574 = Not(x=w3238) -> (.not. x?=w3239:bool)
              n1575 = local write "error out"(w3224) -> ()
              n1576 = Not Equal To 0?(x=w3232) -> (x != 0?=w3246:bool)
              n1577 = Compound Arithmetic op=OR(w3241, w3239, w3240) -> (w3227:bool)
              n1578 = call "myRIO_BRig_RT_dataCurrent_nRewTrials.vi"() -> ("output_nRewTrials"=w3244:i32)  [unwired: 11 in]
              n1579 = call "myRIO_BRig_RT_dataCurrent_iTrial.vi"() -> ("output_iTrial"=w3245:i32)  [unwired: 11 in]
              n1580 = Select(t=w3244, s=w3246, f=w3245) -> (s? t:f=w3243:i32)
              n1581 = call "myRIO_BRig_RT_dataCurrent_TpB.vi"() -> ("output_TpB"=w3247:i32)  [unwired: 11 in]
              n1582 = Index Array(array=w3235, index #1=w3247, index #2=w3243) -> (element #1=w3236:u16, element #2=w3237:u16)
              n1583 = Less Or Equal?(x=w3236, y=w3237) -> (x <= y?=w3228:bool)
              n1584 = Or(x=w3227, y=w3228) -> (x .or. y?=w3225:bool)
              n1585 = Select(t=myRIO_BRig_RT__Case_Exp_stateList."saveData_dataBlock" ("Enum"), s=w3225, f=myRIO_BRig_RT__Case_Exp_stateList."dummyState" ("Enum")) -> (s? t:f=w3233:T2)
            }
            frame "endBlock" {
              # "R"
              # "L"
              # "idxDataBlock"
              n1586 = Equal?(x=w3268, y=enum16{"Left", "Right"}."Left") -> (x = y?=w3267:bool)
              n1587 = call "myRIO_BRig_RT_dataCurrent_idxDataBlockL.vi"() -> ("output_idxDataBlock__L"=w3271:i32)  [unwired: 11 in]
              n1588 = call "myRIO_BRig_RT_dataCurrent_idxDataBlockR.vi"() -> ("output_idxDataBlock__R"=w3270:i32)  [unwired: 11 in]
              n1589 = Increment(x=w3262) -> (x+1=w3261:i32)
              n1590 = local read "START"() -> (w3287:bool)
              n1591 = local read "STOP_endBlock"() -> (w3282:bool)
              n1592 = local read "STOP_endTrial"() -> (w3285:bool)
              n1593 = local read "STOP_abort"() -> (w3284:bool)
              n1594 = Select(t=w3271, s=w3267, f=w3270) -> (s? t:f=w3265:i32)
              n1595 = To Unsigned Word Integer(number=w3261) -> (unsigned 16bit integer=w3263:u16)
              n1596 = Not(x=w3287) -> (.not. x?=w3286:bool)
              n1597 = Replace Array Subset(array=w3266, new element=w3263, index=w3265) -> (w3264:u16[])
              n1598 = Compound Arithmetic op=OR(w3286, w3282, w3285, w3284) -> (w3283:bool)
              n1599 = Select(t=myRIO_BRig_RT__Case_Exp_stateList."endExp" ("Enum"), s=w3283, f=myRIO_BRig_RT__Case_Exp_stateList."dummyState_endBlock" ("Enum")) -> (s? t:f=w3291:T2)
            }
            frame "endExp" {
              n1600 = xnode "Read/Write Control"("FPGA VI Reference In"=w3294, "error in"=w3293, "A6_Act"=FALSE) -> ("error out"=w3295:errorcluster)  [unwired: 1 out]
              n1601 = local write "error out"(w3295) -> ()
            }
            frame "commConnect" {
              n1602 = call "myRIO_BRig_RT_comm_webdav_connect.vi"("input_password"="Host Password", "input_username"="Host UserName") -> ("output_Iconnected"=w3312:bool, "output_hSession"=w3326:T6)  [unwired: 7 in, 1 out]
              "Connected To Host?" <- w3312
              n1603 = case shown="False" w3312 {
                frame False {
                  n1604 = One Button Dialog(message="Connection Failed!\nData not being saved!") -> ()  [unwired: 1 in, 1 out]
                }
                frame True {
                }
              }
            }
            frame "commUpload_pre" {
              n1605 = Select(t=myRIO_BRig_RT__Case_Exp_stateList."commUpload_dataBlock" ("Enum"), s=w3333, f=myRIO_BRig_RT__Case_Exp_stateList."endBlock") -> (s? t:f=w3331:T2)
            }
            frame "commUpload_dataBlock" {
              n1606 = call "myRIO_BRig_RT_comm_webdav_uploadFile__data.vi"("input_fileName_prefix"=w3350, "input_fileName"="dataBlock" ("input_filename"), "input_hSession"=w3352) -> ()  [unwired: 8 in, 1 out]
            }
            frame "commUpload_dataCurrent" {
              n1607 = call "myRIO_BRig_RT_comm_webdav_uploadFile__data.vi"("input_fileName_prefix"=w3367, "input_fileName"="dataCurrent" ("input_filename"), "input_hSession"=w3369) -> ()  [unwired: 8 in, 1 out]
            }
            frame "commUpload_dataExp" {
              n1608 = call "myRIO_BRig_RT_comm_webdav_uploadFile__data.vi"("input_fileName_prefix"=w3384, "input_fileName"="dataExp" ("input_filename"), "input_hSession"=w3386) -> ()  [unwired: 8 in, 1 out]
            }
            frame "commUpload_dataLC" {
              n1609 = call "myRIO_BRig_RT_comm_webdav_uploadFile__data.vi"("input_fileName_prefix"=w3401, "input_fileName"="dataLC" ("input_filename"), "input_hSession"=w3403) -> ()  [unwired: 8 in, 1 out]
            }
            frame "commUpload_dataTrial" {
              n1610 = call "myRIO_BRig_RT_comm_webdav_uploadFile__data.vi"("input_fileName_prefix"=w3421, "input_fileName"="dataTrial" ("input_filename"), "input_hSession"=w3423) -> ()  [unwired: 8 in, 1 out]
            }
            frame "saveData_dataBlock" {
              # "idxDataBlockR"
              # "idxDataBlockL"
              n1611 = call "myRIO_BRig_RT_dataCurrent_idxDataBlockL.vi"() -> ("output_idxDataBlock__L"=w3443:i32)  [unwired: 11 in]
              n1612 = call "myRIO_BRig_RT_dataCurrent_idxDataBlockR.vi"() -> ("output_idxDataBlock__R"=w3444:i32)  [unwired: 11 in]
              n1613 = Index Array(array=w3445, index #1=w3443, index #2=w3444) -> (element #1=w3442:u16, element #2=w3441:u16)
              n1614 = Greater?(x=w3442, y=w3441) -> (0:w3440:bool)
              n1615 = Select(t=w3442, s=w3440, f=w3441) -> (s? t:f=w3438:u16)
              n1616 = Increment(x=w3438) -> (x+1=w3437:u16)
              n1617 = To Long Integer(number=w3437) -> (32bit integer=w3436:i32)
              n1618 = Array Subset(array=w3439, length (row)=w3436) -> (w3435:u16[][])  [unwired: 3 in]
              n1619 = call "myRIO_BRig_RT_comm_webdav_saveArrayToFile__2D_u16.vi"("Array"=w3435, "input_filename"="dataBlock") -> ()  [unwired: 10 in]
            }
            frame "saveData_dataCurrent" {
              n1620 = call "myRIO_BRig_RT_comm_webdav_saveArrayToFile__1D_u16.vi"("Array"=w3460, "input_filename"="dataCurrent") -> ()  [unwired: 10 in]
            }
            frame "saveData_dataExp" {
              # "runTime"
              n1621 = Get Date/Time In Seconds() -> (seconds since 1Jan1904=w3484:timestamp)
              n1622 = To Double Precision Float(number=w3484) -> (double precision float=w3483:dbl)
              n1623 = call "myRIO_BRig_RT_dataExp_runTime_seconds.vi"() -> ("output_RunTime_minutes"=w3482:i32)  [unwired: 11 in]
              n1624 = Subtract(x=w3483, y=w3481) -> (x-y=w3478:dbl)
              n1625 = To Unsigned Word Integer(number=w3478) -> (unsigned 16bit integer=w3477:u16)
              n1626 = Replace Array Subset(array=w3476, new element=w3477, index=w3482) -> (w3479:u16[])
              n1627 = call "myRIO_BRig_RT_comm_webdav_saveArrayToFile__1D_u16.vi"("Array"=w3479, "input_filename"="dataExp") -> ()  [unwired: 10 in]
            }
            frame "saveData_dataLC" {
              n1628 = call "myRIO_BRig_RT_comm_webdav_saveArrayToFile__1D_u16.vi"("Array"=w3499, "input_filename"="dataLC") -> ()  [unwired: 10 in]
            }
            frame "saveData_dataTrial" {
              # "idxTrial"
              n1629 = call "myRIO_BRig_RT_dataCurrent_idxDataTrial.vi"() -> ("output_idxDataTrial"=w3519:i32)  [unwired: 11 in]
              n1630 = Index Array(array=w3520, index=w3519) -> (element=w3512:u16)
              n1631 = Increment(x=w3512) -> ()  [unwired: 1 out]
              n1632 = To Long Integer(number=w3512) -> (32bit integer=w3516:i32)
              n1633 = Array Subset(array=w3517, length (row)=w3516) -> (w3518:u16[][])  [unwired: 3 in]
              n1634 = call "myRIO_BRig_RT_comm_webdav_saveArrayToFile__2D_u16.vi"("Array"=w3518, "input_filename"="dataTrial") -> ()  [unwired: 10 in]
            }
            frame "dummyState" {
              n1635 = call "myRIO_BRig_RT_dataCurrent_iTrial.vi"() -> ("output_iTrial"=w3538:i32)  [unwired: 11 in]
              n1636 = Index Array(array=w3539, index=w3538) -> (element=w3537:u16)
              n1637 = Equal?(x=w3537, y=u16 1) -> (x = y?=w3535:bool)
              n1638 = Equal To 0?(x=w3546) -> (x = 0?=w3547:bool)
              n1639 = Select(t=u16 13, s=w3535, f=u16 15) -> (s? t:f=w3532:u16)
              n1640 = Select(t=w3532, s=w3547, f=w3546) -> (s? t:f=w3545:u16)
              n1641 = Decrement(x=w3545) -> (x-1=w3544:u16)
              n1642 = Equal To 0?(x=w3544) -> (x = 0?=w3543:bool)
              n1643 = Select(t=myRIO_BRig_RT__Case_Exp_stateList."initTrial" ("Enum"), s=w3543, f=w3541) -> (s? t:f=w3540:T2)
            }
            frame "dummyState_endBlock" {
              n1644 = call "myRIO_BRig_RT_dataCurrent_iTrial.vi"() -> ("output_iTrial"=w3567:i32)  [unwired: 11 in]
              n1645 = Index Array(array=w3568, index=w3567) -> (element=w3566:u16)
              n1646 = Equal?(x=w3566, y=u16 1) -> (x = y?=w3564:bool)
              n1647 = Equal To 0?(x=w3575) -> (x = 0?=w3576:bool)
              n1648 = Select(t=u16 1, s=w3564, f=u16 3) -> (s? t:f=w3561:u16)
              n1649 = Select(t=w3561, s=w3576, f=w3575) -> (s? t:f=w3574:u16)
              n1650 = Decrement(x=w3574) -> (x-1=w3573:u16)
              n1651 = Equal To 0?(x=w3573) -> (x = 0?=w3572:bool)
              n1652 = Select(t=myRIO_BRig_RT__Case_Exp_stateList."initBlock" ("Enum"), s=w3572, f=w3570) -> (s? t:f=w3569:T2)
            }
          }
          n1653 = call "myRIO_BRig_RT_dataMTrig_main.vi"("input_dataMTrig"=w1660, "input_Solenoid_trig_L"=w1657, "input_Solenoid_trig_R"=w1656, "input_Audio_trig_L"=w1655, "input_Audio_trig_R"=w1654, "input_Laser_trig"=w1653) -> ("output_Laser"=w1594:bool, "output_dataMTrig"=w1659:u16[], "output_Solenoid_L"=w1597:bool, "output_Solenoid_R"=w1649:bool, "output_Audio_L"=w1651:bool, "output_Audio_R"=w1652:bool)  [unwired: 8 in]
          n1654 = Compound Arithmetic op=OR(w1657, w1656, w1655, w1654, w1653) -> (w1658:bool)
          n1655 = case shown="True" w1658 {
            frame False {
            }
            frame True {
              w1690 = FALSE
              n1656 = local write "MTrig_Solenoid_trig__L"(w1690) -> ()
              n1657 = local write "MTrig_Solenoid_trig__R"(w1690) -> ()
              n1658 = local write "MTrig_Audio_trig__L"(w1690) -> ()
              n1659 = local write "MTrig_Audio_trig__R"(w1690) -> ()
              n1660 = local write "MTrig_Laser_trig"(w1690) -> ()
            }
          }
          n1661 = local read "MTrig_Laser_Switch"() -> (w1592:bool)
          n1662 = Not(x=w1592) -> (.not. x?=w1593:bool)
          n1663 = And(x=w1594, y=w1593) -> (x .and. y?=w1588:bool)
          n1664 = And(x=w1594, y=w1592) -> (x .and. y?=w1590:bool)
          n1665 = Or(x=w1591, y=w1590) -> (x .or. y?=w1581:bool)
          n1666 = Or(x=w1590, y=w1589) -> (x .or. y?=w1580:bool)
          n1667 = Or(x=w1587, y=w1588) -> (x .or. y?=w1583:bool)
          n1668 = Or(x=w1588, y=w1586) -> (x .or. y?=w1582:bool)
          n1669 = Or(x=w1596, y=w1597) -> (x .or. y?=w1585:bool)
          n1670 = Or(x=w1650, y=w1649) -> (x .or. y?=w1584:bool)
          n1671 = case shown="False" w1670 {
            tunnel: w1667 -> [w1692 w1700]
            tunnel: w1669 -> [_ w1697]
            tunnel: w1668 -> [_ w1696]
            tunnel: w1571 -> [_ w1695]
            tunnel: w1647 -> [_ w1694]
            tunnel: [w1692 w1699] -> w1666
            tunnel: [w1691 w1698] -> w1665
            tunnel: w1579 -> [w1691 w1693]
            frame False {
            }
            frame True {
              n1672 = call "myRIO_BRig_RT__Case_Exp__recordLick.vi"("intput_state__trialEnd"=w1694, "intput_state__trialStart"=w1695, "input_lick__R"=w1696, "input_lick__L"=w1697, "input_dataCurrent"=w1693, "input_dataLick"=w1700) -> ("output_dataCurrent"=w1698:u16[], "output_dataLick"=w1699:u16[][])  [unwired: 4 in]
            }
          }
          n1673 = Or(x=w1651, y=w1637) -> (x .or. y?=w1627:bool)
          n1674 = Or(x=w1636, y=w1652) -> (x .or. y?=w1648:bool)
          n1675 = Or(x=w1671, y="STOP_abort") -> (x .or. y?=w1673:bool)
          n1676 = Select(t=w1617, s=w1618, f=w1616) -> (s? t:f=w1607:u16)
          n1677 = Select(t=w1578, s=w1620, f=w1619) -> (s? t:f=w1606:u16)
          n1678 = Select(t=u16 0, s=w1623, f=w1622) -> (s? t:f=w1609:u16)
          n1679 = xnode "Read/Write Control"("FPGA VI Reference In"=w1629, "error in"=w1628, "audioTrigger_L"=w1627, "audioTrigger_R"=w1648, "CueLed_Event"=w1595, "A3_SL"=w1585, "A1_SR"=w1584, "LC_Event_l1"=w1583, "LC_Laser_l1"=w1582, "LC_Event_l2"=w1581, "LC_Laser_l2"=w1580) -> ("FPGA VI Reference Out"=w1664:refnum<k20>, "error out"=w1663:errorcluster, "AnaIn_0"=w1600:i16, "AnaIn_1"=w1608:i16)
          n1680 = call "myRIO_BRig_RT_dataAnalog_enterData__PortC.vi"("input_iState"=w1571, "input_AI0"=w1600, "input_iEvent"=w1609, "input_AI1"=w1608, "input_iTrial"=w1607, "input_iBlock"=w1606, "input_index"=w1610, "input_dataAnalog"=w1626) -> ("output_dataAnalog"=w1625:u16[][])  [unwired: 3 in]
          n1681 = call "myRIO_BRig_RT_TCP__v3__PortC.vi"("input_hTCP"=w1614, "input_AI1"=w1608, "input_AI0"=w1600, "input_I_connected_TCP"=w1611, "input_iBlock"=w1606, "input_spout"=w1605, "input_iTrial"=w1607, "input_error"=w1612, "input_countTrial"=w1602, "input_iState"=w1571) -> ("output_hTCP"=w1613:refnum<k5>, "output_countTrial"=w1601:u16, "output_error"=w1575:errorcluster)  [unwired: 3 in]
          n1682 = call "test_myRIO_Exp_tLoop.vi"("input_error"=w1575, "input_Threshold"=w1572, "input_timestamp"=w1573, "input_state"=w1571) -> ("output_Threshold"=w1569:bool, "output_duration"=→"tLoop":dbl, "error out"=w1574:errorcluster)  [unwired: 5 in]
          "Threshold" <- w1569
          n1683 = node-c288() -> ()  [unwired: 1 in, 1 out]
          n1684 = Increment(x=w1609) -> (x+1=w1615:u16)
          n1685 = Increment(x=w1610) -> (x+1=w1624:i32)
          "cState" <- w1571
        }
        n1686 = node-c288(w1512) -> ()  [unwired: 1 out]
        n1687 = flat-sequence {
          tunnel: w1508 -> [w1557]
          tunnel: w1507 -> [w1556]
          tunnel: [w1555] -> w1500
          tunnel: [w1554] -> w1499
          tunnel: [w1560] -> w1501
          tunnel: [w1561] -> w1506
          tunnel: w1500 -> [w1561]
          tunnel: w1499 -> [w1560]
          frame #0 {
            w1551 = u8 0
            w1552 = u16 0 ("AudioLeft_phase_inc")
            w1553 = FALSE
            n1688 = xnode "Read/Write Control"("FPGA VI Reference In"=w1557, "error in"=w1556, "Counts_Reset"=TRUE, "audioTrigger_L"=w1553, "audioFreq_L_kHz"=w1551, "audioAmp_L"=w1552, "audioTrigger_R"=w1553, "audioFreq_R_kHz"=w1551, "audioAmp_R"=w1552, "A3_SL"=w1553, "A1_SR"=w1553, "A6_Act"=w1553) -> ("FPGA VI Reference Out"=w1555:refnum<k20>, "error out"=w1554:errorcluster)
          }
          frame #1 {
            w1559 = FALSE ("START")
            n1689 = local write "START"(w1559) -> ()
            n1690 = local write "STOP_endTrial"(w1559) -> ()
            n1691 = local write "STOP_endBlock"(w1559) -> ()
          }
        }
        n1692 = stacked-sequence {
          tunnel: w1485 -> [w1531 _]
          tunnel: w1483 -> [w1532 _]
          tunnel: w1482 -> [_ w1537]
          tunnel: w1481 -> [_ w1536]
          tunnel: w1480 -> [_ w1535]
          tunnel: w1479 -> [w1525 _]
          tunnel: w1461 -> [w1522 _]
          tunnel: w1460 -> [w1521 _]
          frame #0 {
            n1693 = call "myRIO_BRig_RT_dataCurrent_idxDataLick.vi"() -> ("output_idxDataLick"=w1526:i32)  [unwired: 11 in]
            n1694 = Index Array(array=w1525, index=w1526) -> (element=w1528:u16)
            n1695 = Array Subset(array=w1522, length (row)=w1521) -> (w1523:u16[][])  [unwired: 3 in]
            n1696 = Increment(x=w1528) -> (x+1=w1529:u16)
            n1697 = call "myRIO_BRig_RT_comm_webdav_saveArrayToFile__1D_u16.vi"("Array"=w1532, "input_filename"="dataMTrig") -> ()  [unwired: 10 in]
            n1698 = To Long Integer(number=w1529) -> (32bit integer=w1527:i32)
            n1699 = Array Subset(array=w1531, length (row)=w1527) -> (w1530:u16[][])  [unwired: 3 in]
            n1700 = call "myRIO_BRig_RT_comm_webdav_saveArrayToFile__2D_u16.vi"("Array"=w1530, "input_filename"="dataLick") -> ()  [unwired: 10 in]
            n1701 = call "myRIO_BRig_RT_comm_webdav_saveArrayToFile__2D_u16.vi"("Array"=w1523, "input_filename"="dataAnalog") -> ()  [unwired: 10 in]
          }
          frame #1 {
            n1702 = case shown="True" w1537 {
              tunnel: w1536 -> [_ w1539]
              tunnel: w1535 -> [_ w1538]
              frame False {
              }
              frame True {
                n1703 = stacked-sequence {
                  tunnel: w1539 -> [w1541 w1548 w1550]
                  tunnel: w1538 -> [w1542 w1547 _]
                  frame #0 {
                    n1704 = call "myRIO_BRig_RT_comm_webdav_uploadFile__announce.vi"("input_addText"=TRUE, "input_fileName_prefix"=w1542, "intput_fileName"="curExp_end", "intput_hSession"=w1541) -> ("output_Isuccess"=w1540:bool)  [unwired: 6 in, 1 out]
                    n1705 = case shown="True" w1540 {
                      frame False {
                        n1706 = One Button Dialog(message="!!! Warning !!! Your data is located at C:\\BehaviorRig\\commTransfer") -> ()  [unwired: 1 in, 1 out]
                      }
                      frame True {
                        n1707 = Wait (ms)(milliseconds to wait=u32 20) -> ()  [unwired: 1 out]
                      }
                    }
                  }
                  frame #1 {
                    n1708 = call "myRIO_BRig_RT__endExp_sendData.vi"("input_fileName_prefix"=w1547, "input_hSession"=w1548) -> ()  [unwired: 8 in, 2 out]
                  }
                  frame #2 {
                    n1709 = local write "Connected To Host?"(FALSE ("Connected To Host?")) -> ()
                    n1710 = call <vilib>:"Close Session.vi"("session handle"=w1550) -> ()  [unwired: 14 in, 1 out]
                  }
                }
              }
            }
          }
        }
      }
    }
    n1711 = local read "STOP_abort"() -> (w44:bool)
  }
  n1712 = case shown="True" w5 {
    tunnel: w4 -> [_ w3595]
    tunnel: w3 -> [_ w3594]
    frame False {
    }
    frame True {
      n1713 = call "myRIO__TCP_disconnect_forWrite.vi"("input_error"=w3594, "input_hTCP"=w3595) -> ()  [unwired: 9 in, 1 out]
    }
  }
  n1714 = xnode "Read/Write Control"("FPGA VI Reference In"=w16, "error in"=w15, "FPGA_Stop"=TRUE) -> ("FPGA VI Reference Out"=w21:refnum<k20>, "error out"=w22:errorcluster)
  n1715 = xnode "Close FPGA VI Reference"("FPGA VI Reference In"=w21, "error in"=w22) -> ("error out"=w20:errorcluster)
  n1716 = call <vilib>:"Reset myRIO.vi"("error in (no error)"=w20) -> ()  [unwired: 10 in, 1 out]
